vi "HandleObservationAsync.vi"(8 "error in (no error)":errorcluster, 10 "Acquisition.lvclass In":refnum<class "Acquisition.lvclass">, 11 "S4ACS_GUI in":refnum<class "S4GUI.lvclass">) -> (0 "error out":errorcluster, 2 "Acquisition.lvclass Out":refnum<class "Acquisition.lvclass">, 3 "S4ACS_GUI out":refnum<class "S4GUI.lvclass">)   [LabVIEW 2018, in "S4GUI.lvclass"]
uses:
  S4GUI.lvclass
  Acquisition/Acquisition.lvclass
  C:/Users/devstaff/sparc4/s4gui/Versao ZeroMQ REQ-REP/SPARC4_GUI -v1.0.0 - 20241216/Server/Server.lvclass
  S4GUI.lvclass/S4GUI.ctl
  Instrument/Instrument.lvclass/Instrument.ctl
  Device/Optics/Optics.lvclass/Optics.ctl
  Interface/Interface.lvclass/Interface.ctl
  Server/Server.lvclass/Server.ctl
  Device/Optics/Opt_Selector/Opt_Selector.lvclass
  C:/Users/devstaff/sparc4/s4gui/Versao ZeroMQ REQ-REP/SPARC4_GUI -v1.0.0 - 20241216/Device/Optics/Optics.lvclass
  Instrument/Instrument.lvclass
  StateMachine/State Machine.lvclass
  SyncBox/Sync Box.lvclass
  Trigger/Trigger.lvclass
  Channel/Channel.lvclass
  Interface/Interface.lvclass
  TelFocus/TelFocus.lvclass
  SecMirror/SecMirror.lvclass
  Device/Optics/Optics.lvclass
  Server/Server.lvclass
panel:
  out "time308":u32
  out "time307":u32
  out "time9":u32
  out "delay 89":u32
  out "time 10":u32
  out "time elapsed 2":u32
  out "time 8":u32
  out "delay 78":u32
  out "time7":u32
  out "time6":u32
  out "time5":u32
  out "delay 3-4":u32
  out "time4":u32
  out "time3":u32
  out "time 2":u32
  out "time1":u32
  # "ACS DELAY"
  # "WAVEPLATE DURATION"
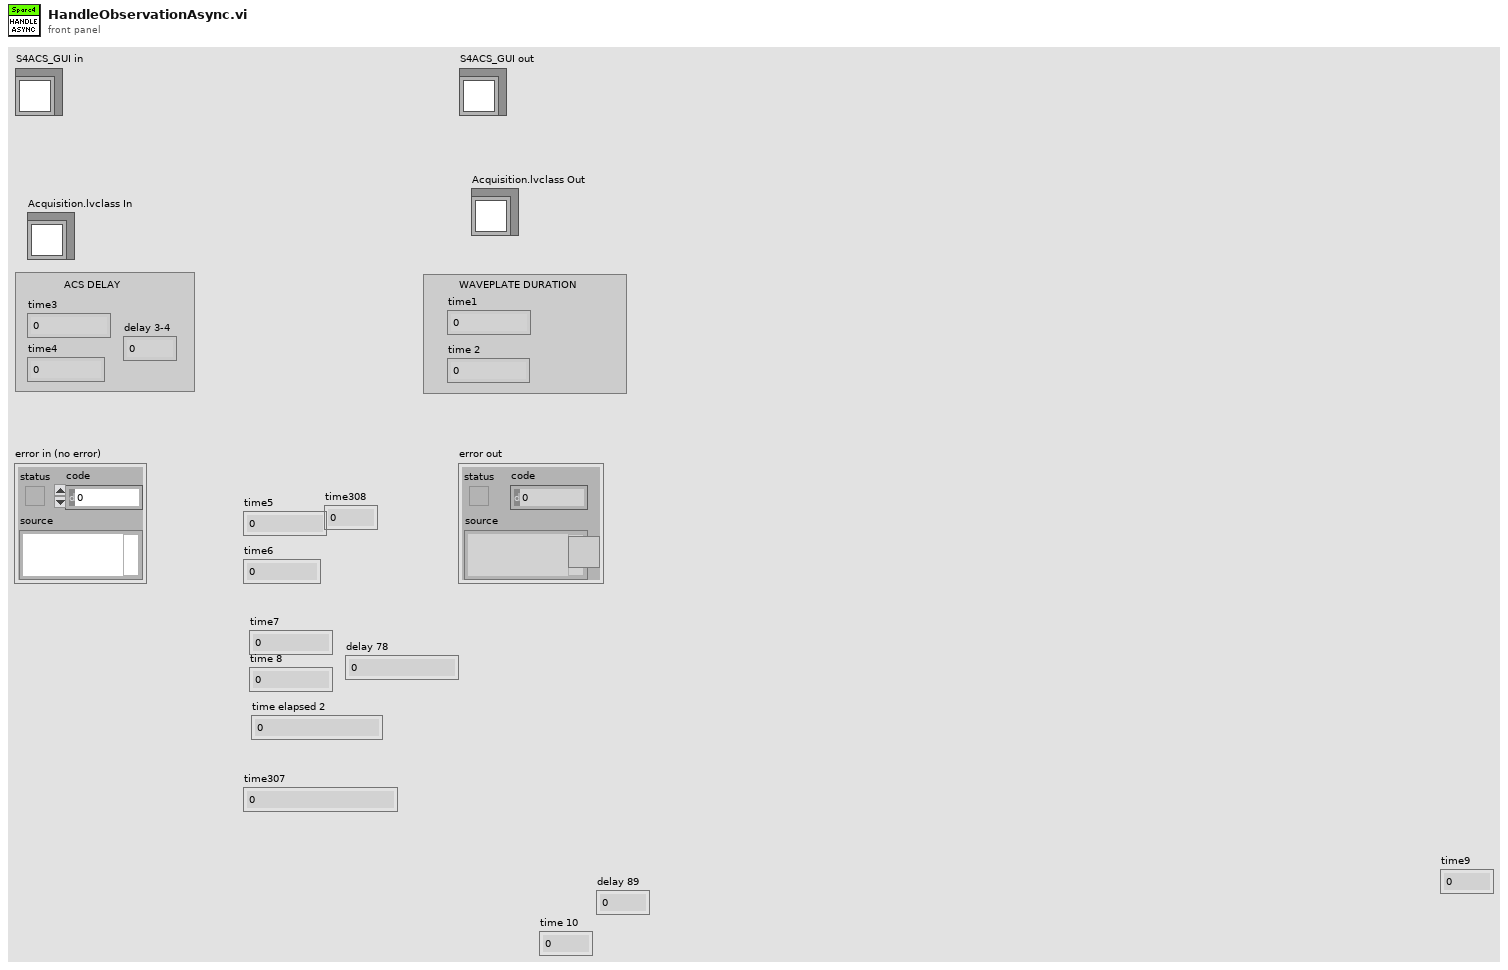
[diagram p1: front panel]
types:
  T1 = cluster{"ACQUISITION_MODE":u8, "TRIGGER_MODE":u8, "READ_MODE":u8, "PREAMP":u8, "READOUT_RATE":u8, "VERTICAL_SHIFT_SPEED":u8, "EM_MODE":u8, "EM_GAIN":u16, "SHUTTER_MODE":u8, "SHUTTER_TTL":u8, "SHUTTER_OPENING_TIME":u16, "SHUTTER_CLOSING_TIME":u16, "VBIN":u16, "HBIN":u16, "INITIAL_LINE":u16, "INITIAL_COLUMN":u16, "FINAL_LINE":u16, "FINAL_COLUMN":u16, "FRAME_TRANSFER":bool, "VERTICAL_CLOCK_VOLTAGE":u8, "AD_CHANNEL":u32}
  T2 = cluster{"Texp":dbl, "Nimages":u32, "InitialLine":u32, "FinalLine":u32, "InitialColumn":u32, "FinalColumn":u32, "EmGain":u32, "Cooler Off":bool, "CyclesDone":u32, "SequesDone":u32, "UsedDiskSpace":u16, "Error":bool}
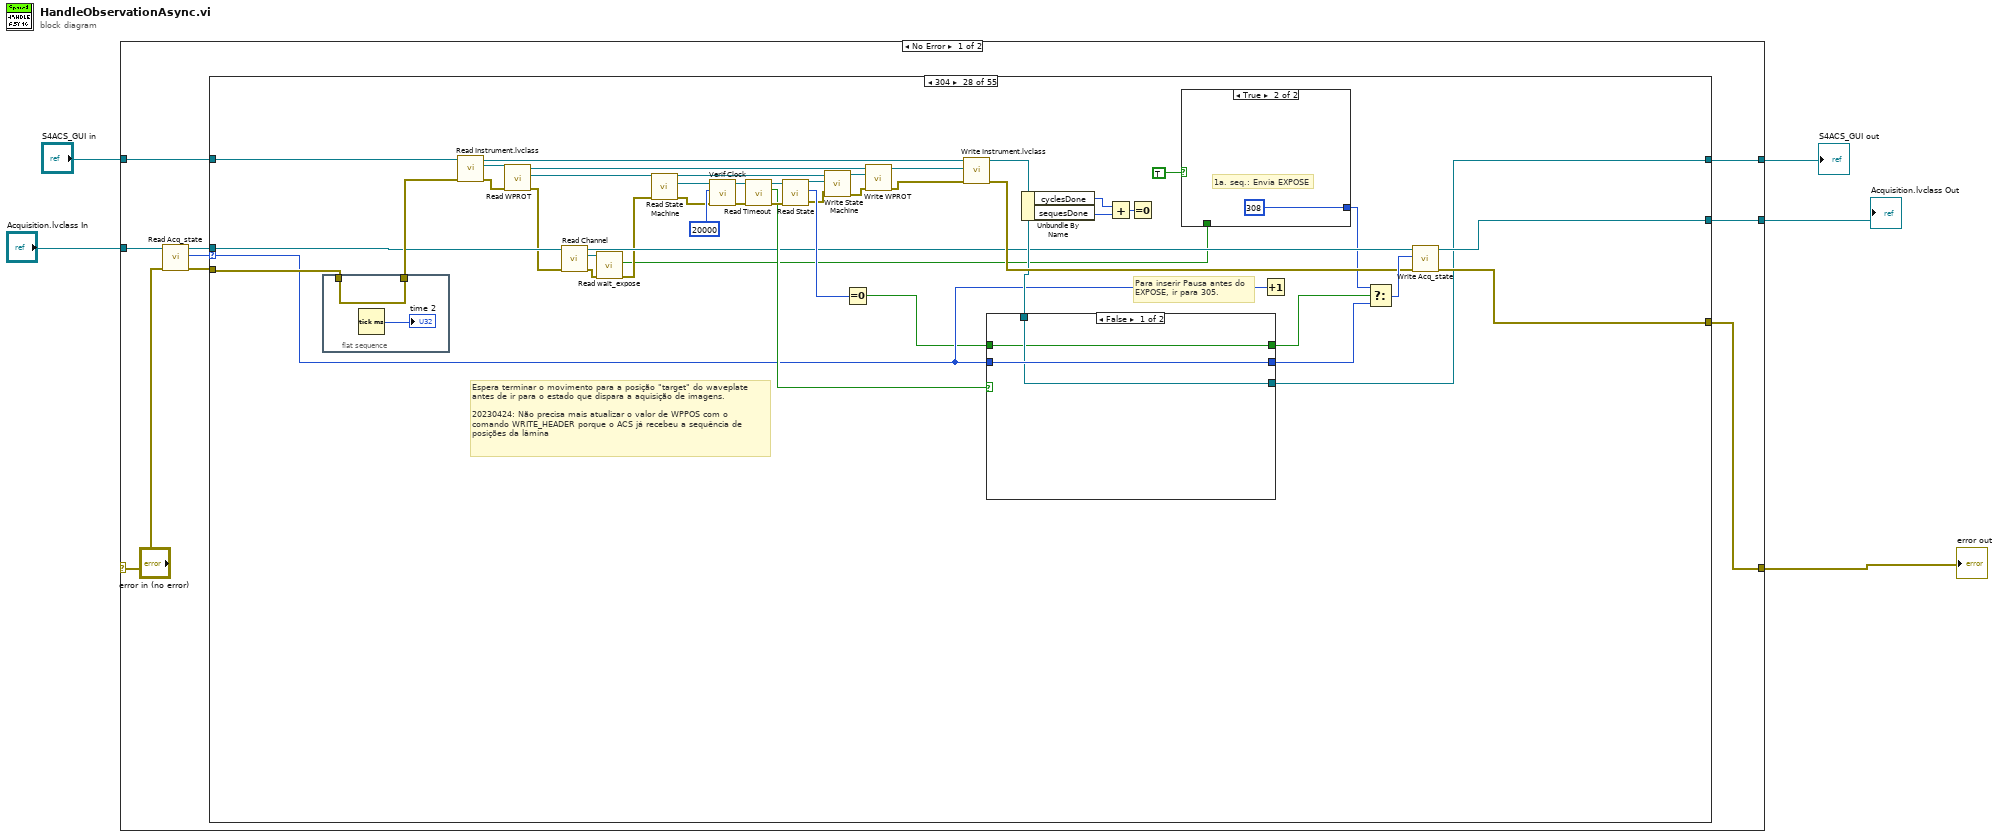
[diagram p0: block diagram]
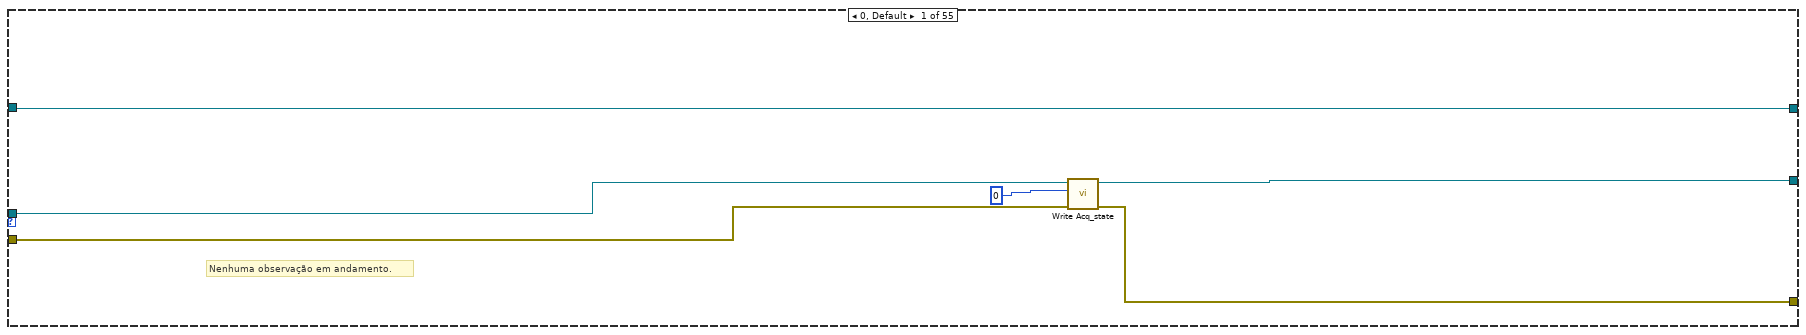
[diagram p2: hidden frame]
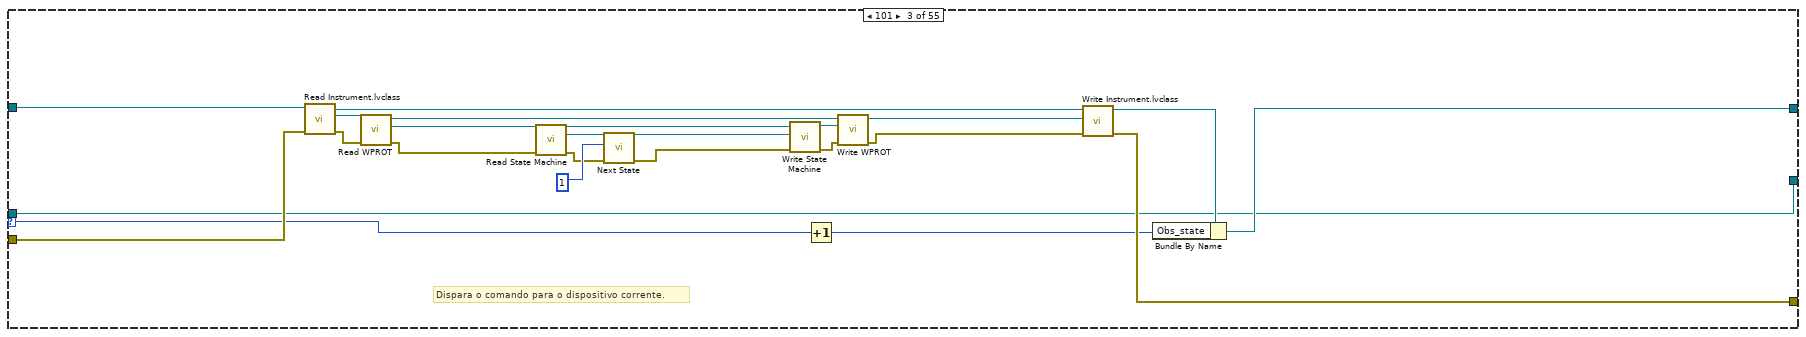
[diagram p4: hidden frame]
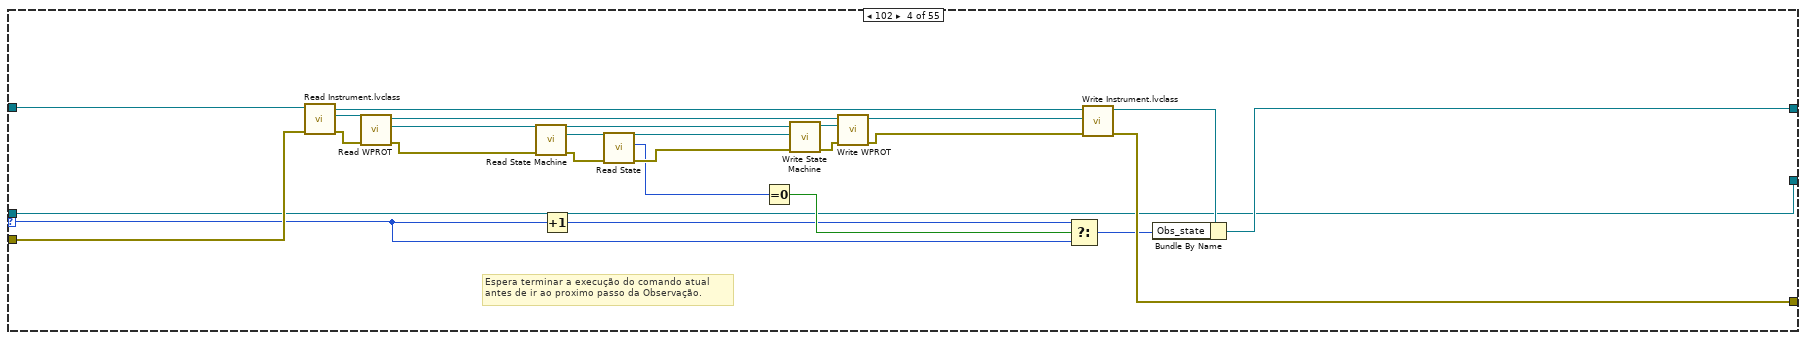
[diagram p5: hidden frame]
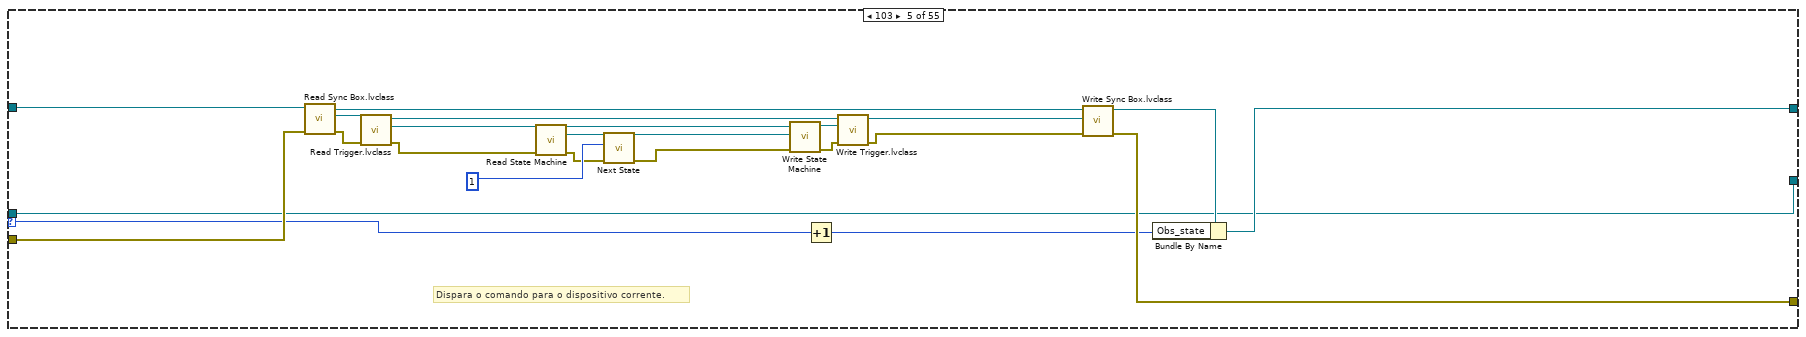
[diagram p6: hidden frame]
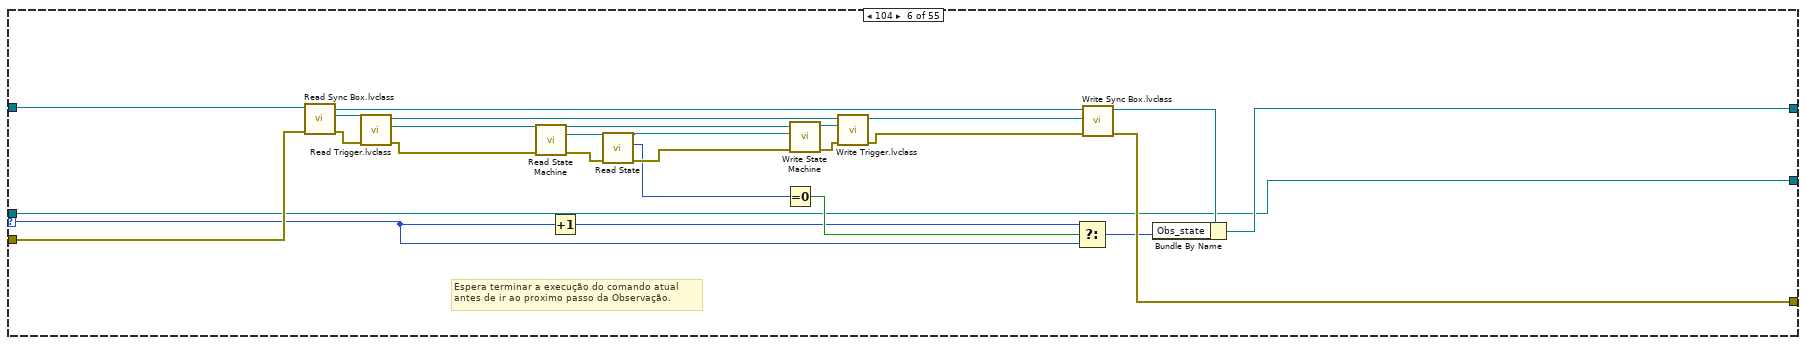
[diagram p7: hidden frame]
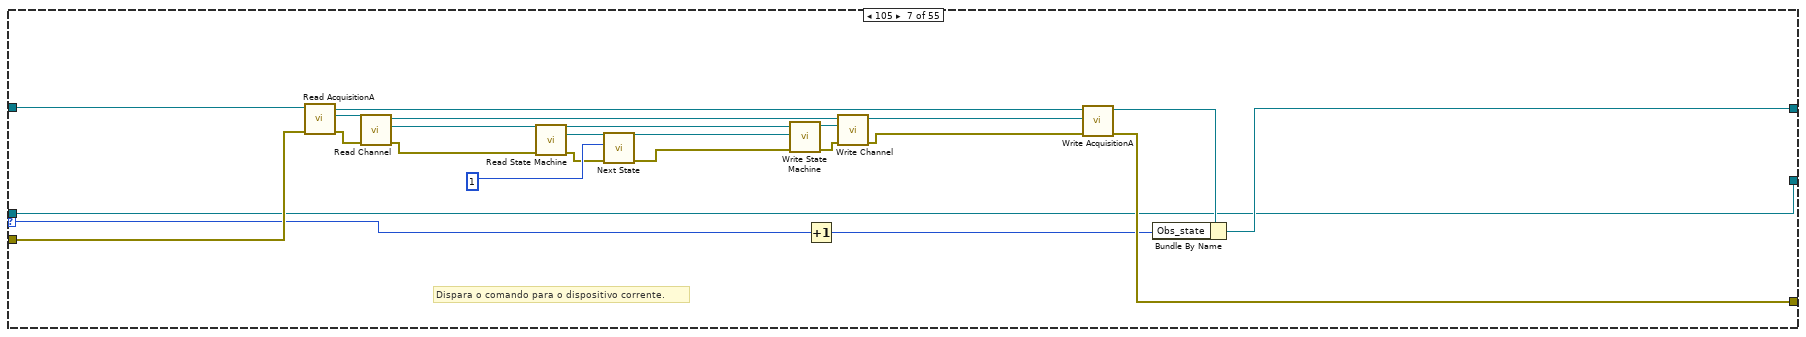
[diagram p8: hidden frame]
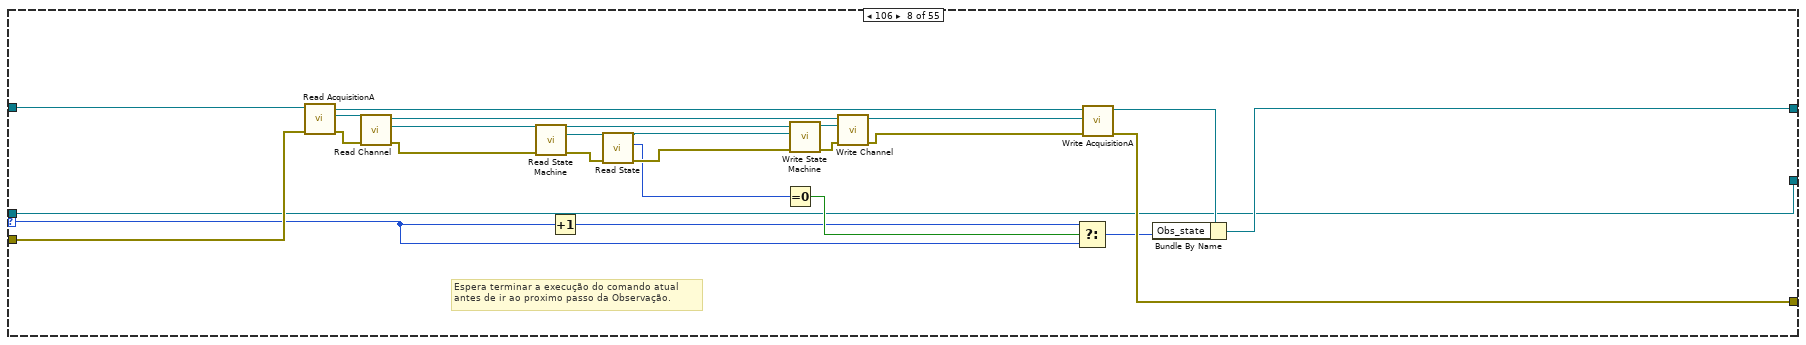
[diagram p9: hidden frame]
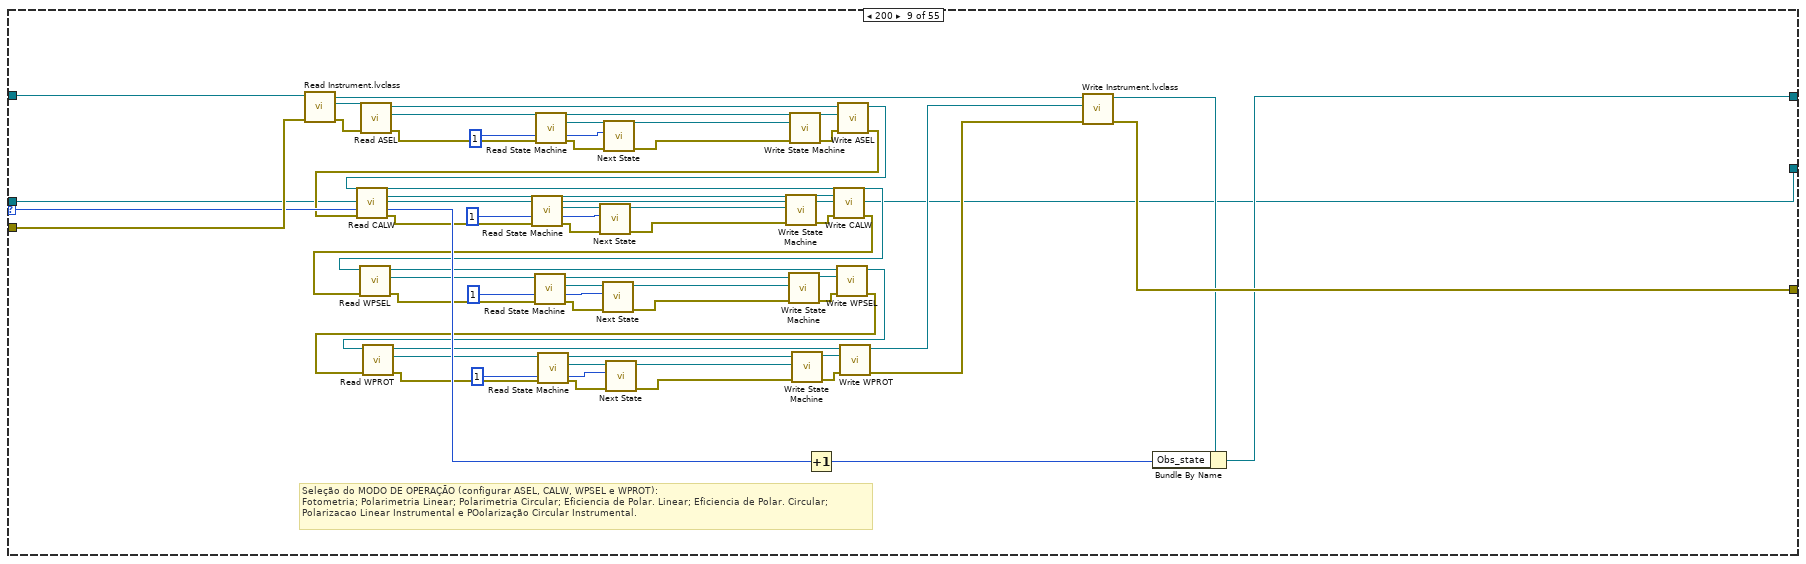
[diagram p10: hidden frame]
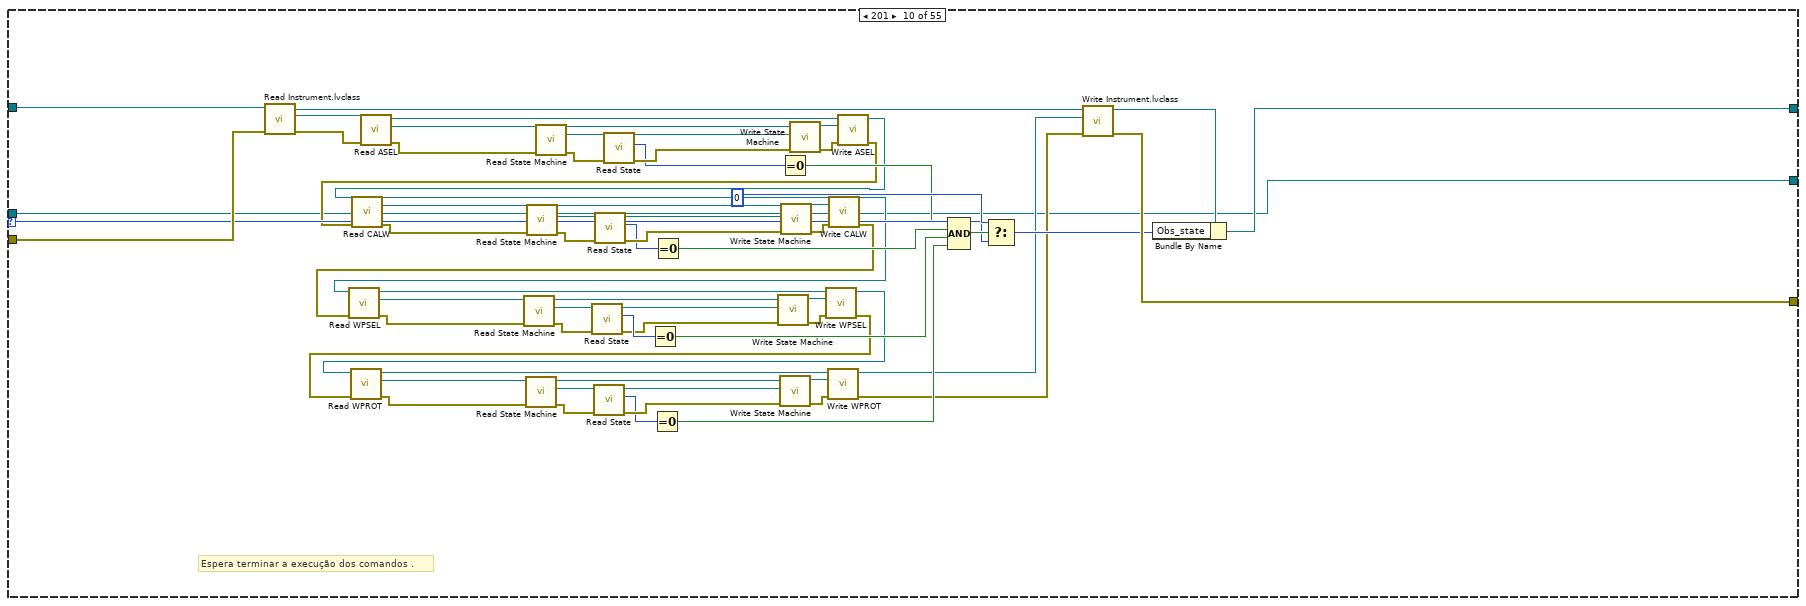
[diagram p11: hidden frame]
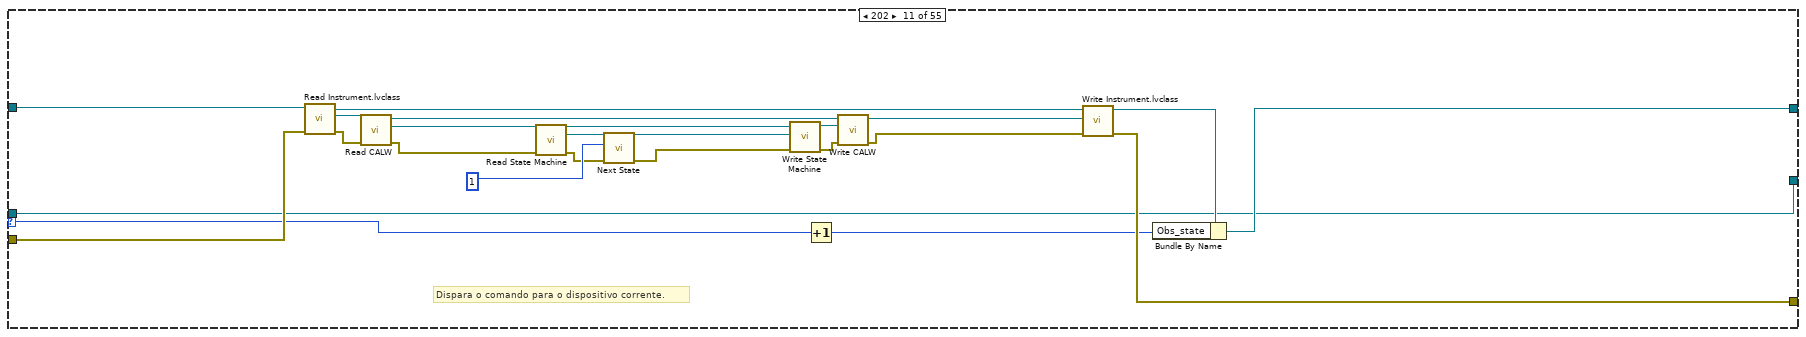
[diagram p12: hidden frame]
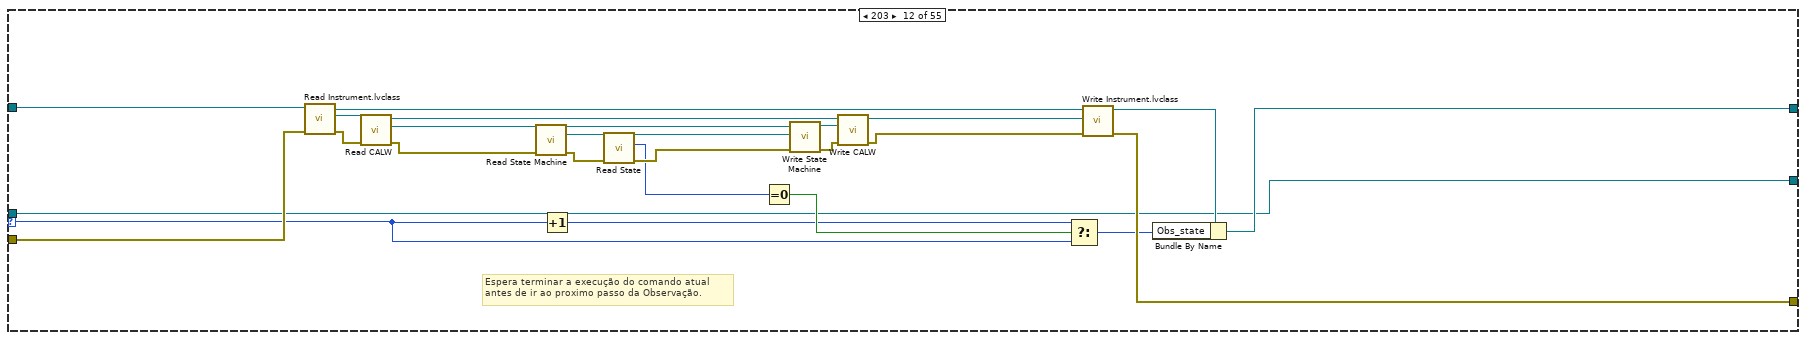
[diagram p13: hidden frame]
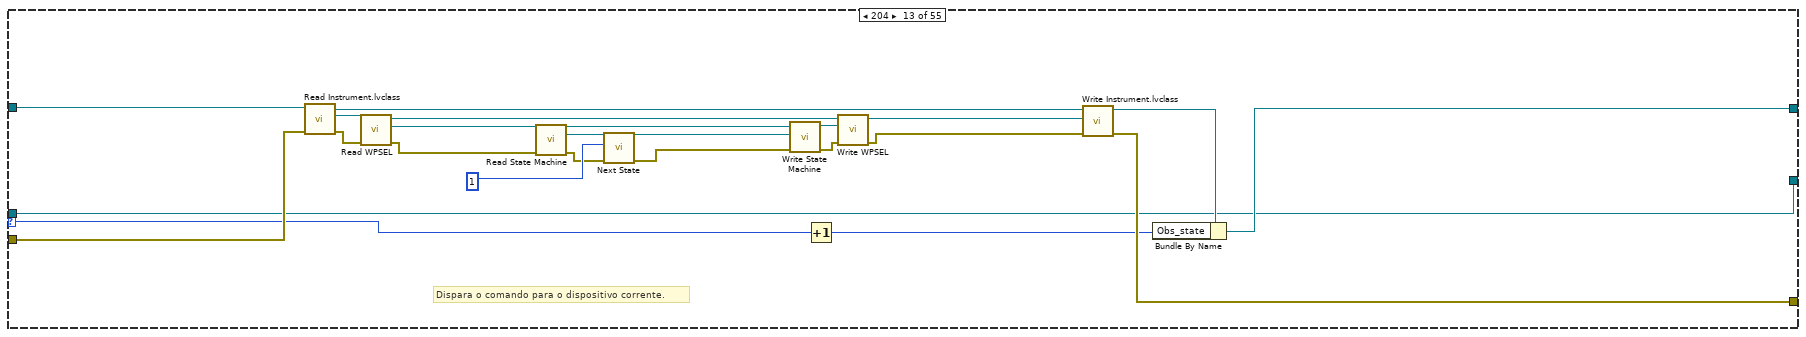
[diagram p14: hidden frame]
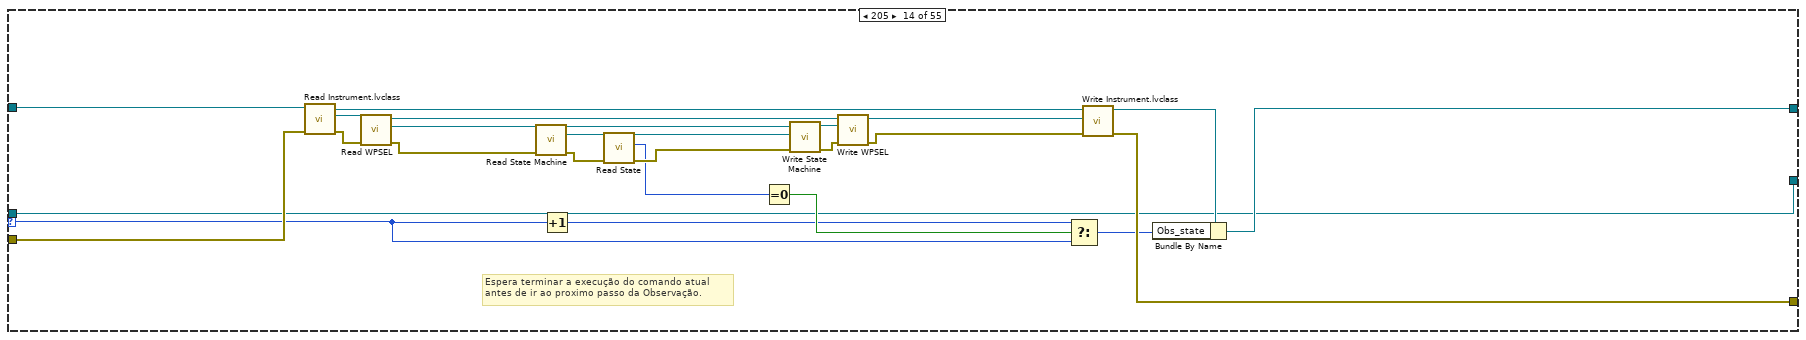
[diagram p15: hidden frame]
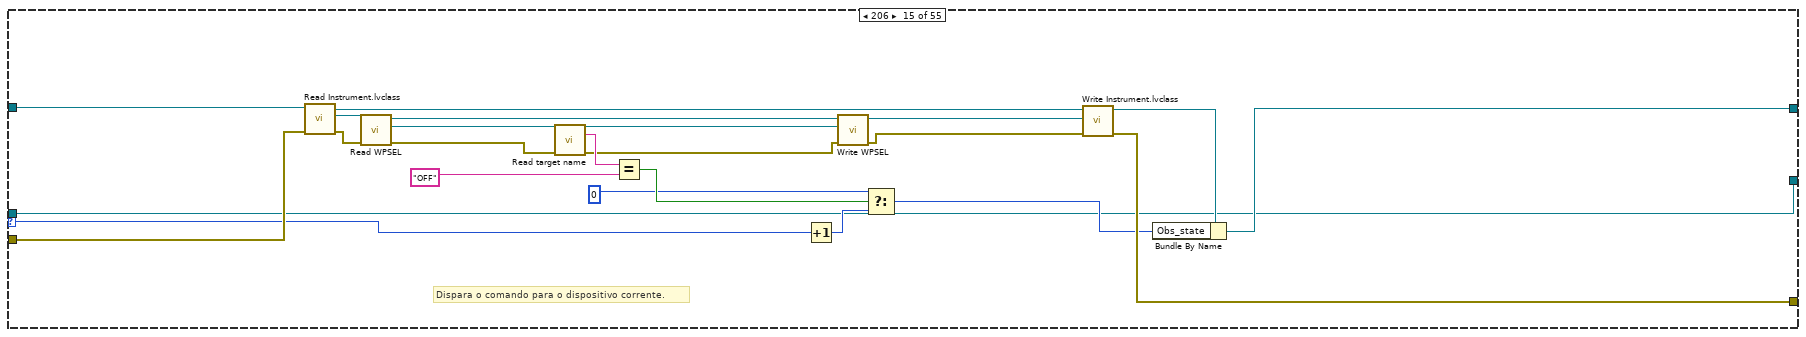
[diagram p16: hidden frame]
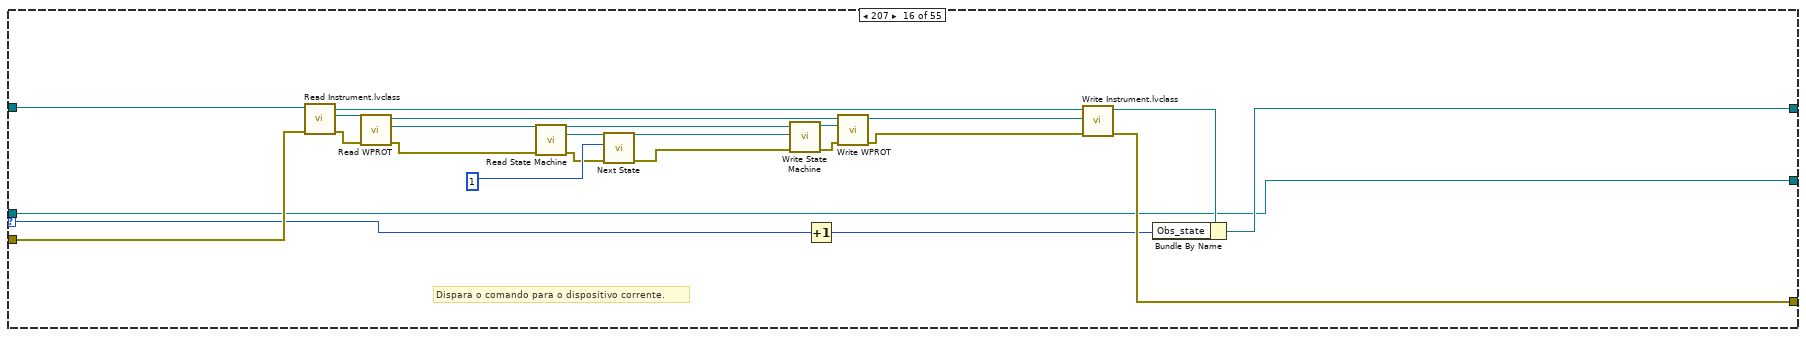
[diagram p17: hidden frame]
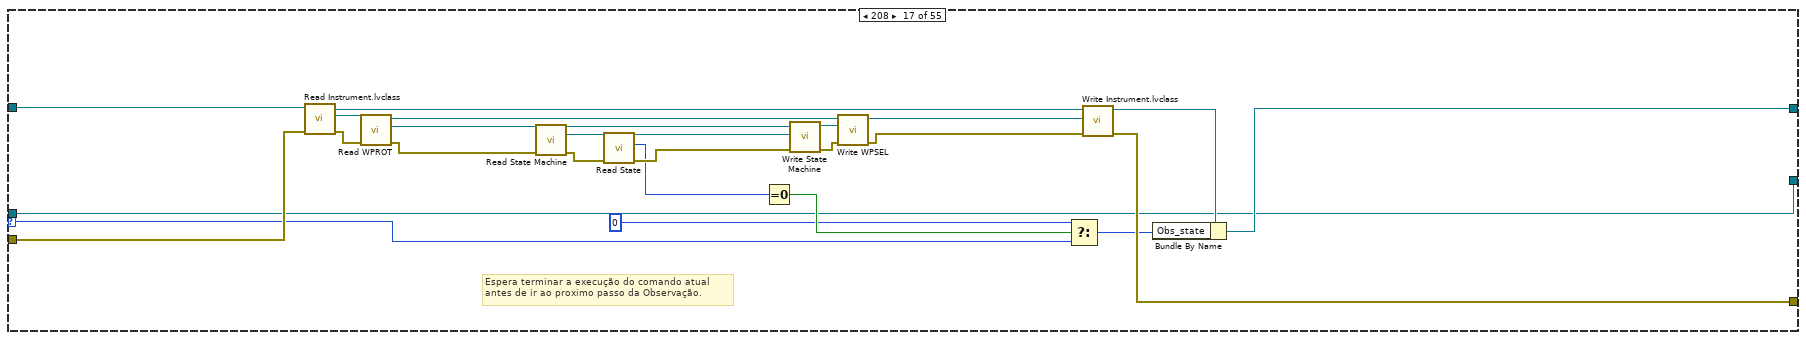
[diagram p18: hidden frame]
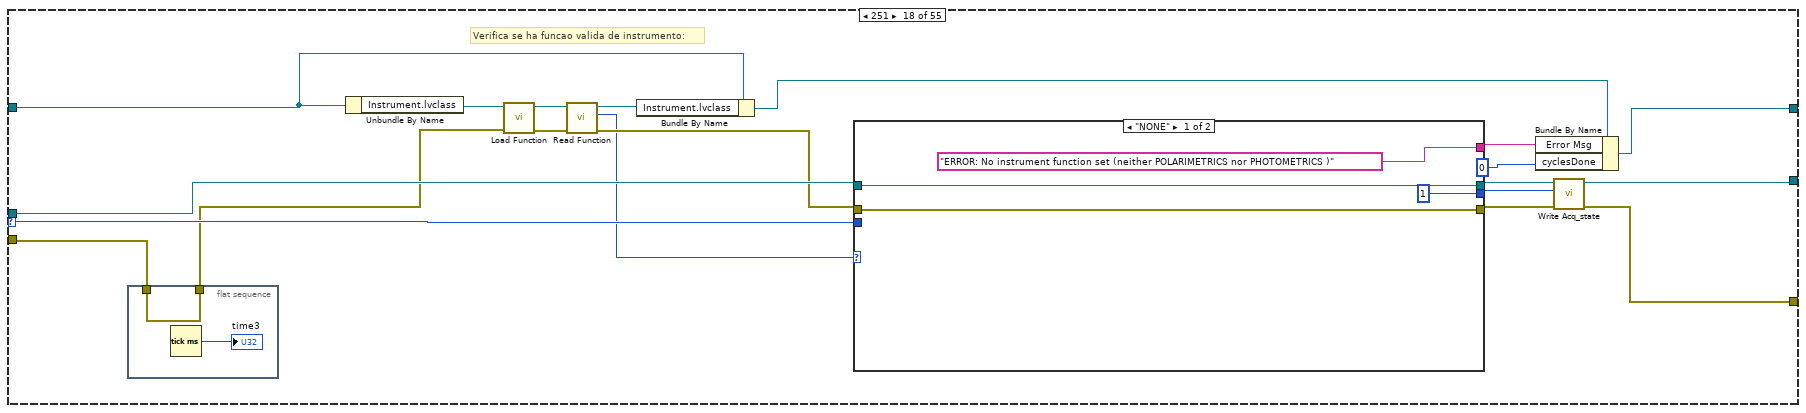
[diagram p19: hidden frame]
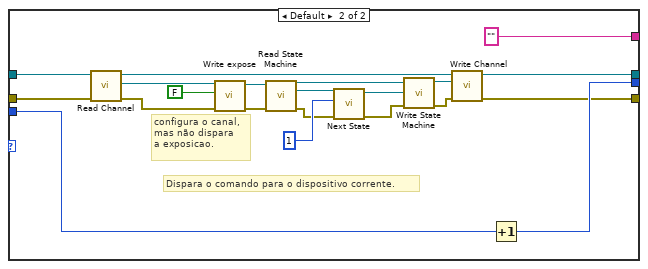
[diagram p20: hidden frame]
diagram:
  n1 = case shown="No Error" "error in (no error)" {
    selector: "error in (no error)" -> [w9 w1887]
    tunnel: [w15 w1887] -> w5
    tunnel: [w14 w1886] -> w3
    tunnel: "S4ACS_GUI in" -> [w13 w1886]
    tunnel: "Acquisition.lvclass In" -> [w12 w1885]
    tunnel: [w7 w1885] -> w1
    frame No Error {
      n2 = call-dynamic "Read Acq_state.vi"("error in (no error)"=w9, "Acquisition in"=w12) -> ("error out"=w8:errorcluster, "Acq_state"=w10:u32, "Acquisition out"=w11:refnum<class "Acquisition.lvclass">)  [unwired: 7 in]
      n3 = case shown="304" w10 {
        selector: w10 -> [_ _ w28 w51 w78 w101 w128 w151 w220 w284 w310 w333 w360 w383 w419 w433 w456 w499 w530 w603 w610 w653 w666 _ w758 w768 w824 w873 w935 w959 w1001 w1047 _ w1146 w1156 w1184 w1224 w1260 w1295 w1351 w1435 _ w1537 _ w1624 w1673 w1722 w1745 w1761 w1786 w1805 w1830 _ _ _]
        tunnel: w13 -> [w20 w24 w42 w68 w92 w118 w142 w168 w234 w302 w324 w350 w374 w400 w423 w447 w473 w484 w528 w573 w617 w634 w664 w733 w743 w767 w825 w909 w931 w949 w990 w1050 w1083 w1136 w1155 w1175 w1202 w1252 w1290 w1346 w1430 w1497 w1536 w1610 w1626 w1675 w1718 w1736 w1767 w1782 w1796 w1823 w1856 w1864 w1867]
        tunnel: [w20 w24 w26 w55 w76 w109 w126 w159 w218 w289 w308 w337 w358 w387 w418 w431 w460 w490 w527 w573 w617 w637 w663 w719 w748 w767 w791 w882 w931 w947 w980 w1049 w1082 w1134 w1155 w1174 w1201 w1254 w1289 w1347 w1431 w1493 w1536 w1610 w1623 w1659 w1718 w1740 w1767 w1782 w1800 w1823 w1851 w1864 w1869] -> w14
        tunnel: w8 -> [w19 w23 w41 w67 w91 w117 w141 w167 w233 w301 w323 w349 w373 w399 w422 w446 w472 w492 w540 w574 w611 w640 w676 w724 w742 w781 w788 w897 w936 w957 w985 w1056 w1087 w1144 w1169 w1172 w1198 w1245 w1280 w1331 w1415 w1508 w1540 w1604 w1625 w1674 w1720 w1750 w1764 w1784 w1813 w1843 w1855 w1863 w1866]
        tunnel: [w16 w23 w40 w66 w90 w116 w140 w166 w232 w300 w322 w348 w372 w398 w421 w445 w471 w493 w541 w607 w612 w641 w677 w726 w752 w779 w790 w901 w933 w952 w1004 w1054 w1084 w1139 w1167 w1178 w1222 w1255 w1300 w1334 w1418 w1513 w1538 w1611 w1617 w1655 w1711 w1746 w1765 w1778 w1809 w1839 w1849 w1863 w1868] -> w15
        tunnel: w11 -> [w18 w22 w25 w49 w75 w99 w125 w149 w175 w238 w307 w331 w357 w381 w407 w430 w454 w498 w545 w606 w618 w645 w681 w718 w757 w782 w793 w881 w937 w958 w971 w1057 w1086 w1145 w1170 w1183 w1200 w1250 w1283 w1332 w1416 w1509 w1541 w1605 w1621 w1658 w1721 w1751 w1762 w1785 w1814 w1844 w1854 w1862 w1865]
        tunnel: [w17 w22 w25 w49 w75 w99 w125 w149 w175 w238 w307 w331 w357 w381 w407 w430 w454 w495 w542 w608 w613 w642 w678 w725 w753 w780 w789 w900 w932 w953 w1005 w1055 w1085 w1140 w1168 w1182 w1223 w1259 w1301 w1350 w1434 w1514 w1539 w1612 w1620 w1656 w1715 w1747 w1766 w1779 w1810 w1840 w1850 w1862 w1865] -> w7
        frame 0, Default {
          # "Nenhuma observação em andamento."
          n4 = call-dynamic "Write Acq_state.vi"("error in (no error)"=w19, "Acq_state"=u32 0 ("Obs_state"), "Acquisition in"=w18) -> ("error out"=w16:errorcluster, "Acquisition out"=w17:refnum<class "Acquisition.lvclass">)  [unwired: 7 in]
        }
        frame 1 {
          # "Estado de erro!\nFica aqui até acionar STOP ou ABORT."
          # "Nenhuma observação em andamento."
        }
        frame 101 {
          # "Dispara o comando para o dispositivo corrente."
          n5 = call "Read Instrument.lvclass.vi"("error in (no error)"=w41, "S4ACS_GUI in"=w42) -> ("error out"=w47:errorcluster, "Instrument.lvclass"=w48:refnum<class "Instrument.lvclass">, "S4ACS_GUI out"=w44:refnum<class "S4GUI.lvclass">)  [unwired: 7 in]
          n6 = call "Read WPROT.vi"("error in (no error)"=w47, "Instrument in"=w48) -> ("error out"=w34:errorcluster, "Opt_Selector.lvclass"=w33:refnum<class "Opt_Selector.lvclass">, "Instrument out"=w46:refnum<class "Instrument.lvclass">)  [unwired: 7 in]
          n7 = call-dynamic "Read State Machine.vi"("error in (no error)"=w34, "Device in"=w33) -> ("error out"=w37:errorcluster, "State Machine.lvclass"=w39:refnum<class "State Machine.lvclass">, "Device out"=w31:refnum<class "Opt_Selector.lvclass">)  [unwired: 7 in]
          n8 = call "Next State.vi"("error in (no error)"=w37, "New_State"=1, "State Machine in"=w39) -> ("error out"=w36:errorcluster, "State Machine out"=w35:refnum<class "State Machine.lvclass">)  [unwired: 7 in]
          n9 = call-dynamic "Write State Machine.vi"("error in (no error)"=w36, "State Machine.lvclass"=w35, "Device in"=w31) -> ("error out"=w30:errorcluster, "Device out"=w32:refnum<class "Opt_Selector.lvclass">)  [unwired: 7 in]
          n10 = Increment(x=w28) -> (x+1=w27:u32)
          n11 = call "Write WPROT.vi"("error in (no error)"=w30, "Opt_Selector.lvclass"=w32, "Instrument in"=w46) -> ("error out"=w43:errorcluster, "Instrument out"=w45:refnum<class "Instrument.lvclass">)  [unwired: 7 in]
          n12 = call "Write Instrument.lvclass.vi"("error in (no error)"=w43, "Instrument.lvclass"=w45, "S4ACS_GUI in"=w44) -> ("error out"=w40:errorcluster, "S4ACS_GUI out"=w29:refnum<class "S4GUI.lvclass">)  [unwired: 7 in]
          n13 = Bundle By Name(cluster=w29, "Obs_state"=w27) -> (w26:refnum<class "S4GUI.lvclass">)
        }
        frame 102 {
          # "Espera terminar a execução do comando atual \nantes de ir ao proximo passo da Observação."
          n14 = call "Read Instrument.lvclass.vi"("error in (no error)"=w67, "S4ACS_GUI in"=w68) -> ("error out"=w73:errorcluster, "Instrument.lvclass"=w74:refnum<class "Instrument.lvclass">, "S4ACS_GUI out"=w70:refnum<class "S4GUI.lvclass">)  [unwired: 7 in]
          n15 = call "Read WPROT.vi"("error in (no error)"=w73, "Instrument in"=w74) -> ("error out"=w61:errorcluster, "Opt_Selector.lvclass"=w60:refnum<class "Opt_Selector.lvclass">, "Instrument out"=w72:refnum<class "Instrument.lvclass">)  [unwired: 7 in]
          n16 = call-dynamic "Read State Machine.vi"("error in (no error)"=w61, "Device in"=w60) -> ("error out"=w64:errorcluster, "State Machine.lvclass"=w65:refnum<class "State Machine.lvclass">, "Device out"=w58:refnum<class "Opt_Selector.lvclass">)  [unwired: 7 in]
          n17 = Increment(x=w51) -> (x+1=w50:u32)
          n18 = call-dynamic "Read State.vi"("error in (no error)"=w64, "State Machine in"=w65) -> ("error out"=w63:errorcluster, "State"=w53:i32, "State Machine out"=w62:refnum<class "State Machine.lvclass">)  [unwired: 7 in]
          n19 = Equal To 0?(x=w53) -> (x = 0?=w54:bool)
          n20 = call-dynamic "Write State Machine.vi"("error in (no error)"=w63, "State Machine.lvclass"=w62, "Device in"=w58) -> ("error out"=w57:errorcluster, "Device out"=w59:refnum<class "Opt_Selector.lvclass">)  [unwired: 7 in]
          n21 = call "Write WPROT.vi"("error in (no error)"=w57, "Opt_Selector.lvclass"=w59, "Instrument in"=w72) -> ("error out"=w69:errorcluster, "Instrument out"=w71:refnum<class "Instrument.lvclass">)  [unwired: 7 in]
          n22 = Select(t=w50, s=w54, f=w51) -> (s? t:f=w52:u32)
          n23 = call "Write Instrument.lvclass.vi"("error in (no error)"=w69, "Instrument.lvclass"=w71, "S4ACS_GUI in"=w70) -> ("error out"=w66:errorcluster, "S4ACS_GUI out"=w56:refnum<class "S4GUI.lvclass">)  [unwired: 7 in]
          n24 = Bundle By Name(cluster=w56, "Obs_state"=w52) -> (w55:refnum<class "S4GUI.lvclass">)
        }
        frame 103 {
          # "Dispara o comando para o dispositivo corrente."
          n25 = call-dynamic "Read Sync Box.lvclass.vi"("error in (no error)"=w91, "SPARC4_AC in"=w92) -> ("error out"=w97:errorcluster, "Sync Box.lvclass"=w98:refnum<class "Sync Box.lvclass">, "SPARC4_AC out"=w94:refnum<class "S4GUI.lvclass">)  [unwired: 7 in]
          n26 = call-dynamic "Read Trigger.lvclass.vi"("error in (no error)"=w97, "Sync Box in"=w98) -> ("error out"=w84:errorcluster, "Trigger.lvclass"=w83:refnum<class "Trigger.lvclass">, "Sync Box out"=w96:refnum<class "Sync Box.lvclass">)  [unwired: 7 in]
          n27 = call-dynamic "Read State Machine.vi"("error in (no error)"=w84, "Device in"=w83) -> ("error out"=w87:errorcluster, "State Machine.lvclass"=w89:refnum<class "State Machine.lvclass">, "Device out"=w81:refnum<class "Trigger.lvclass">)  [unwired: 7 in]
          n28 = call "Next State.vi"("error in (no error)"=w87, "New_State"=1, "State Machine in"=w89) -> ("error out"=w86:errorcluster, "State Machine out"=w85:refnum<class "State Machine.lvclass">)  [unwired: 7 in]
          n29 = call-dynamic "Write State Machine.vi"("error in (no error)"=w86, "State Machine.lvclass"=w85, "Device in"=w81) -> ("error out"=w80:errorcluster, "Device out"=w82:refnum<class "Trigger.lvclass">)  [unwired: 7 in]
          n30 = Increment(x=w78) -> (x+1=w77:u32)
          n31 = call-dynamic "Write Trigger.lvclass.vi"("error in (no error)"=w80, "Trigger.lvclass"=w82, "Sync Box in"=w96) -> ("error out"=w93:errorcluster, "Sync Box out"=w95:refnum<class "Sync Box.lvclass">)  [unwired: 7 in]
          n32 = call-dynamic "Write Sync Box.lvclass.vi"("error in (no error)"=w93, "Sync Box.lvclass"=w95, "SPARC4_AC in"=w94) -> ("error out"=w90:errorcluster, "SPARC4_AC out"=w79:refnum<class "S4GUI.lvclass">)  [unwired: 7 in]
          n33 = Bundle By Name(cluster=w79, "Obs_state"=w77) -> (w76:refnum<class "S4GUI.lvclass">)
        }
        frame 104 {
          # "Espera terminar a execução do comando atual \nantes de ir ao proximo passo da Observação."
          n34 = call-dynamic "Read Sync Box.lvclass.vi"("error in (no error)"=w117, "SPARC4_AC in"=w118) -> ("error out"=w123:errorcluster, "Sync Box.lvclass"=w124:refnum<class "Sync Box.lvclass">, "SPARC4_AC out"=w120:refnum<class "S4GUI.lvclass">)  [unwired: 7 in]
          n35 = call-dynamic "Read Trigger.lvclass.vi"("error in (no error)"=w123, "Sync Box in"=w124) -> ("error out"=w115:errorcluster, "Trigger.lvclass"=w114:refnum<class "Trigger.lvclass">, "Sync Box out"=w122:refnum<class "Sync Box.lvclass">)  [unwired: 7 in]
          n36 = call-dynamic "Read State Machine.vi"("error in (no error)"=w115, "Device in"=w114) -> ("error out"=w106:errorcluster, "State Machine.lvclass"=w108:refnum<class "State Machine.lvclass">, "Device out"=w112:refnum<class "Trigger.lvclass">)  [unwired: 7 in]
          n37 = Increment(x=w101) -> (x+1=w103:u32)
          n38 = call-dynamic "Read State.vi"("error in (no error)"=w106, "State Machine in"=w108) -> ("error out"=w105:errorcluster, "State"=w100:i32, "State Machine out"=w107:refnum<class "State Machine.lvclass">)  [unwired: 7 in]
          n39 = Equal To 0?(x=w100) -> (x = 0?=w104:bool)
          n40 = call-dynamic "Write State Machine.vi"("error in (no error)"=w105, "State Machine.lvclass"=w107, "Device in"=w112) -> ("error out"=w111:errorcluster, "Device out"=w113:refnum<class "Trigger.lvclass">)  [unwired: 7 in]
          n41 = call-dynamic "Write Trigger.lvclass.vi"("error in (no error)"=w111, "Trigger.lvclass"=w113, "Sync Box in"=w122) -> ("error out"=w119:errorcluster, "Sync Box out"=w121:refnum<class "Sync Box.lvclass">)  [unwired: 7 in]
          n42 = Select(t=w103, s=w104, f=w101) -> (s? t:f=w102:u32)
          n43 = call-dynamic "Write Sync Box.lvclass.vi"("error in (no error)"=w119, "Sync Box.lvclass"=w121, "SPARC4_AC in"=w120) -> ("error out"=w116:errorcluster, "SPARC4_AC out"=w110:refnum<class "S4GUI.lvclass">)  [unwired: 7 in]
          n44 = Bundle By Name(cluster=w110, "Obs_state"=w102) -> (w109:refnum<class "S4GUI.lvclass">)
        }
        frame 105 {
          # "Dispara o comando para o dispositivo corrente."
          n45 = call-dynamic "Read AcquisitionA.vi"("error in (no error)"=w141, "S4ACS_GUI in"=w142) -> ("error out"=w147:errorcluster, "Acquisition.lvclass"=w148:refnum<class "Acquisition.lvclass">, "S4ACS_GUI out"=w144:refnum<class "S4GUI.lvclass">)  [unwired: 7 in]
          n46 = call-dynamic "Read Channel.vi"("error in (no error)"=w147, "Acquisition in"=w148) -> ("error out"=w134:errorcluster, "Channel.lvclass"=w133:refnum<class "Channel.lvclass">, "Acquisition out"=w146:refnum<class "Acquisition.lvclass">)  [unwired: 7 in]
          n47 = call-dynamic "Read State Machine.vi"("error in (no error)"=w134, "Device in"=w133) -> ("error out"=w137:errorcluster, "State Machine.lvclass"=w139:refnum<class "State Machine.lvclass">, "Device out"=w131:refnum<class "Channel.lvclass">)  [unwired: 7 in]
          n48 = call "Next State.vi"("error in (no error)"=w137, "New_State"=1, "State Machine in"=w139) -> ("error out"=w136:errorcluster, "State Machine out"=w135:refnum<class "State Machine.lvclass">)  [unwired: 7 in]
          n49 = call-dynamic "Write State Machine.vi"("error in (no error)"=w136, "State Machine.lvclass"=w135, "Device in"=w131) -> ("error out"=w130:errorcluster, "Device out"=w132:refnum<class "Channel.lvclass">)  [unwired: 7 in]
          n50 = Increment(x=w128) -> (x+1=w127:u32)
          n51 = call-dynamic "Write Channel.vi"("error in (no error)"=w130, "Channel.lvclass"=w132, "Acquisition in"=w146) -> ("error out"=w143:errorcluster, "Acquisition out"=w145:refnum<class "Acquisition.lvclass">)  [unwired: 7 in]
          n52 = call-dynamic "Write AcquisitionA.vi"("error in (no error)"=w143, "Acquisition.lvclass"=w145, "S4ACS_GUI in"=w144) -> ("error out"=w140:errorcluster, "S4ACS_GUI out"=w129:refnum<class "S4GUI.lvclass">)  [unwired: 7 in]
          n53 = Bundle By Name(cluster=w129, "Obs_state"=w127) -> (w126:refnum<class "S4GUI.lvclass">)
        }
        frame 106 {
          # "Espera terminar a execução do comando atual \nantes de ir ao proximo passo da Observação."
          n54 = call-dynamic "Read AcquisitionA.vi"("error in (no error)"=w167, "S4ACS_GUI in"=w168) -> ("error out"=w173:errorcluster, "Acquisition.lvclass"=w174:refnum<class "Acquisition.lvclass">, "S4ACS_GUI out"=w170:refnum<class "S4GUI.lvclass">)  [unwired: 7 in]
          n55 = call-dynamic "Read Channel.vi"("error in (no error)"=w173, "Acquisition in"=w174) -> ("error out"=w165:errorcluster, "Channel.lvclass"=w164:refnum<class "Channel.lvclass">, "Acquisition out"=w172:refnum<class "Acquisition.lvclass">)  [unwired: 7 in]
          n56 = call-dynamic "Read State Machine.vi"("error in (no error)"=w165, "Device in"=w164) -> ("error out"=w156:errorcluster, "State Machine.lvclass"=w158:refnum<class "State Machine.lvclass">, "Device out"=w162:refnum<class "Channel.lvclass">)  [unwired: 7 in]
          n57 = Increment(x=w151) -> (x+1=w153:u32)
          n58 = call-dynamic "Read State.vi"("error in (no error)"=w156, "State Machine in"=w158) -> ("error out"=w155:errorcluster, "State"=w150:i32, "State Machine out"=w157:refnum<class "State Machine.lvclass">)  [unwired: 7 in]
          n59 = Equal To 0?(x=w150) -> (x = 0?=w154:bool)
          n60 = call-dynamic "Write State Machine.vi"("error in (no error)"=w155, "State Machine.lvclass"=w157, "Device in"=w162) -> ("error out"=w161:errorcluster, "Device out"=w163:refnum<class "Channel.lvclass">)  [unwired: 7 in]
          n61 = call-dynamic "Write Channel.vi"("error in (no error)"=w161, "Channel.lvclass"=w163, "Acquisition in"=w172) -> ("error out"=w169:errorcluster, "Acquisition out"=w171:refnum<class "Acquisition.lvclass">)  [unwired: 7 in]
          n62 = Select(t=w153, s=w154, f=w151) -> (s? t:f=w152:u32)
          n63 = call-dynamic "Write AcquisitionA.vi"("error in (no error)"=w169, "Acquisition.lvclass"=w171, "S4ACS_GUI in"=w170) -> ("error out"=w166:errorcluster, "S4ACS_GUI out"=w160:refnum<class "S4GUI.lvclass">)  [unwired: 7 in]
          n64 = Bundle By Name(cluster=w160, "Obs_state"=w152) -> (w159:refnum<class "S4GUI.lvclass">)
        }
        frame 200 {
          # "Seleção do MODO DE OPERAÇÃO (configurar ASEL, CALW, WPSEL e WPROT): \nFotometria; Polarimetria Linear; Polarimetria Circular; Eficiencia de Polar. Linear; Eficiencia de Polar. Circular;\nPolarizacao Linear Instrumental e POolarização Circular Instrumental."
          n65 = call "Read Instrument.lvclass.vi"("error in (no error)"=w233, "S4ACS_GUI in"=w234) -> ("error out"=w237:errorcluster, "Instrument.lvclass"=w197:refnum<class "Instrument.lvclass">, "S4ACS_GUI out"=w235:refnum<class "S4GUI.lvclass">)  [unwired: 7 in]
          n66 = call "Read ASEL.vi"("error in (no error)"=w237, "Instrument in"=w197) -> ("error out"=w226:errorcluster, "Opt_Selector.lvclass"=w225:refnum<class "Opt_Selector.lvclass">, "Instrument out"=w236:refnum<class "Instrument.lvclass">)  [unwired: 7 in]
          n67 = call-dynamic "Read State Machine.vi"("error in (no error)"=w226, "Device in"=w225) -> ("error out"=w229:errorcluster, "State Machine.lvclass"=w231:refnum<class "State Machine.lvclass">, "Device out"=w223:refnum<class "Opt_Selector.lvclass">)  [unwired: 7 in]
          n68 = call "Next State.vi"("error in (no error)"=w229, "New_State"=1, "State Machine in"=w231) -> ("error out"=w228:errorcluster, "State Machine out"=w227:refnum<class "State Machine.lvclass">)  [unwired: 7 in]
          n69 = call-dynamic "Write State Machine.vi"("error in (no error)"=w228, "State Machine.lvclass"=w227, "Device in"=w223) -> ("error out"=w222:errorcluster, "Device out"=w224:refnum<class "Opt_Selector.lvclass">)  [unwired: 7 in]
          n70 = Increment(x=w220) -> (x+1=w219:u32)
          n71 = call "Write ASEL.vi"("error in (no error)"=w222, "Opt_Selector.lvclass"=w224, "Instrument in"=w236) -> ("error out"=w178:errorcluster, "Instrument out"=w196:refnum<class "Instrument.lvclass">)  [unwired: 7 in]
          n72 = call "Read CALW.vi"("error in (no error)"=w178, "Instrument in"=w196) -> ("error out"=w213:errorcluster, "Opt_Selector.lvclass"=w214:refnum<class "Opt_Selector.lvclass">, "Instrument out"=w195:refnum<class "Instrument.lvclass">)  [unwired: 7 in]
          n73 = call-dynamic "Read State Machine.vi"("error in (no error)"=w213, "Device in"=w214) -> ("error out"=w210:errorcluster, "State Machine.lvclass"=w208:refnum<class "State Machine.lvclass">, "Device out"=w216:refnum<class "Opt_Selector.lvclass">)  [unwired: 7 in]
          n74 = call "Next State.vi"("error in (no error)"=w210, "New_State"=1, "State Machine in"=w208) -> ("error out"=w211:errorcluster, "State Machine out"=w212:refnum<class "State Machine.lvclass">)  [unwired: 7 in]
          n75 = call-dynamic "Write State Machine.vi"("error in (no error)"=w211, "State Machine.lvclass"=w212, "Device in"=w216) -> ("error out"=w217:errorcluster, "Device out"=w215:refnum<class "Opt_Selector.lvclass">)  [unwired: 7 in]
          n76 = call "Write CALW.vi"("error in (no error)"=w217, "Opt_Selector.lvclass"=w215, "Instrument in"=w195) -> ("error out"=w177:errorcluster, "Instrument out"=w194:refnum<class "Instrument.lvclass">)  [unwired: 7 in]
          n77 = call "Read WPSEL.vi"("error in (no error)"=w177, "Instrument in"=w194) -> ("error out"=w202:errorcluster, "Opt_Selector.lvclass"=w201:refnum<class "Opt_Selector.lvclass">, "Instrument out"=w193:refnum<class "Instrument.lvclass">)  [unwired: 7 in]
          n78 = call-dynamic "Read State Machine.vi"("error in (no error)"=w202, "Device in"=w201) -> ("error out"=w205:errorcluster, "State Machine.lvclass"=w207:refnum<class "State Machine.lvclass">, "Device out"=w199:refnum<class "Opt_Selector.lvclass">)  [unwired: 7 in]
          n79 = call "Next State.vi"("error in (no error)"=w205, "New_State"=1, "State Machine in"=w207) -> ("error out"=w204:errorcluster, "State Machine out"=w203:refnum<class "State Machine.lvclass">)  [unwired: 7 in]
          n80 = call-dynamic "Write State Machine.vi"("error in (no error)"=w204, "State Machine.lvclass"=w203, "Device in"=w199) -> ("error out"=w198:errorcluster, "Device out"=w200:refnum<class "Opt_Selector.lvclass">)  [unwired: 7 in]
          n81 = call "Write WPSEL.vi"("error in (no error)"=w198, "Opt_Selector.lvclass"=w200, "Instrument in"=w193) -> ("error out"=w176:errorcluster, "Instrument out"=w182:refnum<class "Instrument.lvclass">)  [unwired: 7 in]
          n82 = call "Read WPROT.vi"("error in (no error)"=w176, "Instrument in"=w182) -> ("error out"=w188:errorcluster, "Opt_Selector.lvclass"=w189:refnum<class "Opt_Selector.lvclass">, "Instrument out"=w181:refnum<class "Instrument.lvclass">)  [unwired: 7 in]
          n83 = call-dynamic "Read State Machine.vi"("error in (no error)"=w188, "Device in"=w189) -> ("error out"=w185:errorcluster, "State Machine.lvclass"=w183:refnum<class "State Machine.lvclass">, "Device out"=w191:refnum<class "Opt_Selector.lvclass">)  [unwired: 7 in]
          n84 = call "Next State.vi"("error in (no error)"=w185, "New_State"=1, "State Machine in"=w183) -> ("error out"=w186:errorcluster, "State Machine out"=w187:refnum<class "State Machine.lvclass">)  [unwired: 7 in]
          n85 = call-dynamic "Write State Machine.vi"("error in (no error)"=w186, "State Machine.lvclass"=w187, "Device in"=w191) -> ("error out"=w192:errorcluster, "Device out"=w190:refnum<class "Opt_Selector.lvclass">)  [unwired: 7 in]
          n86 = call "Write WPROT.vi"("error in (no error)"=w192, "Opt_Selector.lvclass"=w190, "Instrument in"=w181) -> ("error out"=w179:errorcluster, "Instrument out"=w180:refnum<class "Instrument.lvclass">)  [unwired: 7 in]
          n87 = call "Write Instrument.lvclass.vi"("error in (no error)"=w179, "Instrument.lvclass"=w180, "S4ACS_GUI in"=w235) -> ("error out"=w232:errorcluster, "S4ACS_GUI out"=w221:refnum<class "S4GUI.lvclass">)  [unwired: 7 in]
          n88 = Bundle By Name(cluster=w221, "Obs_state"=w219) -> (w218:refnum<class "S4GUI.lvclass">)
        }
        frame 201 {
          # "Espera terminar a execução dos comandos ."
          n89 = call "Read Instrument.lvclass.vi"("error in (no error)"=w301, "S4ACS_GUI in"=w302) -> ("error out"=w305:errorcluster, "Instrument.lvclass"=w306:refnum<class "Instrument.lvclass">, "S4ACS_GUI out"=w303:refnum<class "S4GUI.lvclass">)  [unwired: 7 in]
          n90 = call "Read ASEL.vi"("error in (no error)"=w305, "Instrument in"=w306) -> ("error out"=w295:errorcluster, "Opt_Selector.lvclass"=w294:refnum<class "Opt_Selector.lvclass">, "Instrument out"=w304:refnum<class "Instrument.lvclass">)  [unwired: 7 in]
          n91 = call-dynamic "Read State Machine.vi"("error in (no error)"=w295, "Device in"=w294) -> ("error out"=w298:errorcluster, "State Machine.lvclass"=w299:refnum<class "State Machine.lvclass">, "Device out"=w292:refnum<class "Opt_Selector.lvclass">)  [unwired: 7 in]
          n92 = call-dynamic "Read State.vi"("error in (no error)"=w298, "State Machine in"=w299) -> ("error out"=w297:errorcluster, "State"=w288:i32, "State Machine out"=w296:refnum<class "State Machine.lvclass">)  [unwired: 7 in]
          n93 = Equal To 0?(x=w288) -> (x = 0?=w283:bool)
          n94 = call-dynamic "Write State Machine.vi"("error in (no error)"=w297, "State Machine.lvclass"=w296, "Device in"=w292) -> ("error out"=w291:errorcluster, "Device out"=w293:refnum<class "Opt_Selector.lvclass">)  [unwired: 7 in]
          n95 = call "Write ASEL.vi"("error in (no error)"=w291, "Opt_Selector.lvclass"=w293, "Instrument in"=w304) -> ("error out"=w245:errorcluster, "Instrument out"=w246:refnum<class "Instrument.lvclass">)  [unwired: 7 in]
          n96 = call "Read CALW.vi"("error in (no error)"=w245, "Instrument in"=w246) -> ("error out"=w278:errorcluster, "Opt_Selector.lvclass"=w279:refnum<class "Opt_Selector.lvclass">, "Instrument out"=w249:refnum<class "Instrument.lvclass">)  [unwired: 7 in]
          n97 = call-dynamic "Read State Machine.vi"("error in (no error)"=w278, "Device in"=w279) -> ("error out"=w275:errorcluster, "State Machine.lvclass"=w274:refnum<class "State Machine.lvclass">, "Device out"=w281:refnum<class "Opt_Selector.lvclass">)  [unwired: 7 in]
          n98 = call-dynamic "Read State.vi"("error in (no error)"=w275, "State Machine in"=w274) -> ("error out"=w276:errorcluster, "State"=w273:i32, "State Machine out"=w277:refnum<class "State Machine.lvclass">)  [unwired: 7 in]
          n99 = Equal To 0?(x=w273) -> (x = 0?=w272:bool)
          n100 = call-dynamic "Write State Machine.vi"("error in (no error)"=w276, "State Machine.lvclass"=w277, "Device in"=w281) -> ("error out"=w282:errorcluster, "Device out"=w280:refnum<class "Opt_Selector.lvclass">)  [unwired: 7 in]
          n101 = call "Write CALW.vi"("error in (no error)"=w282, "Opt_Selector.lvclass"=w280, "Instrument in"=w249) -> ("error out"=w243:errorcluster, "Instrument out"=w244:refnum<class "Instrument.lvclass">)  [unwired: 7 in]
          n102 = call "Read WPSEL.vi"("error in (no error)"=w243, "Instrument in"=w244) -> ("error out"=w266:errorcluster, "Opt_Selector.lvclass"=w265:refnum<class "Opt_Selector.lvclass">, "Instrument out"=w248:refnum<class "Instrument.lvclass">)  [unwired: 7 in]
          n103 = call-dynamic "Read State Machine.vi"("error in (no error)"=w266, "Device in"=w265) -> ("error out"=w269:errorcluster, "State Machine.lvclass"=w270:refnum<class "State Machine.lvclass">, "Device out"=w263:refnum<class "Opt_Selector.lvclass">)  [unwired: 7 in]
          n104 = call-dynamic "Read State.vi"("error in (no error)"=w269, "State Machine in"=w270) -> ("error out"=w268:errorcluster, "State"=w271:i32, "State Machine out"=w267:refnum<class "State Machine.lvclass">)  [unwired: 7 in]
          n105 = Equal To 0?(x=w271) -> (x = 0?=w251:bool)
          n106 = call-dynamic "Write State Machine.vi"("error in (no error)"=w268, "State Machine.lvclass"=w267, "Device in"=w263) -> ("error out"=w262:errorcluster, "Device out"=w264:refnum<class "Opt_Selector.lvclass">)  [unwired: 7 in]
          n107 = call "Write WPSEL.vi"("error in (no error)"=w262, "Opt_Selector.lvclass"=w264, "Instrument in"=w248) -> ("error out"=w241:errorcluster, "Instrument out"=w242:refnum<class "Instrument.lvclass">)  [unwired: 7 in]
          n108 = call "Read WPROT.vi"("error in (no error)"=w241, "Instrument in"=w242) -> ("error out"=w257:errorcluster, "Opt_Selector.lvclass"=w258:refnum<class "Opt_Selector.lvclass">, "Instrument out"=w247:refnum<class "Instrument.lvclass">)  [unwired: 7 in]
          n109 = call-dynamic "Read State Machine.vi"("error in (no error)"=w257, "Device in"=w258) -> ("error out"=w254:errorcluster, "State Machine.lvclass"=w253:refnum<class "State Machine.lvclass">, "Device out"=w260:refnum<class "Opt_Selector.lvclass">)  [unwired: 7 in]
          n110 = call-dynamic "Read State.vi"("error in (no error)"=w254, "State Machine in"=w253) -> ("error out"=w255:errorcluster, "State"=w252:i32, "State Machine out"=w256:refnum<class "State Machine.lvclass">)  [unwired: 7 in]
          n111 = Equal To 0?(x=w252) -> (x = 0?=w250:bool)
          n112 = call-dynamic "Write State Machine.vi"("error in (no error)"=w255, "State Machine.lvclass"=w256, "Device in"=w260) -> ("error out"=w261:errorcluster, "Device out"=w259:refnum<class "Opt_Selector.lvclass">)  [unwired: 7 in]
          n113 = call "Write WPROT.vi"("error in (no error)"=w261, "Opt_Selector.lvclass"=w259, "Instrument in"=w247) -> ("error out"=w239:errorcluster, "Instrument out"=w240:refnum<class "Instrument.lvclass">)  [unwired: 7 in]
          n114 = Compound Arithmetic op=AND(w283, w272, w251, w250) -> (w285:bool)
          n115 = Select(t=u32 0, s=w285, f=w284) -> (s? t:f=w287:u32)
          n116 = call "Write Instrument.lvclass.vi"("error in (no error)"=w239, "Instrument.lvclass"=w240, "S4ACS_GUI in"=w303) -> ("error out"=w300:errorcluster, "S4ACS_GUI out"=w290:refnum<class "S4GUI.lvclass">)  [unwired: 7 in]
          n117 = Bundle By Name(cluster=w290, "Obs_state"=w287) -> (w289:refnum<class "S4GUI.lvclass">)
        }
        frame 202 {
          # "Dispara o comando para o dispositivo corrente."
          n118 = call "Read Instrument.lvclass.vi"("error in (no error)"=w323, "S4ACS_GUI in"=w324) -> ("error out"=w329:errorcluster, "Instrument.lvclass"=w330:refnum<class "Instrument.lvclass">, "S4ACS_GUI out"=w326:refnum<class "S4GUI.lvclass">)  [unwired: 7 in]
          n119 = call "Read CALW.vi"("error in (no error)"=w329, "Instrument in"=w330) -> ("error out"=w316:errorcluster, "Opt_Selector.lvclass"=w315:refnum<class "Opt_Selector.lvclass">, "Instrument out"=w328:refnum<class "Instrument.lvclass">)  [unwired: 7 in]
          n120 = call-dynamic "Read State Machine.vi"("error in (no error)"=w316, "Device in"=w315) -> ("error out"=w319:errorcluster, "State Machine.lvclass"=w321:refnum<class "State Machine.lvclass">, "Device out"=w313:refnum<class "Opt_Selector.lvclass">)  [unwired: 7 in]
          n121 = call "Next State.vi"("error in (no error)"=w319, "New_State"=1, "State Machine in"=w321) -> ("error out"=w318:errorcluster, "State Machine out"=w317:refnum<class "State Machine.lvclass">)  [unwired: 7 in]
          n122 = call-dynamic "Write State Machine.vi"("error in (no error)"=w318, "State Machine.lvclass"=w317, "Device in"=w313) -> ("error out"=w312:errorcluster, "Device out"=w314:refnum<class "Opt_Selector.lvclass">)  [unwired: 7 in]
          n123 = Increment(x=w310) -> (x+1=w309:u32)
          n124 = call "Write CALW.vi"("error in (no error)"=w312, "Opt_Selector.lvclass"=w314, "Instrument in"=w328) -> ("error out"=w325:errorcluster, "Instrument out"=w327:refnum<class "Instrument.lvclass">)  [unwired: 7 in]
          n125 = call "Write Instrument.lvclass.vi"("error in (no error)"=w325, "Instrument.lvclass"=w327, "S4ACS_GUI in"=w326) -> ("error out"=w322:errorcluster, "S4ACS_GUI out"=w311:refnum<class "S4GUI.lvclass">)  [unwired: 7 in]
          n126 = Bundle By Name(cluster=w311, "Obs_state"=w309) -> (w308:refnum<class "S4GUI.lvclass">)
        }
        frame 203 {
          # "Espera terminar a execução do comando atual \nantes de ir ao proximo passo da Observação."
          n127 = call "Read Instrument.lvclass.vi"("error in (no error)"=w349, "S4ACS_GUI in"=w350) -> ("error out"=w355:errorcluster, "Instrument.lvclass"=w356:refnum<class "Instrument.lvclass">, "S4ACS_GUI out"=w352:refnum<class "S4GUI.lvclass">)  [unwired: 7 in]
          n128 = call "Read CALW.vi"("error in (no error)"=w355, "Instrument in"=w356) -> ("error out"=w343:errorcluster, "Opt_Selector.lvclass"=w342:refnum<class "Opt_Selector.lvclass">, "Instrument out"=w354:refnum<class "Instrument.lvclass">)  [unwired: 7 in]
          n129 = call-dynamic "Read State Machine.vi"("error in (no error)"=w343, "Device in"=w342) -> ("error out"=w346:errorcluster, "State Machine.lvclass"=w347:refnum<class "State Machine.lvclass">, "Device out"=w340:refnum<class "Opt_Selector.lvclass">)  [unwired: 7 in]
          n130 = Increment(x=w333) -> (x+1=w332:u32)
          n131 = call-dynamic "Read State.vi"("error in (no error)"=w346, "State Machine in"=w347) -> ("error out"=w345:errorcluster, "State"=w335:i32, "State Machine out"=w344:refnum<class "State Machine.lvclass">)  [unwired: 7 in]
          n132 = Equal To 0?(x=w335) -> (x = 0?=w336:bool)
          n133 = call-dynamic "Write State Machine.vi"("error in (no error)"=w345, "State Machine.lvclass"=w344, "Device in"=w340) -> ("error out"=w339:errorcluster, "Device out"=w341:refnum<class "Opt_Selector.lvclass">)  [unwired: 7 in]
          n134 = call "Write CALW.vi"("error in (no error)"=w339, "Opt_Selector.lvclass"=w341, "Instrument in"=w354) -> ("error out"=w351:errorcluster, "Instrument out"=w353:refnum<class "Instrument.lvclass">)  [unwired: 7 in]
          n135 = Select(t=w332, s=w336, f=w333) -> (s? t:f=w334:u32)
          n136 = call "Write Instrument.lvclass.vi"("error in (no error)"=w351, "Instrument.lvclass"=w353, "S4ACS_GUI in"=w352) -> ("error out"=w348:errorcluster, "S4ACS_GUI out"=w338:refnum<class "S4GUI.lvclass">)  [unwired: 7 in]
          n137 = Bundle By Name(cluster=w338, "Obs_state"=w334) -> (w337:refnum<class "S4GUI.lvclass">)
        }
        frame 204 {
          # "Dispara o comando para o dispositivo corrente."
          n138 = call "Read Instrument.lvclass.vi"("error in (no error)"=w373, "S4ACS_GUI in"=w374) -> ("error out"=w379:errorcluster, "Instrument.lvclass"=w380:refnum<class "Instrument.lvclass">, "S4ACS_GUI out"=w376:refnum<class "S4GUI.lvclass">)  [unwired: 7 in]
          n139 = call "Read WPSEL.vi"("error in (no error)"=w379, "Instrument in"=w380) -> ("error out"=w366:errorcluster, "Opt_Selector.lvclass"=w365:refnum<class "Opt_Selector.lvclass">, "Instrument out"=w378:refnum<class "Instrument.lvclass">)  [unwired: 7 in]
          n140 = call-dynamic "Read State Machine.vi"("error in (no error)"=w366, "Device in"=w365) -> ("error out"=w369:errorcluster, "State Machine.lvclass"=w371:refnum<class "State Machine.lvclass">, "Device out"=w363:refnum<class "Opt_Selector.lvclass">)  [unwired: 7 in]
          n141 = call "Next State.vi"("error in (no error)"=w369, "New_State"=1, "State Machine in"=w371) -> ("error out"=w368:errorcluster, "State Machine out"=w367:refnum<class "State Machine.lvclass">)  [unwired: 7 in]
          n142 = call-dynamic "Write State Machine.vi"("error in (no error)"=w368, "State Machine.lvclass"=w367, "Device in"=w363) -> ("error out"=w362:errorcluster, "Device out"=w364:refnum<class "Opt_Selector.lvclass">)  [unwired: 7 in]
          n143 = Increment(x=w360) -> (x+1=w359:u32)
          n144 = call "Write WPSEL.vi"("error in (no error)"=w362, "Opt_Selector.lvclass"=w364, "Instrument in"=w378) -> ("error out"=w375:errorcluster, "Instrument out"=w377:refnum<class "Instrument.lvclass">)  [unwired: 7 in]
          n145 = call "Write Instrument.lvclass.vi"("error in (no error)"=w375, "Instrument.lvclass"=w377, "S4ACS_GUI in"=w376) -> ("error out"=w372:errorcluster, "S4ACS_GUI out"=w361:refnum<class "S4GUI.lvclass">)  [unwired: 7 in]
          n146 = Bundle By Name(cluster=w361, "Obs_state"=w359) -> (w358:refnum<class "S4GUI.lvclass">)
        }
        frame 205 {
          # "Espera terminar a execução do comando atual \nantes de ir ao proximo passo da Observação."
          n147 = call "Read Instrument.lvclass.vi"("error in (no error)"=w399, "S4ACS_GUI in"=w400) -> ("error out"=w405:errorcluster, "Instrument.lvclass"=w406:refnum<class "Instrument.lvclass">, "S4ACS_GUI out"=w402:refnum<class "S4GUI.lvclass">)  [unwired: 7 in]
          n148 = call "Read WPSEL.vi"("error in (no error)"=w405, "Instrument in"=w406) -> ("error out"=w393:errorcluster, "Opt_Selector.lvclass"=w392:refnum<class "Opt_Selector.lvclass">, "Instrument out"=w404:refnum<class "Instrument.lvclass">)  [unwired: 7 in]
          n149 = call-dynamic "Read State Machine.vi"("error in (no error)"=w393, "Device in"=w392) -> ("error out"=w396:errorcluster, "State Machine.lvclass"=w397:refnum<class "State Machine.lvclass">, "Device out"=w390:refnum<class "Opt_Selector.lvclass">)  [unwired: 7 in]
          n150 = Increment(x=w383) -> (x+1=w382:u32)
          n151 = call-dynamic "Read State.vi"("error in (no error)"=w396, "State Machine in"=w397) -> ("error out"=w395:errorcluster, "State"=w385:i32, "State Machine out"=w394:refnum<class "State Machine.lvclass">)  [unwired: 7 in]
          n152 = Equal To 0?(x=w385) -> (x = 0?=w386:bool)
          n153 = call-dynamic "Write State Machine.vi"("error in (no error)"=w395, "State Machine.lvclass"=w394, "Device in"=w390) -> ("error out"=w389:errorcluster, "Device out"=w391:refnum<class "Opt_Selector.lvclass">)  [unwired: 7 in]
          n154 = call "Write WPSEL.vi"("error in (no error)"=w389, "Opt_Selector.lvclass"=w391, "Instrument in"=w404) -> ("error out"=w401:errorcluster, "Instrument out"=w403:refnum<class "Instrument.lvclass">)  [unwired: 7 in]
          n155 = Select(t=w382, s=w386, f=w383) -> (s? t:f=w384:u32)
          n156 = call "Write Instrument.lvclass.vi"("error in (no error)"=w401, "Instrument.lvclass"=w403, "S4ACS_GUI in"=w402) -> ("error out"=w398:errorcluster, "S4ACS_GUI out"=w388:refnum<class "S4GUI.lvclass">)  [unwired: 7 in]
          n157 = Bundle By Name(cluster=w388, "Obs_state"=w384) -> (w387:refnum<class "S4GUI.lvclass">)
        }
        frame 206 {
          # "Dispara o comando para o dispositivo corrente."
          n158 = call "Read Instrument.lvclass.vi"("error in (no error)"=w422, "S4ACS_GUI in"=w423) -> ("error out"=w428:errorcluster, "Instrument.lvclass"=w429:refnum<class "Instrument.lvclass">, "S4ACS_GUI out"=w425:refnum<class "S4GUI.lvclass">)  [unwired: 7 in]
          n159 = call "Read WPSEL.vi"("error in (no error)"=w428, "Instrument in"=w429) -> ("error out"=w416:errorcluster, "Opt_Selector.lvclass"=w417:refnum<class "Opt_Selector.lvclass">, "Instrument out"=w427:refnum<class "Instrument.lvclass">)  [unwired: 7 in]
          n160 = call "Read target name.vi"("error in (no error)"=w416, "Optics in"=w417) -> ("error out"=w410:errorcluster, "target name"=w415:string, "Optics out"=w409:refnum<class "Opt_Selector.lvclass">)  [unwired: 7 in]
          n161 = Equal?(x=w415, y="OFF") -> (x = y?=w413:bool)
          n162 = Increment(x=w419) -> (x+1=w411:u32)
          n163 = call "Write WPSEL.vi"("error in (no error)"=w410, "Opt_Selector.lvclass"=w409, "Instrument in"=w427) -> ("error out"=w424:errorcluster, "Instrument out"=w426:refnum<class "Instrument.lvclass">)  [unwired: 7 in]
          n164 = Select(t=u32 0, s=w413, f=w411) -> (s? t:f=w408:u32)
          n165 = call "Write Instrument.lvclass.vi"("error in (no error)"=w424, "Instrument.lvclass"=w426, "S4ACS_GUI in"=w425) -> ("error out"=w421:errorcluster, "S4ACS_GUI out"=w420:refnum<class "S4GUI.lvclass">)  [unwired: 7 in]
          n166 = Bundle By Name(cluster=w420, "Obs_state"=w408) -> (w418:refnum<class "S4GUI.lvclass">)
        }
        frame 207 {
          # "Dispara o comando para o dispositivo corrente."
          n167 = call "Read Instrument.lvclass.vi"("error in (no error)"=w446, "S4ACS_GUI in"=w447) -> ("error out"=w452:errorcluster, "Instrument.lvclass"=w453:refnum<class "Instrument.lvclass">, "S4ACS_GUI out"=w449:refnum<class "S4GUI.lvclass">)  [unwired: 7 in]
          n168 = call "Read WPROT.vi"("error in (no error)"=w452, "Instrument in"=w453) -> ("error out"=w439:errorcluster, "Opt_Selector.lvclass"=w438:refnum<class "Opt_Selector.lvclass">, "Instrument out"=w451:refnum<class "Instrument.lvclass">)  [unwired: 7 in]
          n169 = call-dynamic "Read State Machine.vi"("error in (no error)"=w439, "Device in"=w438) -> ("error out"=w442:errorcluster, "State Machine.lvclass"=w444:refnum<class "State Machine.lvclass">, "Device out"=w436:refnum<class "Opt_Selector.lvclass">)  [unwired: 7 in]
          n170 = call "Next State.vi"("error in (no error)"=w442, "New_State"=1, "State Machine in"=w444) -> ("error out"=w441:errorcluster, "State Machine out"=w440:refnum<class "State Machine.lvclass">)  [unwired: 7 in]
          n171 = call-dynamic "Write State Machine.vi"("error in (no error)"=w441, "State Machine.lvclass"=w440, "Device in"=w436) -> ("error out"=w435:errorcluster, "Device out"=w437:refnum<class "Opt_Selector.lvclass">)  [unwired: 7 in]
          n172 = Increment(x=w433) -> (x+1=w432:u32)
          n173 = call "Write WPROT.vi"("error in (no error)"=w435, "Opt_Selector.lvclass"=w437, "Instrument in"=w451) -> ("error out"=w448:errorcluster, "Instrument out"=w450:refnum<class "Instrument.lvclass">)  [unwired: 7 in]
          n174 = call "Write Instrument.lvclass.vi"("error in (no error)"=w448, "Instrument.lvclass"=w450, "S4ACS_GUI in"=w449) -> ("error out"=w445:errorcluster, "S4ACS_GUI out"=w434:refnum<class "S4GUI.lvclass">)  [unwired: 7 in]
          n175 = Bundle By Name(cluster=w434, "Obs_state"=w432) -> (w431:refnum<class "S4GUI.lvclass">)
        }
        frame 208 {
          # "Espera terminar a execução do comando atual \nantes de ir ao proximo passo da Observação."
          n176 = call "Read Instrument.lvclass.vi"("error in (no error)"=w472, "S4ACS_GUI in"=w473) -> ("error out"=w478:errorcluster, "Instrument.lvclass"=w479:refnum<class "Instrument.lvclass">, "S4ACS_GUI out"=w475:refnum<class "S4GUI.lvclass">)  [unwired: 7 in]
          n177 = call "Read WPROT.vi"("error in (no error)"=w478, "Instrument in"=w479) -> ("error out"=w466:errorcluster, "Opt_Selector.lvclass"=w465:refnum<class "Opt_Selector.lvclass">, "Instrument out"=w477:refnum<class "Instrument.lvclass">)  [unwired: 7 in]
          n178 = call-dynamic "Read State Machine.vi"("error in (no error)"=w466, "Device in"=w465) -> ("error out"=w469:errorcluster, "State Machine.lvclass"=w470:refnum<class "State Machine.lvclass">, "Device out"=w463:refnum<class "Opt_Selector.lvclass">)  [unwired: 7 in]
          n179 = call-dynamic "Read State.vi"("error in (no error)"=w469, "State Machine in"=w470) -> ("error out"=w468:errorcluster, "State"=w458:i32, "State Machine out"=w467:refnum<class "State Machine.lvclass">)  [unwired: 7 in]
          n180 = Equal To 0?(x=w458) -> (x = 0?=w459:bool)
          n181 = call-dynamic "Write State Machine.vi"("error in (no error)"=w468, "State Machine.lvclass"=w467, "Device in"=w463) -> ("error out"=w462:errorcluster, "Device out"=w464:refnum<class "Opt_Selector.lvclass">)  [unwired: 7 in]
          n182 = call "Write WPSEL.vi"("error in (no error)"=w462, "Opt_Selector.lvclass"=w464, "Instrument in"=w477) -> ("error out"=w474:errorcluster, "Instrument out"=w476:refnum<class "Instrument.lvclass">)  [unwired: 7 in]
          n183 = Select(t=u32 0, s=w459, f=w456) -> (s? t:f=w457:u32)
          n184 = call "Write Instrument.lvclass.vi"("error in (no error)"=w474, "Instrument.lvclass"=w476, "S4ACS_GUI in"=w475) -> ("error out"=w471:errorcluster, "S4ACS_GUI out"=w461:refnum<class "S4GUI.lvclass">)  [unwired: 7 in]
          n185 = Bundle By Name(cluster=w461, "Obs_state"=w457) -> (w460:refnum<class "S4GUI.lvclass">)
        }
        frame 251 {
          # "Verifica se ha funcao valida de instrumento:"
          n186 = flat-sequence {
            tunnel: [w526] -> w482
            tunnel: w492 -> [w526]
            frame #0 {
              n187 = Tick Count (ms)() -> (millisecond timer value=→"time3":u32)
            }
          }
          n188 = Unbundle By Name(w484) -> ("Instrument.lvclass"=w488:refnum<class "Instrument.lvclass">)
          n189 = call-dynamic "Load Function.vi"("error in (no error)"=w482, "Instrument in"=w488) -> ("error out"=w485:errorcluster, "Instrument out"=w487:refnum<class "Instrument.lvclass">)  [unwired: 8 in]
          n190 = call-dynamic "Read Function.vi"("error in (no error)"=w485, "Instrument in"=w487) -> ("error out"=w481:errorcluster, "Function"=w480:enum16{"PHOTO", "POLAR", "NONE"}, "Instrument out"=w486:refnum<class "Instrument.lvclass">)  [unwired: 7 in]
          n191 = Bundle By Name(cluster=w484, "Instrument.lvclass"=w486) -> (w483:refnum<class "S4GUI.lvclass">)
          n192 = case shown="\"NONE\"" w480 {
            tunnel: w499 -> [_ w517]
            tunnel: w498 -> [w503 w509]
            tunnel: [u32 1 w508] -> w497
            tunnel: [w503 w507] -> w496
            tunnel: [w501 w506] -> w494
            tunnel: w481 -> [w501 w505]
            tunnel: ["ERROR: No instrument function set (neither POLARIMETRICS nor PHOTOMETRICS )" ("Error Msg") "" ("Error Msg")] -> w491
            frame "NONE" {
            }
            frame Default {
              # "configura o canal,\nmas não dispara\na exposicao."
              # "Dispara o comando para o dispositivo corrente."
              n193 = call-dynamic "Read Channel.vi"("error in (no error)"=w505, "Acquisition in"=w509) -> ("error out"=w514:errorcluster, "Channel.lvclass"=w516:refnum<class "Channel.lvclass">, "Acquisition out"=w524:refnum<class "Acquisition.lvclass">)  [unwired: 7 in]
              n194 = call-dynamic "Write expose.vi"("error in (no error)"=w514, "expose"=FALSE, "Channel in"=w516) -> ("error out"=w513:errorcluster, "Channel out"=w515:refnum<class "Channel.lvclass">)  [unwired: 7 in]
              n195 = call-dynamic "Read State Machine.vi"("error in (no error)"=w513, "Device in"=w515) -> ("error out"=w521:errorcluster, "State Machine.lvclass"=w523:refnum<class "State Machine.lvclass">, "Device out"=w519:refnum<class "Channel.lvclass">)  [unwired: 7 in]
              n196 = call "Next State.vi"("error in (no error)"=w521, "New_State"=1, "State Machine in"=w523) -> ("error out"=w510:errorcluster, "State Machine out"=w511:refnum<class "State Machine.lvclass">)  [unwired: 7 in]
              n197 = call-dynamic "Write State Machine.vi"("error in (no error)"=w510, "State Machine.lvclass"=w511, "Device in"=w519) -> ("error out"=w518:errorcluster, "Device out"=w520:refnum<class "Channel.lvclass">)  [unwired: 7 in]
              n198 = call-dynamic "Write Channel.vi"("error in (no error)"=w518, "Channel.lvclass"=w520, "Acquisition in"=w524) -> ("error out"=w506:errorcluster, "Acquisition out"=w507:refnum<class "Acquisition.lvclass">)  [unwired: 7 in]
              n199 = Increment(x=w517) -> (x+1=w508:u32)
            }
          }
          n200 = Bundle By Name(cluster=w483, "Error Msg"=w491, "cyclesDone"=u32 0) -> (w490:refnum<class "S4GUI.lvclass">)
          n201 = call-dynamic "Write Acq_state.vi"("error in (no error)"=w494, "Acq_state"=w497, "Acquisition in"=w496) -> ("error out"=w493:errorcluster, "Acquisition out"=w495:refnum<class "Acquisition.lvclass">)  [unwired: 7 in]
        }
        frame 252 {
          # "Erro no Texp."
          # "Erro no setup\ninicial do ACS."
          # "Espera terminar a execução do comando atual \nantes de ir ao proximo passo da Observação."
          n202 = flat-sequence {
            tunnel: [w571] -> w539
            tunnel: w540 -> [w571]
            frame #0 {
              n203 = Tick Count (ms)() -> (millisecond timer value=→"time4":u32)
            }
          }
          n204 = call-dynamic "Read Channel.vi"("error in (no error)"=w539, "Acquisition in"=w545) -> ("error out"=w554:errorcluster, "Channel.lvclass"=w553:refnum<class "Channel.lvclass">, "Acquisition out"=w555:refnum<class "Acquisition.lvclass">)  [unwired: 7 in]
          n205 = call-dynamic "Read State Machine.vi"("error in (no error)"=w554, "Device in"=w553) -> ("error out"=w547:errorcluster, "State Machine.lvclass"=w549:refnum<class "State Machine.lvclass">, "Device out"=w551:refnum<class "Channel.lvclass">)  [unwired: 7 in]
          n206 = call-dynamic "Read State.vi"("error in (no error)"=w547, "State Machine in"=w549) -> ("error out"=w546:errorcluster, "State"=w537:i32, "State Machine out"=w548:refnum<class "State Machine.lvclass">)  [unwired: 7 in]
          n207 = Equal To 0?(x=w537) -> (x = 0?=w535:bool)
          n208 = call-dynamic "Write State Machine.vi"("error in (no error)"=w546, "State Machine.lvclass"=w548, "Device in"=w551) -> ("error out"=w550:errorcluster, "Device out"=w552:refnum<class "Channel.lvclass">)  [unwired: 7 in]
          n209 = Equal?(x=28, y=w537) -> (x = y?=w534:bool)
          n210 = Equal?(x=38, y=w537) -> (x = y?=w533:bool)
          n211 = call-dynamic "Write Channel.vi"("error in (no error)"=w550, "Channel.lvclass"=w552, "Acquisition in"=w555) -> ("error out"=w544:errorcluster, "Acquisition out"=w543:refnum<class "Acquisition.lvclass">)  [unwired: 7 in]
          n212 = Build Array(w535, w534, w533) -> (w532:bool[])
          n213 = Boolean Array To Number(Boolean array=w532) -> (number=w531:u32)
          n214 = case shown="0, Default" w531 {
            tunnel: w530 -> [w557 _ _ _]
            tunnel: [w557 u32 300 ("t") u32 1 ("t") u32 1 ("t")] -> w529
            tunnel: w528 -> [w556 w560 w565 w569]
            tunnel: [w556 w559 w564 w568] -> w527
            frame 0, Default {
            }
            frame 1 {
              n215 = Tick Count (ms)() -> (millisecond timer value=→"time307":u32)
              n216 = Bundle By Name(cluster=w560, "Error Msg"="") -> (w559:refnum<class "S4GUI.lvclass">)
            }
            frame 2 {
              n217 = Bundle By Name(cluster=w565, "Error Msg"="ERROR: Some channel initialization failed. S4GUI:HandleObservationAsync.vi state 252.") -> (w564:refnum<class "S4GUI.lvclass">)
            }
            frame 4 {
              n218 = Bundle By Name(cluster=w569, "Error Msg"="ERROR: Some channel with invalid Exposition Time. S4GUI:HandleObservationAsync.vi state 252.") -> (w568:refnum<class "S4GUI.lvclass">)
            }
          }
          n219 = call-dynamic "Write Acq_state.vi"("error in (no error)"=w544, "Acq_state"=w529, "Acquisition in"=w543) -> ("error out"=w541:errorcluster, "Acquisition out"=w542:refnum<class "Acquisition.lvclass">)  [unwired: 7 in]
        }
        frame 253 {
          # "Sem syncbox, \ntrigger mode = 0 (internal)"
          n220 = call-dynamic "Read Channel.vi"("error in (no error)"=w574, "Acquisition in"=w606) -> ("error out"=w579:errorcluster, "Channel.lvclass"=w578:refnum<class "Channel.lvclass">, "Acquisition out"=w601:refnum<class "Acquisition.lvclass">)  [unwired: 7 in]
          n221 = call-dynamic "Read Interface.vi"("error in (no error)"=w579, "Channel in"=w578) -> ("error out"=w577:errorcluster, "Interface.lvclass"=w583:refnum<class "Interface.lvclass">, "Channel out"=w582:refnum<class "Channel.lvclass">)  [unwired: 7 in]
          n222 = call-dynamic "Get CCD_Config.vi"("error in (no error)"=w577, "Interface in"=w583) -> ("error out"=w590:errorcluster, "output cluster"=w592:T1, "Interface out"=w589:refnum<class "Interface.lvclass">)  [unwired: 7 in]
          n223 = Bundle By Name(cluster=w592, "TRIGGER_MODE"=u8 0) -> (w588:T1)
          n224 = call-dynamic "Set CCD_Config.vi"("error in (no error)"=w590, "input cluster"=w588, "Interface in"=w589) -> ("error out"=w586:errorcluster, "Interface out"=w584:refnum<class "Interface.lvclass">)  [unwired: 7 in]
          n225 = Flatten To String(anything=w588, error in (no error)=w586) -> (data string=w587:string, error out=w585:errorcluster)  [unwired: 2 in, 1 out]
          n226 = call "Write flatted cluster.vi"("error in (no error)"=w585, "flatted cluster"=w587, "Interface in"=w584) -> ("error out"=w580:errorcluster, "Interface out"=w581:refnum<class "Interface.lvclass">)  [unwired: 7 in]
          n227 = call-dynamic "Write Interface.vi"("error in (no error)"=w580, "Interface.lvclass"=w581, "Channel in"=w582) -> ("error out"=w576:errorcluster, "Channel out"=w575:refnum<class "Channel.lvclass">)  [unwired: 7 in]
          n228 = call-dynamic "Read State Machine.vi"("error in (no error)"=w576, "Device in"=w575) -> ("error out"=w598:errorcluster, "State Machine.lvclass"=w600:refnum<class "State Machine.lvclass">, "Device out"=w596:refnum<class "Channel.lvclass">)  [unwired: 7 in]
          n229 = Increment(x=w603) -> (x+1=w604:u32)
          n230 = call "Next State.vi"("error in (no error)"=w598, "New_State"=60, "State Machine in"=w600) -> ("error out"=w593:errorcluster, "State Machine out"=w594:refnum<class "State Machine.lvclass">)  [unwired: 7 in]
          n231 = call-dynamic "Write State Machine.vi"("error in (no error)"=w593, "State Machine.lvclass"=w594, "Device in"=w596) -> ("error out"=w595:errorcluster, "Device out"=w597:refnum<class "Channel.lvclass">)  [unwired: 7 in]
          n232 = call-dynamic "Write Channel.vi"("error in (no error)"=w595, "Channel.lvclass"=w597, "Acquisition in"=w601) -> ("error out"=w602:errorcluster, "Acquisition out"=w605:refnum<class "Acquisition.lvclass">)  [unwired: 7 in]
          n233 = call-dynamic "Write Acq_state.vi"("error in (no error)"=w602, "Acq_state"=w604, "Acquisition in"=w605) -> ("error out"=w607:errorcluster, "Acquisition out"=w608:refnum<class "Acquisition.lvclass">)  [unwired: 7 in]
        }
        frame 254 {
          # "Espera terminar a execução do comando atual \nantes de ir ao proximo passo da Observação."
          n234 = call-dynamic "Read Channel.vi"("error in (no error)"=w611, "Acquisition in"=w618) -> ("error out"=w629:errorcluster, "Channel.lvclass"=w628:refnum<class "Channel.lvclass">, "Acquisition out"=w630:refnum<class "Acquisition.lvclass">)  [unwired: 7 in]
          n235 = call-dynamic "Read State Machine.vi"("error in (no error)"=w629, "Device in"=w628) -> ("error out"=w622:errorcluster, "State Machine.lvclass"=w624:refnum<class "State Machine.lvclass">, "Device out"=w626:refnum<class "Channel.lvclass">)  [unwired: 7 in]
          n236 = call-dynamic "Read State.vi"("error in (no error)"=w622, "State Machine in"=w624) -> ("error out"=w621:errorcluster, "State"=w619:i32, "State Machine out"=w623:refnum<class "State Machine.lvclass">)  [unwired: 7 in]
          n237 = Equal To 0?(x=w619) -> (x = 0?=w620:bool)
          n238 = call-dynamic "Write State Machine.vi"("error in (no error)"=w621, "State Machine.lvclass"=w623, "Device in"=w626) -> ("error out"=w625:errorcluster, "Device out"=w627:refnum<class "Channel.lvclass">)  [unwired: 7 in]
          n239 = call-dynamic "Write Channel.vi"("error in (no error)"=w625, "Channel.lvclass"=w627, "Acquisition in"=w630) -> ("error out"=w615:errorcluster, "Acquisition out"=w614:refnum<class "Acquisition.lvclass">)  [unwired: 7 in]
          n240 = Select(t=u32 299, s=w620, f=w610) -> (s? t:f=w616:u32)
          n241 = call-dynamic "Write Acq_state.vi"("error in (no error)"=w615, "Acq_state"=w616, "Acquisition in"=w614) -> ("error out"=w612:errorcluster, "Acquisition out"=w613:refnum<class "Acquisition.lvclass">)  [unwired: 7 in]
        }
        frame 271 {
          # "configura o canal,\nmas não dispara\na exposicao."
          # "Dispara o comando para o dispositivo corrente."
          n242 = flat-sequence {
            tunnel: [w662] -> w639
            tunnel: w640 -> [w662]
            frame #0 {
              n243 = Tick Count (ms)() -> (millisecond timer value=→"time5":u32)
            }
          }
          n244 = call-dynamic "Read Channel.vi"("error in (no error)"=w639, "Acquisition in"=w645) -> ("error out"=w650:errorcluster, "Channel.lvclass"=w652:refnum<class "Channel.lvclass">, "Acquisition out"=w660:refnum<class "Acquisition.lvclass">)  [unwired: 7 in]
          n245 = call-dynamic "Write expose.vi"("error in (no error)"=w650, "expose"=FALSE, "Channel in"=w652) -> ("error out"=w649:errorcluster, "Channel out"=w651:refnum<class "Channel.lvclass">)  [unwired: 7 in]
          n246 = call-dynamic "Read State Machine.vi"("error in (no error)"=w649, "Device in"=w651) -> ("error out"=w657:errorcluster, "State Machine.lvclass"=w659:refnum<class "State Machine.lvclass">, "Device out"=w655:refnum<class "Channel.lvclass">)  [unwired: 7 in]
          n247 = call "Next State.vi"("error in (no error)"=w657, "New_State"=1, "State Machine in"=w659) -> ("error out"=w646:errorcluster, "State Machine out"=w647:refnum<class "State Machine.lvclass">)  [unwired: 7 in]
          n248 = call-dynamic "Write State Machine.vi"("error in (no error)"=w646, "State Machine.lvclass"=w647, "Device in"=w655) -> ("error out"=w654:errorcluster, "Device out"=w656:refnum<class "Channel.lvclass">)  [unwired: 7 in]
          n249 = call-dynamic "Write Channel.vi"("error in (no error)"=w654, "Channel.lvclass"=w656, "Acquisition in"=w660) -> ("error out"=w632:errorcluster, "Acquisition out"=w643:refnum<class "Acquisition.lvclass">)  [unwired: 7 in]
          n250 = Increment(x=w653) -> (x+1=w644:u32)
          n251 = Unbundle By Name(w634) -> ("TelFocus.lvclass"=w636:refnum<class "TelFocus.lvclass">)
          n252 = call-dynamic "Write focus #stepsdone.vi"("error in (no error)"=w632, "focus #stepsdone"=u32 0, "TelFocus in"=w636) -> ("error out"=w631:errorcluster, "TelFocus out"=w633:refnum<class "TelFocus.lvclass">)  [unwired: 7 in]
          n253 = Bundle By Name(cluster=w634, "TelFocus.lvclass"=w633, "Error Msg"="") -> (w637:refnum<class "S4GUI.lvclass">)
          n254 = call-dynamic "Write Acq_state.vi"("error in (no error)"=w631, "Acq_state"=w644, "Acquisition in"=w643) -> ("error out"=w641:errorcluster, "Acquisition out"=w642:refnum<class "Acquisition.lvclass">)  [unwired: 7 in]
        }
        frame 272 {
          # "Erro no Texp."
          # "Erro no setup\ninicial do ACS."
          # "Espera terminar a execução do comando atual \nantes de ir ao proximo passo da Observação."
          n255 = flat-sequence {
            tunnel: [w706] -> w675
            tunnel: w676 -> [w706]
            frame #0 {
              n256 = Tick Count (ms)() -> (millisecond timer value=→"time6":u32)
            }
          }
          n257 = call-dynamic "Read Channel.vi"("error in (no error)"=w675, "Acquisition in"=w681) -> ("error out"=w690:errorcluster, "Channel.lvclass"=w689:refnum<class "Channel.lvclass">, "Acquisition out"=w691:refnum<class "Acquisition.lvclass">)  [unwired: 7 in]
          n258 = call-dynamic "Read State Machine.vi"("error in (no error)"=w690, "Device in"=w689) -> ("error out"=w683:errorcluster, "State Machine.lvclass"=w685:refnum<class "State Machine.lvclass">, "Device out"=w687:refnum<class "Channel.lvclass">)  [unwired: 7 in]
          n259 = call-dynamic "Read State.vi"("error in (no error)"=w683, "State Machine in"=w685) -> ("error out"=w682:errorcluster, "State"=w673:i32, "State Machine out"=w684:refnum<class "State Machine.lvclass">)  [unwired: 7 in]
          n260 = Equal To 0?(x=w673) -> (x = 0?=w671:bool)
          n261 = call-dynamic "Write State Machine.vi"("error in (no error)"=w682, "State Machine.lvclass"=w684, "Device in"=w687) -> ("error out"=w686:errorcluster, "Device out"=w688:refnum<class "Channel.lvclass">)  [unwired: 7 in]
          n262 = Equal?(x=28, y=w673) -> (x = y?=w670:bool)
          n263 = Equal?(x=38, y=w673) -> (x = y?=w669:bool)
          n264 = call-dynamic "Write Channel.vi"("error in (no error)"=w686, "Channel.lvclass"=w688, "Acquisition in"=w691) -> ("error out"=w680:errorcluster, "Acquisition out"=w679:refnum<class "Acquisition.lvclass">)  [unwired: 7 in]
          n265 = Build Array(w671, w670, w669) -> (w668:bool[])
          n266 = Boolean Array To Number(Boolean array=w668) -> (number=w667:u32)
          n267 = case shown="0, Default" w667 {
            tunnel: w666 -> [w692 _ _ _]
            tunnel: [w692 u32 360 ("t") u32 0 ("t") u32 0 ("t")] -> w665
            tunnel: w664 -> [w693 w695 w700 w704]
            tunnel: [w693 w694 w699 w703] -> w663
            frame 0, Default {
            }
            frame 1 {
              n268 = Bundle By Name(cluster=w695, "Error Msg"="") -> (w694:refnum<class "S4GUI.lvclass">)
            }
            frame 2 {
              n269 = Bundle By Name(cluster=w700, "Error Msg"="ERROR: Some channel initialization failed. S4GUI:HandleObservationAsync.vi state 272.") -> (w699:refnum<class "S4GUI.lvclass">)
            }
            frame 4 {
              n270 = Bundle By Name(cluster=w704, "Error Msg"="ERROR: Some channel with invalid Exposition Time. S4GUI:HandleObservationAsync.vi state 272.") -> (w703:refnum<class "S4GUI.lvclass">)
            }
          }
          n271 = call-dynamic "Write Acq_state.vi"("error in (no error)"=w680, "Acq_state"=w665, "Acquisition in"=w679) -> ("error out"=w677:errorcluster, "Acquisition out"=w678:refnum<class "Acquisition.lvclass">)  [unwired: 7 in]
        }
        frame 300 {
          # "Verifica se é modo fotometria ou polarimetria:\nTrue = polarimetria (estado 301)\nFalse = fotometria (estado 321)"
          n272 = flat-sequence {
            tunnel: [w734] -> w723
            tunnel: w724 -> [w734]
            frame #0 {
              n273 = local read "time4"() -> (w736:u32)
              n274 = local read "time3"() -> (w735:u32)
              n275 = Subtract(x=w736, y=w735) -> (x-y=→"delay 3-4":u32)
            }
          }
          n276 = call "Read Instrument.lvclass.vi"("error in (no error)"=w723, "S4ACS_GUI in"=w733) -> ("error out"=w730:errorcluster, "Instrument.lvclass"=w731:refnum<class "Instrument.lvclass">, "S4ACS_GUI out"=w720:refnum<class "S4GUI.lvclass">)  [unwired: 7 in]
          n277 = call-dynamic "Read mode.vi"("error in (no error)"=w730, "Instrument in"=w731) -> ("error out"=w710:errorcluster, "mode"=w729:bool)  [unwired: 7 in, 1 out]
          n278 = call-dynamic "Read Channel.vi"("error in (no error)"=w710, "Acquisition in"=w718) -> ("error out"=w712:errorcluster, "Channel.lvclass"=w714:refnum<class "Channel.lvclass">, "Acquisition out"=w717:refnum<class "Acquisition.lvclass">)  [unwired: 7 in]
          n279 = call-dynamic "Write PrevCyclesDone.vi"("error in (no error)"=w712, "PrevCyclesDone"=u32 0, "Channel in"=w714) -> ("error out"=w711:errorcluster, "Channel out"=w713:refnum<class "Channel.lvclass">)  [unwired: 7 in]
          n280 = call-dynamic "Write Channel.vi"("error in (no error)"=w711, "Channel.lvclass"=w713, "Acquisition in"=w717) -> ("error out"=w709:errorcluster, "Acquisition out"=w716:refnum<class "Acquisition.lvclass">)  [unwired: 7 in]
          n281 = Select(t=u32 301, s=w729, f=u32 321 ("t")) -> (s? t:f=w727:u32)
          n282 = call-dynamic "Write Acq_state.vi"("error in (no error)"=w709, "Acq_state"=w727, "Acquisition in"=w716) -> ("error out"=w726:errorcluster, "Acquisition out"=w725:refnum<class "Acquisition.lvclass">)  [unwired: 7 in]
          n283 = Bundle By Name(cluster=w720, "cyclesDone"=u32 0, "sequesDone"=u32 0, "seqAtual"=u32 0) -> (w719:refnum<class "S4GUI.lvclass">)
        }
        frame 301 {
          # "Se for polarimetria com 1 pos,\ndesabilita WAIT EXPOSE no ACS."
          # "Envia WAIT_EXPOSE_COMMAND ...\nON (se forem varias posicoes) ou\nOFF (se for uma única posição da lâmina.)"
          n284 = call-dynamic "VerifWavePlate.vi"("error in (no error)"=w742, "S4GUI in"=w743) -> ("error out"=w741:errorcluster, "One Position"=w739:bool, "S4GUI out"=w740:refnum<class "S4GUI.lvclass">)  [unwired: 7 in]
          n285 = Not(x=w739) -> (.not. x?=w738:bool)
          n286 = call-dynamic "Read Channel.vi"("error in (no error)"=w741, "Acquisition in"=w757) -> ("error out"=w745:errorcluster, "Channel.lvclass"=w747:refnum<class "Channel.lvclass">, "Acquisition out"=w765:refnum<class "Acquisition.lvclass">)  [unwired: 7 in]
          n287 = call-dynamic "Write wait_expose.vi"("error in (no error)"=w745, "wait_expose"=w738, "Channel in"=w747) -> ("error out"=w744:errorcluster, "Channel out"=w746:refnum<class "Channel.lvclass">)  [unwired: 7 in]
          n288 = call-dynamic "Read State Machine.vi"("error in (no error)"=w744, "Device in"=w746) -> ("error out"=w762:errorcluster, "State Machine.lvclass"=w764:refnum<class "State Machine.lvclass">, "Device out"=w760:refnum<class "Channel.lvclass">)  [unwired: 7 in]
          n289 = call "Next State.vi"("error in (no error)"=w762, "New_State"=40, "State Machine in"=w764) -> ("error out"=w750:errorcluster, "State Machine out"=w751:refnum<class "State Machine.lvclass">)  [unwired: 7 in]
          n290 = call-dynamic "Write State Machine.vi"("error in (no error)"=w750, "State Machine.lvclass"=w751, "Device in"=w760) -> ("error out"=w759:errorcluster, "Device out"=w761:refnum<class "Channel.lvclass">)  [unwired: 7 in]
          n291 = Increment(x=w758) -> (x+1=w756:u32)
          n292 = call-dynamic "Write Channel.vi"("error in (no error)"=w759, "Channel.lvclass"=w761, "Acquisition in"=w765) -> ("error out"=w755:errorcluster, "Acquisition out"=w754:refnum<class "Acquisition.lvclass">)  [unwired: 7 in]
          n293 = call-dynamic "Write Acq_state.vi"("error in (no error)"=w755, "Acq_state"=w756, "Acquisition in"=w754) -> ("error out"=w752:errorcluster, "Acquisition out"=w753:refnum<class "Acquisition.lvclass">)  [unwired: 7 in]
          n294 = Bundle By Name(cluster=w740, "Error Msg"="") -> (w748:refnum<class "S4GUI.lvclass">)
        }
        frame 302 {
          # "Espera canal voltar para IDLE"
          n295 = call-dynamic "Read Channel.vi"("error in (no error)"=w781, "Acquisition in"=w782) -> ("error out"=w772:errorcluster, "Channel.lvclass"=w773:refnum<class "Channel.lvclass">, "Acquisition out"=w774:refnum<class "Acquisition.lvclass">)  [unwired: 7 in]
          n296 = call-dynamic "Read State Machine.vi"("error in (no error)"=w772, "Device in"=w773) -> ("error out"=w775:errorcluster, "State Machine.lvclass"=w777:refnum<class "State Machine.lvclass">)  [unwired: 7 in, 1 out]
          n297 = call-dynamic "Read State.vi"("error in (no error)"=w775, "State Machine in"=w777) -> ("error out"=w770:errorcluster, "State"=w776:i32)  [unwired: 7 in, 1 out]
          n298 = Equal?(x=0, y=w776) -> (x = y?=w766:bool)
          n299 = Increment(x=w768) -> (x+1=w769:u32)
          n300 = Select(t=w769, s=w766, f=w768) -> (s? t:f=w771:u32)
          n301 = call-dynamic "Write Acq_state.vi"("error in (no error)"=w770, "Acq_state"=w771, "Acquisition in"=w774) -> ("error out"=w779:errorcluster, "Acquisition out"=w780:refnum<class "Acquisition.lvclass">)  [unwired: 7 in]
        }
        frame 303 {
          # "2024 04 26: ATEN敲O: NO MODO POLARIMETRIA ASYNC, APENAS 1 CANAL POR VEZ PODE FAZER AQUISI敲O!\nO atributo S4GUI:SeqAtual pode se perder se mais de um canal rodar aqui..."
          n302 = flat-sequence {
            tunnel: w788 -> [w829]
            tunnel: [w829] -> w787
            frame #0 {
              n303 = Tick Count (ms)() -> (millisecond timer value=→"time1":u32)
            }
          }
          n304 = call "Read Instrument.lvclass.vi"("error in (no error)"=w787, "S4ACS_GUI in"=w825) -> ("error out"=w827:errorcluster, "Instrument.lvclass"=w828:refnum<class "Instrument.lvclass">, "S4ACS_GUI out"=w785:refnum<class "S4GUI.lvclass">)  [unwired: 7 in]
          n305 = call "Read WPROT.vi"("error in (no error)"=w827, "Instrument in"=w828) -> ("error out"=w822:errorcluster, "Opt_Selector.lvclass"=w823:refnum<class "Opt_Selector.lvclass">, "Instrument out"=w826:refnum<class "Instrument.lvclass">)  [unwired: 7 in]
          n306 = call-dynamic "getTargetPos.vi"("error in (no error)"=w822, "Opt_Selector in"=w823) -> ("error out"=w821:errorcluster, "Target Pos"=w801:u16, "Opt_Selector out"=w820:refnum<class "Opt_Selector.lvclass">)  [unwired: 7 in]
          n307 = Build Array(-1.0 ("element"), 0.0 ("element"), 22.5 ("element"), 45.0 ("element"), 67.5 ("element"), 90.0 ("element"), 112.5 ("element"), 135.0 ("element"), 157.5 ("element"), 180.0 ("element"), 202.5 ("element"), 225.0 ("element"), 247.5 ("element"), 270.0 ("element"), 292.5 ("element"), 315.0 ("element"), 337.5 ("element")) -> (w813:dbl[])
          n308 = Unbundle By Name(w785) -> ("seqAtual"=w786:u32)
          n309 = Index Array(array=w813, index=w801) -> (element=w800:dbl)
          n310 = case shown="0, Default" w801 {
            selector: w801 -> [_ w863]
            tunnel: w826 -> [w839 w851]
            tunnel: [w839 w851] -> w796
            tunnel: [w836 w850] -> w795
            tunnel: w824 -> [_ w865]
            tunnel: [u32 314 w864] -> w794
            tunnel: w821 -> [w837 w859]
            tunnel: w820 -> [w838 w858]
            tunnel: w800 -> [_ w853]
            tunnel: [w834 w852] -> w797
            tunnel: [u32 0 ("seqAtual") w841] -> w784
            tunnel: w786 -> [_ w842]
            frame 0, Default {
              # "Verifica os ciclos"
              # "Recupera a sequencia anterior para o caso \nde repetição da sequencia (sem precisar clicar \nnas posicoes desejadas novamente)."
              n311 = call-dynamic "Read sequencia_ant.vi"("error in (no error)"=w837, "Opt_Selector in"=w838) -> ("error out"=w833:errorcluster, "sequencia_ant"=w832:u16, "Opt_Selector out"=w835:refnum<class "Opt_Selector.lvclass">)  [unwired: 7 in]
              n312 = call-dynamic "Write sequencia.vi"("error in (no error)"=w833, "sequencia"=w832, "Opt_Selector in"=w835) -> ("error out"=w836:errorcluster, "Opt_Selector out"=w834:refnum<class "Opt_Selector.lvclass">)  [unwired: 7 in]
            }
            frame 1..16 {
              # "Inicia o Ticks com\nvalor do relogio atual"
              # "Espera até 40 x 0.25s (= 10s) para\nmecanismo entrar em READY"
              n313 = Number To Decimal String(number=w863) -> (decimal integer string=w862:string)  [unwired: 1 in]
              n314 = Concatenate Strings("WP" ("string"), w862) -> (w860:string)
              n315 = call "Write target name.vi"("error in (no error)"=w859, "target name"=w860, "Optics in"=w858) -> ("error out"=w856:errorcluster, "Optics out"=w857:refnum<class "Opt_Selector.lvclass">)  [unwired: 7 in]
              n316 = call "Write target.vi"("error in (no error)"=w856, "target"=w853, "Optics in"=w857) -> ("error out"=w855:errorcluster, "Optics out"=w854:refnum<class "Opt_Selector.lvclass">)  [unwired: 7 in]
              n317 = call-dynamic "Read State Machine.vi"("error in (no error)"=w855, "Device in"=w854) -> ("error out"=w867:errorcluster, "State Machine.lvclass"=w869:refnum<class "State Machine.lvclass">, "Device out"=w866:refnum<class "Opt_Selector.lvclass">)  [unwired: 7 in]
              n318 = Increment(x=w865) -> (x+1=w864:u32)
              n319 = Increment(x=w842) -> (x+1=w841:u32)
              n320 = call "Next State.vi"("error in (no error)"=w867, "New_State"=1, "State Machine in"=w869) -> ("error out"=w848:errorcluster, "State Machine out"=w849:refnum<class "State Machine.lvclass">)  [unwired: 7 in]
              n321 = call-dynamic "Write Timer.vi"("error in (no error)"=w848, "Timer"=u32 40, "State Machine in"=w849) -> ("error out"=w845:errorcluster, "State Machine out"=w846:refnum<class "State Machine.lvclass">)  [unwired: 7 in]
              n322 = call-dynamic "Init Ticks.vi"("error in (no error)"=w845, "State Machine in"=w846) -> ("error out"=w843:errorcluster, "State Machine out"=w844:refnum<class "State Machine.lvclass">)  [unwired: 8 in]
              n323 = call-dynamic "Write State Machine.vi"("error in (no error)"=w843, "State Machine.lvclass"=w844, "Device in"=w866) -> ("error out"=w850:errorcluster, "Device out"=w852:refnum<class "Opt_Selector.lvclass">)  [unwired: 7 in]
            }
          }
          n324 = call "Write WPROT.vi"("error in (no error)"=w795, "Opt_Selector.lvclass"=w797, "Instrument in"=w796) -> ("error out"=w799:errorcluster, "Instrument out"=w798:refnum<class "Instrument.lvclass">)  [unwired: 7 in]
          n325 = Bundle By Name(cluster=w785, "seqAtual"=w784) -> (w783:refnum<class "S4GUI.lvclass">)
          n326 = call "Write Instrument.lvclass.vi"("error in (no error)"=w799, "Instrument.lvclass"=w798, "S4ACS_GUI in"=w783) -> ("error out"=w792:errorcluster, "S4ACS_GUI out"=w791:refnum<class "S4GUI.lvclass">)  [unwired: 7 in]
          n327 = call-dynamic "Write Acq_state.vi"("error in (no error)"=w792, "Acq_state"=w794, "Acquisition in"=w793) -> ("error out"=w790:errorcluster, "Acquisition out"=w789:refnum<class "Acquisition.lvclass">)  [unwired: 7 in]
        }
        frame 304 {
          # "Para inserir Pausa antes do\nEXPOSE, ir para 305."
          # "Espera terminar o movimento para a posição \"target\" do waveplate\nantes de ir para o estado que dispara a aquisição de imagens.\n\n20230424: Não precisa mais atualizar o valor de WPPOS com o\ncomando WRITE_HEADER porque o ACS já recebeu a sequência de\nposições da lâmina"
          n328 = flat-sequence {
            tunnel: [w929] -> w896
            tunnel: w897 -> [w929]
            frame #0 {
              n329 = Tick Count (ms)() -> (millisecond timer value=→"time 2":u32)
            }
          }
          n330 = call "Read Instrument.lvclass.vi"("error in (no error)"=w896, "S4ACS_GUI in"=w909) -> ("error out"=w914:errorcluster, "Instrument.lvclass"=w915:refnum<class "Instrument.lvclass">, "S4ACS_GUI out"=w911:refnum<class "S4GUI.lvclass">)  [unwired: 7 in]
          n331 = call "Read WPROT.vi"("error in (no error)"=w914, "Instrument in"=w915) -> ("error out"=w879:errorcluster, "Opt_Selector.lvclass"=w908:refnum<class "Opt_Selector.lvclass">, "Instrument out"=w913:refnum<class "Instrument.lvclass">)  [unwired: 7 in]
          n332 = call-dynamic "Read Channel.vi"("error in (no error)"=w879, "Acquisition in"=w881) -> ("error out"=w875:errorcluster, "Channel.lvclass"=w876:refnum<class "Channel.lvclass">, "Acquisition out"=w880:refnum<class "Acquisition.lvclass">)  [unwired: 7 in]
          n333 = call-dynamic "Read wait_expose.vi"("error in (no error)"=w875, "Channel in"=w876) -> ("error out"=w878:errorcluster, "wait_expose"=w877:bool)  [unwired: 7 in, 1 out]
          n334 = call-dynamic "Read State Machine.vi"("error in (no error)"=w878, "Device in"=w908) -> ("error out"=w885:errorcluster, "State Machine.lvclass"=w888:refnum<class "State Machine.lvclass">, "Device out"=w906:refnum<class "Opt_Selector.lvclass">)  [unwired: 7 in]
          n335 = call-dynamic "Verif Clock.vi"("error in (no error)"=w885, "period (ms)"=u32 20000 ("period"), "State Machine in"=w888) -> ("error out"=w889:errorcluster, "State Machine out"=w887:refnum<class "State Machine.lvclass">)  [unwired: 6 in, 1 out]
          n336 = call-dynamic "Read Timeout.vi"("error in (no error)"=w889, "State Machine in"=w887) -> ("error out"=w884:errorcluster, "Timeout"=w883:bool, "State Machine out"=w886:refnum<class "State Machine.lvclass">)  [unwired: 7 in]
          n337 = call-dynamic "Read State.vi"("error in (no error)"=w884, "State Machine in"=w886) -> ("error out"=w898:errorcluster, "State"=w904:i32, "State Machine out"=w899:refnum<class "State Machine.lvclass">)  [unwired: 7 in]
          n338 = call-dynamic "Write State Machine.vi"("error in (no error)"=w898, "State Machine.lvclass"=w899, "Device in"=w906) -> ("error out"=w905:errorcluster, "Device out"=w907:refnum<class "Opt_Selector.lvclass">)  [unwired: 7 in]
          n339 = Equal To 0?(x=w904) -> (x = 0?=w872:bool)
          n340 = call "Write WPROT.vi"("error in (no error)"=w905, "Opt_Selector.lvclass"=w907, "Instrument in"=w913) -> ("error out"=w910:errorcluster, "Instrument out"=w912:refnum<class "Instrument.lvclass">)  [unwired: 7 in]
          n341 = call "Write Instrument.lvclass.vi"("error in (no error)"=w910, "Instrument.lvclass"=w912, "S4ACS_GUI in"=w911) -> ("error out"=w902:errorcluster, "S4ACS_GUI out"=w891:refnum<class "S4GUI.lvclass">)  [unwired: 7 in]
          n342 = case shown="False" w883 {
            tunnel: w873 -> [w918 _]
            tunnel: [w918 u32 1 ("Obs_state")] -> w892
            tunnel: w891 -> [w917 w923]
            tunnel: [w917 w922] -> w882
            tunnel: [w916 FALSE] -> w871
            tunnel: w872 -> [w916 _]
            frame False {
            }
            frame True {
              n343 = Bundle By Name(cluster=w923, "Error Msg"="ERROR: moving waveplate (S4GUI:HandleObservationAsync.vi - state 304)") -> (w922:refnum<class "S4GUI.lvclass">)
            }
          }
          n344 = Unbundle By Name(w891) -> ("cyclesDone"=w894:u32, "sequesDone"=w893:u32)
          n345 = Add(x=w894, y=w893) -> (x+y=w895:u32)
          n346 = Equal To 0?(x=w895) -> ()  [unwired: 1 out]
          n347 = case shown="True" TRUE {
            tunnel: [w924 u32 308 ("t")] -> w870
            tunnel: w877 -> [w926 _]
            frame False {
              # "2a seq. em diante: depende\nde Channel.wait_expose"
              n348 = Select(t=u32 308, s=w926, f=u32 326 ("t")) -> (s? t:f=w924:u32)
            }
            frame True {
              # "1a. seq.: Envia EXPOSE"
            }
          }
          n349 = Increment(x=w873) -> ()  [unwired: 1 out]
          n350 = Select(t=w870, s=w871, f=w892) -> (s? t:f=w903:u32)
          n351 = call-dynamic "Write Acq_state.vi"("error in (no error)"=w902, "Acq_state"=w903, "Acquisition in"=w880) -> ("error out"=w901:errorcluster, "Acquisition out"=w900:refnum<class "Acquisition.lvclass">)  [unwired: 7 in]
        }
        frame 305 {
          # "Pausa de 200ms entre posicio-\nnamento da lamina e o envio de\nEXPOSE."
          n352 = Tick Count (ms)() -> (millisecond timer value=w938:u32)
          n353 = local read "time 2"() -> (w940:u32)
          n354 = Subtract(x=w938, y=w940) -> (x-y=w942:u32)
          n355 = To Double Precision Float(number=w942) -> (double precision float=w943:dbl)
          n356 = Less?(x=200.0 ("y"), y=w943) -> (x < y?=w939:bool)
          n357 = case shown="True" w939 {
            tunnel: [w944 u32 308 ("t")] -> w934
            tunnel: w938 -> [_ w945]
            tunnel: w935 -> [w944 _]
            frame False {
            }
            frame True {
              # "1a sequencia:\nenvia EXPOSE"
              n358 = local write "time 2"(w945) -> ()
            }
          }
          n359 = call-dynamic "Write Acq_state.vi"("error in (no error)"=w936, "Acq_state"=w934, "Acquisition in"=w937) -> ("error out"=w933:errorcluster, "Acquisition out"=w932:refnum<class "Acquisition.lvclass">)  [unwired: 7 in]
        }
        frame 308 {
          # "Dispara o comando para o dispositivo corrente."
          n360 = call-dynamic "Read Channel.vi"("error in (no error)"=w957, "Acquisition in"=w958) -> ("error out"=w964:errorcluster, "Channel.lvclass"=w963:refnum<class "Channel.lvclass">, "Acquisition out"=w968:refnum<class "Acquisition.lvclass">)  [unwired: 7 in]
          n361 = call-dynamic "Read State Machine.vi"("error in (no error)"=w964, "Device in"=w963) -> ("error out"=w965:errorcluster, "State Machine.lvclass"=w967:refnum<class "State Machine.lvclass">, "Device out"=w961:refnum<class "Channel.lvclass">)  [unwired: 7 in]
          n362 = call "Next State.vi"("error in (no error)"=w965, "New_State"=50, "State Machine in"=w967) -> ("error out"=w950:errorcluster, "State Machine out"=w951:refnum<class "State Machine.lvclass">)  [unwired: 7 in]
          n363 = call-dynamic "Write State Machine.vi"("error in (no error)"=w950, "State Machine.lvclass"=w951, "Device in"=w961) -> ("error out"=w960:errorcluster, "Device out"=w962:refnum<class "Channel.lvclass">)  [unwired: 7 in]
          n364 = Increment(x=w959) -> (x+1=w956:u32)
          n365 = call-dynamic "Write Channel.vi"("error in (no error)"=w960, "Channel.lvclass"=w962, "Acquisition in"=w968) -> ("error out"=w955:errorcluster, "Acquisition out"=w954:refnum<class "Acquisition.lvclass">)  [unwired: 7 in]
          n366 = call-dynamic "Write Acq_state.vi"("error in (no error)"=w955, "Acq_state"=w956, "Acquisition in"=w954) -> ("error out"=w952:errorcluster, "Acquisition out"=w953:refnum<class "Acquisition.lvclass">)  [unwired: 7 in]
          n367 = Bundle By Name(cluster=w949, "Error Msg"="") -> (w947:refnum<class "S4GUI.lvclass">)
        }
        frame 309 {
          # "OV 20241016 -Cancelada a verificacao do \nSeqsDone incrementar, pois agora o ACS garante as\ntransicoes Detector Status:  IDLE->ACTIVE->WAITING..."
          # "Se wait_expose=T, não envia\no EXPOSE do estado 308\n(1o EXPOSE já foi enviado).\n\nNeste caso, vai para:\n* 312 se houver mais \n   de 1 posição da lamina ou para \n* 326 se houver apenas 1 posição\n   da lâmina"
          # "OV 20240821 -Espera ACTIVE ou SeqsDone incrementar."
          n368 = Unbundle By Name(w990) -> ("seqAtual"=w989:u32)
          n369 = flat-sequence {
            tunnel: [w1031] -> w973
            tunnel: w985 -> [w1031]
            frame #0 {
              n370 = Tick Count (ms)() -> (millisecond timer value=→"time308":u32)
            }
          }
          n371 = call "Read id.vi"("error in (no error)"=w973, "Server in"=w971) -> ("error out"=w972:errorcluster, "id"=w969:u32, "Server out"=w970:refnum<class "Acquisition.lvclass">)  [unwired: 7 in]
          n372 = call-dynamic "Read Channel.vi"("error in (no error)"=w972, "Acquisition in"=w970) -> ("error out"=w977:errorcluster, "Channel.lvclass"=w979:refnum<class "Channel.lvclass">, "Acquisition out"=w1014:refnum<class "Acquisition.lvclass">)  [unwired: 7 in]
          n373 = call-dynamic "Read Status.vi"("error in (no error)"=w977, "Channel in"=w979) -> ("error out"=w976:errorcluster, "Status"=w975:T2, "Channel out"=w978:refnum<class "Channel.lvclass">)  [unwired: 7 in]
          n374 = Unbundle By Name(w975) -> ("Error"=w974:bool)
          n375 = call-dynamic "Read SequesDone.vi"("error in (no error)"=w976, "Channel in"=w978) -> ("error out"=w991:errorcluster, "SequesDoneRaw"=w992:u32, "Channel out"=w993:refnum<class "Channel.lvclass">)  [unwired: 6 in, 1 out]
          n376 = call-dynamic "Read wait_expose.vi"("error in (no error)"=w991, "Channel in"=w993) -> ("error out"=w999:errorcluster, "Channel out"=w1000:refnum<class "Channel.lvclass">)  [unwired: 7 in, 1 out]
          n377 = Equal?(x=w992, y=w989) -> (x = y?=w986:bool)
          n378 = call-dynamic "Read State Machine.vi"("error in (no error)"=w999, "Device in"=w1000) -> ("error out"=w1008:errorcluster, "State Machine.lvclass"=w1010:refnum<class "State Machine.lvclass">, "Device out"=w1012:refnum<class "Channel.lvclass">)  [unwired: 7 in]
          n379 = call-dynamic "Read State.vi"("error in (no error)"=w1008, "State Machine in"=w1010) -> ("error out"=w1007:errorcluster, "State"=w1002:i32, "State Machine out"=w1009:refnum<class "State Machine.lvclass">)  [unwired: 7 in]
          n380 = call-dynamic "Write State Machine.vi"("error in (no error)"=w1007, "State Machine.lvclass"=w1009, "Device in"=w1012) -> ("error out"=w1011:errorcluster, "Device out"=w1013:refnum<class "Channel.lvclass">)  [unwired: 7 in]
          n381 = Greater?(x=w1002, y=53) -> (0:w988:bool)
          n382 = disable-structure shown="Enabled" {
            disable-tunnel: w988 -> [w1029 w1030]
            disable-tunnel: [w1028 w1030] -> w987
            disable-tunnel: w986 -> [w1027 _]
            frame Disabled {
              n383 = Or(x=w1029, y=w1027) -> (x .or. y?=w1028:bool)
            }
            frame Enabled {
            }
          }
          n384 = call-dynamic "Write Channel.vi"("error in (no error)"=w1011, "Channel.lvclass"=w1013, "Acquisition in"=w1014) -> ("error out"=w998:errorcluster, "Acquisition out"=w1006:refnum<class "Acquisition.lvclass">)  [unwired: 7 in]
          n385 = call-dynamic "VerifWavePlate.vi"("error in (no error)"=w998, "S4GUI in"=w990) -> ("error out"=w997:errorcluster, "One Position"=w996:bool, "S4GUI out"=w981:refnum<class "S4GUI.lvclass">)  [unwired: 7 in]
          n386 = Select(t=u32 328, s=w996, f=u32 312 ("t")) -> (s? t:f=w984:u32)
          n387 = Select(t=w984, s=w987, f=w1001) -> (s? t:f=w983:u32)
          n388 = case shown="False" w974 {
            tunnel: [w1017 u32 1 ("Acq_state")] -> w982
            tunnel: w983 -> [w1017 _]
            tunnel: w981 -> [w1016 w1021]
            tunnel: [w1016 w1020] -> w980
            tunnel: w969 -> [_ w1019]
            frame False {
              n389 = Tick Count (ms)() -> (millisecond timer value=w1015:u32)
              n390 = local write "time307"(w1015) -> ()
            }
            frame True {
              n391 = Increment(x=w1019) -> (x+1=w1018:u32)
              n392 = Number To Decimal String(number=w1018) -> (decimal integer string=w1024:string)  [unwired: 1 in]
              n393 = Concatenate Strings("CHANNEL ", w1024, ": Error flag TRUE - see ACS panel.  HandleObservationAsync.vi - state 309.") -> (w1026:string)
              n394 = Bundle By Name(cluster=w1021, "Error Msg"=w1026) -> (w1020:refnum<class "S4GUI.lvclass">)
            }
          }
          n395 = call-dynamic "Write Acq_state.vi"("error in (no error)"=w997, "Acq_state"=w982, "Acquisition in"=w1006) -> ("error out"=w1004:errorcluster, "Acquisition out"=w1005:refnum<class "Acquisition.lvclass">)  [unwired: 7 in]
        }
        frame 312 {
          # "Exemplo:\nSET #CYCLES 3\nSET #SEQ 4\ntotal de sequencias: 3 x 4 = 12\n\nseq.        CYCLES_DONE           SEQS_DONE\n1a.                     0                                 0\n2a.                     0                                 1 \n3a.                     0                                 2 \n4a.                     0                                 3 \n\n5a.                     1                                 4->0 \n6a.                     1                                 1 \n7a.                     1                                 2 \n8a.                     1                                 3 \n\n9a.                     2                                 4->0 \n10a.                   2                                 1 \n11a.                   2                                 2 \n12a.                   2                                 3 \n\nfim                    3                                 4"
          # "SEQS_DONE = 0,1,2,...,n,0,1,..."
          n396 = Unbundle By Name(w1050) -> ("seqAtual"=w1051:u32)
          n397 = call-dynamic "Read Channel.vi"("error in (no error)"=w1056, "Acquisition in"=w1057) -> ("error out"=w1043:errorcluster, "Channel.lvclass"=w1045:refnum<class "Channel.lvclass">, "Acquisition out"=w1058:refnum<class "Acquisition.lvclass">)  [unwired: 7 in]
          n398 = call-dynamic "Read stopping.vi"("error in (no error)"=w1043, "Channel in"=w1045) -> ("error out"=w1042:errorcluster, "stopping"=w1041:bool, "Channel out"=w1044:refnum<class "Channel.lvclass">)  [unwired: 7 in]
          n399 = call-dynamic "Read SequesDone.vi"("error in (no error)"=w1042, "Channel in"=w1044) -> ("error out"=w1052:errorcluster, "SequesDoneRaw"=w1033:u32, "Channel out"=w1053:refnum<class "Channel.lvclass">)  [unwired: 6 in, 1 out]
          n400 = Equal?(x=w1033, y=w1051) -> (x = y?=w1046:bool)
          n401 = call-dynamic "Write Channel.vi"("error in (no error)"=w1052, "Channel.lvclass"=w1053, "Acquisition in"=w1058) -> ("error out"=w1039:errorcluster, "Acquisition out"=w1040:refnum<class "Acquisition.lvclass">)  [unwired: 7 in]
          n402 = call-dynamic "GetCubeDuration.vi"("error in (no error)"=w1039, "Acquisition in"=w1040) -> ("error out"=w1038:errorcluster, "Acquisition out"=w1037:refnum<class "Acquisition.lvclass">, "CubeDuration"=w1036:dbl)  [unwired: 7 in]
          n403 = Multiply(x=w1036, y=1000.0) -> (x*y=w1035:dbl)
          n404 = case shown="False" w1046 {
            tunnel: w1050 -> [w1060 w1077]
            tunnel: [w1059 w1077] -> w1049
            tunnel: [w1061 w1079] -> w1048
            tunnel: w1047 -> [w1062 _]
            tunnel: w1041 -> [_ w1078]
            tunnel: w1035 -> [w1068 _]
            frame False {
              n405 = Add(x=1000.0, y=w1068) -> (x+y=w1066:dbl)
              n406 = local read "time307"() -> (w1069:u32)
              n407 = Tick Count (ms)() -> (millisecond timer value=w1070:u32)
              n408 = Subtract(x=w1070, y=w1069) -> (x-y=w1065:u32)
              n409 = To Double Precision Float(number=w1065) -> (double precision float=w1064:dbl)
              n410 = Less?(x=w1066, y=w1064) -> (x < y?=w1063:bool)
              n411 = case shown="True" w1063 {
                tunnel: w1062 -> [w1072 _]
                tunnel: [w1072 u32 1 ("Acq_state")] -> w1061
                tunnel: [w1071 w1074] -> w1059
                tunnel: w1060 -> [w1071 w1075]
                frame False {
                }
                frame True {
                  n412 = Bundle By Name(cluster=w1075, "Error Msg"="ERROR: Acquisition Timeout - HandleObservationAsync.vi - state 312.") -> (w1074:refnum<class "S4GUI.lvclass">)
                }
              }
            }
            frame True {
              n413 = case shown="False" w1078 {
                tunnel: [u32 303 ("Obs_state") u32 0 ("Obs_state")] -> w1079
                frame False {
                }
                frame True {
                }
              }
            }
          }
          n414 = call-dynamic "Write Acq_state.vi"("error in (no error)"=w1038, "Acq_state"=w1048, "Acquisition in"=w1037) -> ("error out"=w1054:errorcluster, "Acquisition out"=w1055:refnum<class "Acquisition.lvclass">)  [unwired: 7 in]
        }
        frame 314 {
          n415 = disable-structure shown="Enabled" {
            disable-tunnel: w1087 -> [w1104 w1120]
            disable-tunnel: w1086 -> [w1103 w1121]
            disable-tunnel: [w1092 w1119] -> w1085
            disable-tunnel: [w1091 w1118] -> w1084
            disable-tunnel: w1083 -> [w1088 w1115]
            disable-tunnel: [w1088 w1114] -> w1082
            frame Disabled {
              n416 = call-dynamic "Read Channel.vi"("error in (no error)"=w1104, "Acquisition in"=w1103) -> ("error out"=w1102:errorcluster, "Channel.lvclass"=w1101:refnum<class "Channel.lvclass">, "Acquisition out"=w1089:refnum<class "Acquisition.lvclass">)  [unwired: 7 in]
              n417 = call-dynamic "Read ciclos.vi"("error in (no error)"=w1102, "Channel in"=w1101) -> ("error out"=w1098:errorcluster, "ciclos"=w1100:u32, "Channel out"=w1090:refnum<class "Channel.lvclass">)  [unwired: 7 in]
              n418 = Decrement(x=w1100) -> (x-1=w1105:u32)
              n419 = Greater Than 0?(x=w1105) -> (x > 0?=w1109:bool)
              n420 = case shown="True" w1109 {
                selector: w1109 -> [w1111 w1113]
                tunnel: w1105 -> [_ w1112]
                tunnel: [w1111 w1113] -> w1108
                tunnel: [u32 0 w1112] -> w1095
                frame False {
                }
                frame True {
                }
              }
              n421 = call-dynamic "Write ciclos.vi"("error in (no error)"=w1098, "ciclos"=w1095, "Channel in"=w1090) -> ("error out"=w1097:errorcluster, "Channel out"=w1096:refnum<class "Channel.lvclass">)  [unwired: 7 in]
              n422 = Select(t=u32 301, s=w1108, f=u32 0) -> (s? t:f=w1099:u32)
              n423 = call-dynamic "Write Channel.vi"("error in (no error)"=w1097, "Channel.lvclass"=w1096, "Acquisition in"=w1089) -> ("error out"=w1093:errorcluster, "Acquisition out"=w1094:refnum<class "Acquisition.lvclass">)  [unwired: 7 in]
              n424 = call-dynamic "Write Acq_state.vi"("error in (no error)"=w1093, "Acq_state"=w1099, "Acquisition in"=w1094) -> ("error out"=w1091:errorcluster, "Acquisition out"=w1092:refnum<class "Acquisition.lvclass">)  [unwired: 7 in]
            }
            frame Enabled {
              n425 = Unbundle By Name(w1115) -> ("cyclesDone"=w1117:u32)
              n426 = Increment(x=w1117) -> (x+1=w1116:u32)
              n427 = Bundle By Name(cluster=w1115, "cyclesDone"=w1116) -> (w1114:refnum<class "S4GUI.lvclass">)
              n428 = Unbundle By Name(w1114) -> ("TotalCiclos"=w1128:u32, "cyclesDone"=w1127:u32)
              n429 = Subtract(x=w1128, y=w1127) -> (x-y=w1126:u32)
              n430 = Greater Than 0?(x=w1126) -> (x > 0?=w1125:bool)
              n431 = Select(t=u32 303, s=w1125, f=u32 0) -> (s? t:f=w1122:u32)
              n432 = call-dynamic "Write Acq_state.vi"("error in (no error)"=w1120, "Acq_state"=w1122, "Acquisition in"=w1121) -> ("error out"=w1118:errorcluster, "Acquisition out"=w1119:refnum<class "Acquisition.lvclass">)  [unwired: 7 in]
            }
          }
        }
        frame 321 {
          # "Envia: WAIT_EXPOSE_COMMAND  OFF"
          # "Para Fotometria Async -> DESABILITA comando EXPOSE para os ACS."
          n433 = call-dynamic "Read Channel.vi"("error in (no error)"=w1144, "Acquisition in"=w1145) -> ("error out"=w1131:errorcluster, "Channel.lvclass"=w1133:refnum<class "Channel.lvclass">, "Acquisition out"=w1153:refnum<class "Acquisition.lvclass">)  [unwired: 7 in]
          n434 = call-dynamic "Write wait_expose.vi"("error in (no error)"=w1131, "wait_expose"=FALSE, "Channel in"=w1133) -> ("error out"=w1130:errorcluster, "Channel out"=w1132:refnum<class "Channel.lvclass">)  [unwired: 7 in]
          n435 = call-dynamic "Read State Machine.vi"("error in (no error)"=w1130, "Device in"=w1132) -> ("error out"=w1150:errorcluster, "State Machine.lvclass"=w1152:refnum<class "State Machine.lvclass">, "Device out"=w1148:refnum<class "Channel.lvclass">)  [unwired: 7 in]
          n436 = call "Next State.vi"("error in (no error)"=w1150, "New_State"=40, "State Machine in"=w1152) -> ("error out"=w1137:errorcluster, "State Machine out"=w1138:refnum<class "State Machine.lvclass">)  [unwired: 7 in]
          n437 = call-dynamic "Write State Machine.vi"("error in (no error)"=w1137, "State Machine.lvclass"=w1138, "Device in"=w1148) -> ("error out"=w1147:errorcluster, "Device out"=w1149:refnum<class "Channel.lvclass">)  [unwired: 7 in]
          n438 = Increment(x=w1146) -> (x+1=w1143:u32)
          n439 = call-dynamic "Write Channel.vi"("error in (no error)"=w1147, "Channel.lvclass"=w1149, "Acquisition in"=w1153) -> ("error out"=w1142:errorcluster, "Acquisition out"=w1141:refnum<class "Acquisition.lvclass">)  [unwired: 7 in]
          n440 = call-dynamic "Write Acq_state.vi"("error in (no error)"=w1142, "Acq_state"=w1143, "Acquisition in"=w1141) -> ("error out"=w1139:errorcluster, "Acquisition out"=w1140:refnum<class "Acquisition.lvclass">)  [unwired: 7 in]
          n441 = Bundle By Name(cluster=w1136, "Error Msg"="") -> (w1134:refnum<class "S4GUI.lvclass">)
        }
        frame 322 {
          # "Espera canal voltar para IDLE"
          n442 = call-dynamic "Read Channel.vi"("error in (no error)"=w1169, "Acquisition in"=w1170) -> ("error out"=w1160:errorcluster, "Channel.lvclass"=w1161:refnum<class "Channel.lvclass">, "Acquisition out"=w1162:refnum<class "Acquisition.lvclass">)  [unwired: 7 in]
          n443 = call-dynamic "Read State Machine.vi"("error in (no error)"=w1160, "Device in"=w1161) -> ("error out"=w1163:errorcluster, "State Machine.lvclass"=w1165:refnum<class "State Machine.lvclass">)  [unwired: 7 in, 1 out]
          n444 = call-dynamic "Read State.vi"("error in (no error)"=w1163, "State Machine in"=w1165) -> ("error out"=w1158:errorcluster, "State"=w1164:i32)  [unwired: 7 in, 1 out]
          n445 = Equal?(x=0, y=w1164) -> (x = y?=w1154:bool)
          n446 = Increment(x=w1156) -> (x+1=w1157:u32)
          n447 = Select(t=w1157, s=w1154, f=w1156) -> (s? t:f=w1159:u32)
          n448 = call-dynamic "Write Acq_state.vi"("error in (no error)"=w1158, "Acq_state"=w1159, "Acquisition in"=w1162) -> ("error out"=w1167:errorcluster, "Acquisition out"=w1168:refnum<class "Acquisition.lvclass">)  [unwired: 7 in]
        }
        frame 323 {
          # "Envia: EXPOSE para o ACS"
          # "Dispara o comando para o dispositivo corrente."
          n449 = flat-sequence {
            tunnel: w1172 -> [w1194]
            tunnel: [w1194] -> w1171
            frame #0 {
              n450 = Tick Count (ms)() -> (millisecond timer value=w1195:u32)
              n451 = local write "time 2"(w1195) -> ()
            }
          }
          n452 = call-dynamic "Read Channel.vi"("error in (no error)"=w1171, "Acquisition in"=w1183) -> ("error out"=w1189:errorcluster, "Channel.lvclass"=w1188:refnum<class "Channel.lvclass">, "Acquisition out"=w1193:refnum<class "Acquisition.lvclass">)  [unwired: 7 in]
          n453 = call-dynamic "Read State Machine.vi"("error in (no error)"=w1189, "Device in"=w1188) -> ("error out"=w1190:errorcluster, "State Machine.lvclass"=w1192:refnum<class "State Machine.lvclass">, "Device out"=w1186:refnum<class "Channel.lvclass">)  [unwired: 7 in]
          n454 = call "Next State.vi"("error in (no error)"=w1190, "New_State"=50, "State Machine in"=w1192) -> ("error out"=w1176:errorcluster, "State Machine out"=w1177:refnum<class "State Machine.lvclass">)  [unwired: 7 in]
          n455 = call-dynamic "Write State Machine.vi"("error in (no error)"=w1176, "State Machine.lvclass"=w1177, "Device in"=w1186) -> ("error out"=w1185:errorcluster, "Device out"=w1187:refnum<class "Channel.lvclass">)  [unwired: 7 in]
          n456 = Increment(x=w1184) -> (x+1=w1180:u32)
          n457 = call-dynamic "Write Channel.vi"("error in (no error)"=w1185, "Channel.lvclass"=w1187, "Acquisition in"=w1193) -> ("error out"=w1179:errorcluster, "Acquisition out"=w1181:refnum<class "Acquisition.lvclass">)  [unwired: 7 in]
          n458 = call-dynamic "Write Acq_state.vi"("error in (no error)"=w1179, "Acq_state"=w1180, "Acquisition in"=w1181) -> ("error out"=w1178:errorcluster, "Acquisition out"=w1182:refnum<class "Acquisition.lvclass">)  [unwired: 7 in]
          n459 = Bundle By Name(cluster=w1175, "Error Msg"="") -> (w1174:refnum<class "S4GUI.lvclass">)
        }
        frame 324 {
          # "Espera Status Detector entrar em ACTIVE"
          n460 = call "Read id.vi"("error in (no error)"=w1198, "Server in"=w1200) -> ("error out"=w1197:errorcluster, "id"=w1196:u32, "Server out"=w1199:refnum<class "Acquisition.lvclass">)  [unwired: 7 in]
          n461 = call-dynamic "Read Channel.vi"("error in (no error)"=w1197, "Acquisition in"=w1199) -> ("error out"=w1209:errorcluster, "Channel.lvclass"=w1210:refnum<class "Channel.lvclass">, "Acquisition out"=w1232:refnum<class "Acquisition.lvclass">)  [unwired: 7 in]
          n462 = call-dynamic "Read Status.vi"("error in (no error)"=w1209, "Channel in"=w1210) -> ("error out"=w1207:errorcluster, "Status"=w1208:T2, "Channel out"=w1206:refnum<class "Channel.lvclass">)  [unwired: 7 in]
          n463 = Unbundle By Name(w1208) -> ("Error"=w1203:bool)
          n464 = call-dynamic "Read wait_expose.vi"("error in (no error)"=w1207, "Channel in"=w1206) -> ("error out"=w1216:errorcluster, "wait_expose"=w1214:bool, "Channel out"=w1217:refnum<class "Channel.lvclass">)  [unwired: 7 in]
          n465 = call-dynamic "Read State Machine.vi"("error in (no error)"=w1216, "Device in"=w1217) -> ("error out"=w1226:errorcluster, "State Machine.lvclass"=w1228:refnum<class "State Machine.lvclass">, "Device out"=w1230:refnum<class "Channel.lvclass">)  [unwired: 7 in]
          n466 = call-dynamic "Read State.vi"("error in (no error)"=w1226, "State Machine in"=w1228) -> ("error out"=w1225:errorcluster, "State"=w1219:i32, "State Machine out"=w1227:refnum<class "State Machine.lvclass">)  [unwired: 7 in]
          n467 = Greater?(x=w1219, y=53) -> (0:w1211:bool)
          n468 = call-dynamic "Write State Machine.vi"("error in (no error)"=w1225, "State Machine.lvclass"=w1227, "Device in"=w1230) -> ("error out"=w1229:errorcluster, "Device out"=w1231:refnum<class "Channel.lvclass">)  [unwired: 7 in]
          n469 = call-dynamic "Write Channel.vi"("error in (no error)"=w1229, "Channel.lvclass"=w1231, "Acquisition in"=w1232) -> ("error out"=w1220:errorcluster, "Acquisition out"=w1221:refnum<class "Acquisition.lvclass">)  [unwired: 7 in]
          n470 = Increment(x=w1224) -> (x+1=w1213:u32)
          n471 = Select(t=327 ("y"), s=w1214, f=w1213) -> (s? t:f=w1212:u32)
          n472 = Select(t=w1212, s=w1211, f=w1224) -> (s? t:f=w1204:u32)
          n473 = case shown="True" w1203 {
            tunnel: [w1235 u32 1 ("Acq_state")] -> w1205
            tunnel: w1204 -> [w1235 _]
            tunnel: w1202 -> [w1234 w1239]
            tunnel: [w1234 w1238] -> w1201
            tunnel: w1196 -> [_ w1237]
            frame False {
              n474 = Tick Count (ms)() -> (millisecond timer value=w1233:u32)
              n475 = local write "time307"(w1233) -> ()
            }
            frame True {
              n476 = Increment(x=w1237) -> (x+1=w1236:u32)
              n477 = Number To Decimal String(number=w1236) -> (decimal integer string=w1242:string)  [unwired: 1 in]
              n478 = Concatenate Strings("CHANNEL ", w1242, ": Error flag TRUE - see ACS panel.  HandleObservationAsync.vi - state 324.") -> (w1244:string)
              n479 = Bundle By Name(cluster=w1239, "Error Msg"=w1244) -> (w1238:refnum<class "S4GUI.lvclass">)
            }
          }
          n480 = call-dynamic "Write Acq_state.vi"("error in (no error)"=w1220, "Acq_state"=w1205, "Acquisition in"=w1221) -> ("error out"=w1222:errorcluster, "Acquisition out"=w1223:refnum<class "Acquisition.lvclass">)  [unwired: 7 in]
        }
        frame 325 {
          # "Dispara o comando para o dispositivo corrente."
          n481 = call-dynamic "Read Channel.vi"("error in (no error)"=w1245, "Acquisition in"=w1250) -> ("error out"=w1251:errorcluster, "Channel.lvclass"=w1246:refnum<class "Channel.lvclass">, "Acquisition out"=w1248:refnum<class "Acquisition.lvclass">)  [unwired: 7 in]
          n482 = call-dynamic "Read wait_expose.vi"("error in (no error)"=w1251, "Channel in"=w1246) -> ("error out"=w1247:errorcluster, "wait_expose"=w1249:bool)  [unwired: 7 in, 1 out]
          n483 = case shown="False" w1249 {
            tunnel: w1248 -> [w1262 w1268]
            tunnel: w1247 -> [w1261 w1267]
            tunnel: [w1262 w1266] -> w1258
            tunnel: [w1261 w1265] -> w1256
            frame False {
            }
            frame True {
              n484 = call-dynamic "Read Channel.vi"("error in (no error)"=w1267, "Acquisition in"=w1268) -> ("error out"=w1273:errorcluster, "Channel.lvclass"=w1272:refnum<class "Channel.lvclass">, "Acquisition out"=w1277:refnum<class "Acquisition.lvclass">)  [unwired: 7 in]
              n485 = call-dynamic "Read State Machine.vi"("error in (no error)"=w1273, "Device in"=w1272) -> ("error out"=w1274:errorcluster, "State Machine.lvclass"=w1276:refnum<class "State Machine.lvclass">, "Device out"=w1270:refnum<class "Channel.lvclass">)  [unwired: 7 in]
              n486 = call "Next State.vi"("error in (no error)"=w1274, "New_State"=50, "State Machine in"=w1276) -> ("error out"=w1263:errorcluster, "State Machine out"=w1264:refnum<class "State Machine.lvclass">)  [unwired: 7 in]
              n487 = call-dynamic "Write State Machine.vi"("error in (no error)"=w1263, "State Machine.lvclass"=w1264, "Device in"=w1270) -> ("error out"=w1269:errorcluster, "Device out"=w1271:refnum<class "Channel.lvclass">)  [unwired: 7 in]
              n488 = call-dynamic "Write Channel.vi"("error in (no error)"=w1269, "Channel.lvclass"=w1271, "Acquisition in"=w1277) -> ("error out"=w1265:errorcluster, "Acquisition out"=w1266:refnum<class "Acquisition.lvclass">)  [unwired: 7 in]
            }
          }
          n489 = Increment(x=w1260) -> (x+1=w1257:u32)
          n490 = call-dynamic "Write Acq_state.vi"("error in (no error)"=w1256, "Acq_state"=w1257, "Acquisition in"=w1258) -> ("error out"=w1255:errorcluster, "Acquisition out"=w1259:refnum<class "Acquisition.lvclass">)  [unwired: 7 in]
          n491 = Bundle By Name(cluster=w1252, "Error Msg"="") -> (w1254:refnum<class "S4GUI.lvclass">)
        }
        frame 326 {
          # "Espera Status Detector entrar em ACTIVE"
          n492 = call "Read id.vi"("error in (no error)"=w1280, "Server in"=w1283) -> ("error out"=w1281:errorcluster, "id"=w1279:u32, "Server out"=w1282:refnum<class "Acquisition.lvclass">)  [unwired: 7 in]
          n493 = call-dynamic "Read Channel.vi"("error in (no error)"=w1281, "Acquisition in"=w1282) -> ("error out"=w1285:errorcluster, "Channel.lvclass"=w1288:refnum<class "Channel.lvclass">, "Acquisition out"=w1310:refnum<class "Acquisition.lvclass">)  [unwired: 7 in]
          n494 = call-dynamic "Read Status.vi"("error in (no error)"=w1285, "Channel in"=w1288) -> ("error out"=w1284:errorcluster, "Status"=w1286:T2, "Channel out"=w1287:refnum<class "Channel.lvclass">)  [unwired: 7 in]
          n495 = Unbundle By Name(w1286) -> ("Error"=w1278:bool)
          n496 = call-dynamic "Read State Machine.vi"("error in (no error)"=w1284, "Device in"=w1287) -> ("error out"=w1304:errorcluster, "State Machine.lvclass"=w1306:refnum<class "State Machine.lvclass">, "Device out"=w1308:refnum<class "Channel.lvclass">)  [unwired: 7 in]
          n497 = call-dynamic "Read State.vi"("error in (no error)"=w1304, "State Machine in"=w1306) -> ("error out"=w1303:errorcluster, "State"=w1297:i32, "State Machine out"=w1305:refnum<class "State Machine.lvclass">)  [unwired: 7 in]
          n498 = disable-structure shown="Enabled" {
            disable-tunnel: w1295 -> [w1312 w1313]
            disable-tunnel: [w1311 w1313] -> w1294
            frame Disabled {
              n499 = Increment(x=w1312) -> (x+1=w1311:u32)
            }
            frame Enabled {
              # "OV20241108:\nNão espera mais \nCyclesDone>0 em 327"
            }
          }
          n500 = Greater?(x=w1297, y=53) -> (0:w1302:bool)
          n501 = call-dynamic "Write State Machine.vi"("error in (no error)"=w1303, "State Machine.lvclass"=w1305, "Device in"=w1308) -> ("error out"=w1307:errorcluster, "Device out"=w1309:refnum<class "Channel.lvclass">)  [unwired: 7 in]
          n502 = call-dynamic "Write Channel.vi"("error in (no error)"=w1307, "Channel.lvclass"=w1309, "Acquisition in"=w1310) -> ("error out"=w1298:errorcluster, "Acquisition out"=w1299:refnum<class "Acquisition.lvclass">)  [unwired: 7 in]
          n503 = Select(t=u32 328, s=w1302, f=w1294) -> (s? t:f=w1292:u32)
          n504 = case shown="False" w1278 {
            tunnel: [w1316 u32 1 ("Acq_state")] -> w1291
            tunnel: w1292 -> [w1316 _]
            tunnel: w1290 -> [w1315 w1320]
            tunnel: [w1315 w1319] -> w1289
            tunnel: w1279 -> [_ w1318]
            frame False {
              n505 = Tick Count (ms)() -> (millisecond timer value=w1314:u32)
              n506 = local write "time307"(w1314) -> ()
            }
            frame True {
              n507 = Increment(x=w1318) -> (x+1=w1317:u32)
              n508 = Number To Decimal String(number=w1317) -> (decimal integer string=w1323:string)  [unwired: 1 in]
              n509 = Concatenate Strings("CHANNEL ", w1323, ": Error flag TRUE - see ACS panel.  HandleObservationAsync.vi - state 326.") -> (w1325:string)
              n510 = Bundle By Name(cluster=w1320, "Error Msg"=w1325) -> (w1319:refnum<class "S4GUI.lvclass">)
            }
          }
          n511 = call-dynamic "Write Acq_state.vi"("error in (no error)"=w1298, "Acq_state"=w1291, "Acquisition in"=w1299) -> ("error out"=w1300:errorcluster, "Acquisition out"=w1301:refnum<class "Acquisition.lvclass">)  [unwired: 7 in]
        }
        frame 327 {
          # "Verifica se CyclesDone lido do STATUS igualou ao PrevCycles+1"
          n512 = call "Read id.vi"("error in (no error)"=w1331, "Server in"=w1332) -> ("error out"=w1329:errorcluster, "id"=w1328:u32, "Server out"=w1330:refnum<class "Acquisition.lvclass">)  [unwired: 7 in]
          n513 = call-dynamic "Read Channel.vi"("error in (no error)"=w1329, "Acquisition in"=w1330) -> ("error out"=w1341:errorcluster, "Channel.lvclass"=w1342:refnum<class "Channel.lvclass">, "Acquisition out"=w1352:refnum<class "Acquisition.lvclass">)  [unwired: 7 in]
          n514 = Increment(x=w1328) -> (x+1=w1327:u32)
          n515 = call-dynamic "Read PrevCyclesDone.vi"("error in (no error)"=w1341, "Channel in"=w1342) -> ("error out"=w1344:errorcluster, "PrevCyclesDone"=w1343:u32, "Channel out"=w1345:refnum<class "Channel.lvclass">)  [unwired: 7 in]
          n516 = call-dynamic "Read CyclesDone.vi"("error in (no error)"=w1344, "Channel in"=w1345) -> ("error out"=w1338:errorcluster, "CyclesDone"=w1333:u32, "Channel out"=w1340:refnum<class "Channel.lvclass">)  [unwired: 7 in]
          n517 = Increment(x=w1343) -> (x+1=w1326:u32)
          n518 = call-dynamic "Read stopping.vi"("error in (no error)"=w1338, "Channel in"=w1340) -> ("error out"=w1337:errorcluster, "stopping"=w1335:bool, "Channel out"=w1339:refnum<class "Channel.lvclass">)  [unwired: 7 in]
          n519 = Equal?(x=w1333, y=w1326) -> (x = y?=w1336:bool)
          n520 = call-dynamic "Write Channel.vi"("error in (no error)"=w1337, "Channel.lvclass"=w1339, "Acquisition in"=w1352) -> ("error out"=w1348:errorcluster, "Acquisition out"=w1349:refnum<class "Acquisition.lvclass">)  [unwired: 7 in]
          n521 = case shown="True" w1336 {
            tunnel: [w1361 w1405] -> w1350
            tunnel: w1349 -> [w1357 w1393]
            tunnel: w1351 -> [w1355 w1404]
            tunnel: w1348 -> [w1358 w1392]
            tunnel: [w1363 w1402] -> w1347
            tunnel: w1346 -> [w1364 w1400]
            tunnel: w1335 -> [_ w1398]
            tunnel: [w1362 w1403] -> w1334
            tunnel: w1333 -> [_ w1397]
            tunnel: w1327 -> [w1360 _]
            frame False {
              # "Aguardando iniciar exposição por 5s"
              n522 = local read "time 2"() -> (w1354:u32)
              n523 = Tick Count (ms)() -> (millisecond timer value=w1367:u32)
              n524 = Subtract(x=w1367, y=w1354) -> (x-y=w1366:u32)
              n525 = To Double Precision Float(number=w1366) -> (double precision float=w1365:dbl)
              n526 = Number To Decimal String(number=w1360) -> (decimal integer string=w1359:string)  [unwired: 1 in]
              n527 = Less?(x=5000.0, y=w1365) -> (x < y?=w1353:bool)
              n528 = case shown="False" w1353 {
                tunnel: w1364 -> [w1374 w1387]
                tunnel: [w1374 w1386] -> w1363
                tunnel: [w1369 w1383] -> w1362
                tunnel: w1358 -> [w1370 w1382]
                tunnel: w1357 -> [w1373 w1385]
                tunnel: [w1371 w1384] -> w1361
                tunnel: w1359 -> [_ w1379]
                tunnel: w1355 -> [w1372 _]
                frame False {
                  n529 = disable-structure shown="Enabled" {
                    disable-tunnel: w1372 -> [w1376 w1377]
                    disable-tunnel: [w1375 w1377] -> w1368
                    frame Disabled {
                      # "Volta para \nesperar ACTIVE."
                      n530 = Decrement(x=w1376) -> (x-1=w1375:u32)
                    }
                    frame Enabled {
                      # "OV20241108:\nNão volta mais pra 326.\nSó verifica CyclesDone."
                    }
                  }
                  n531 = call-dynamic "Write Acq_state.vi"("error in (no error)"=w1370, "Acq_state"=w1368, "Acquisition in"=w1373) -> ("error out"=w1369:errorcluster, "Acquisition out"=w1371:refnum<class "Acquisition.lvclass">)  [unwired: 7 in]
                }
                frame True {
                  n532 = Concatenate Strings("ERROR: Init Acquisition Timeout. HandleObservationAsync.vi - state 327. Channel: ", w1379) -> (w1378:string)
                  n533 = call-dynamic "Write Acq_state.vi"("error in (no error)"=w1382, "Acq_state"=u32 1, "Acquisition in"=w1385) -> ("error out"=w1383:errorcluster, "Acquisition out"=w1384:refnum<class "Acquisition.lvclass">)  [unwired: 7 in]
                  n534 = Bundle By Name(cluster=w1387, "Error Msg"=w1378) -> (w1386:refnum<class "S4GUI.lvclass">)
                }
              }
            }
            frame True {
              # "STOP?"
              # "Avançou o ciclo."
              n535 = call-dynamic "Read Channel.vi"("error in (no error)"=w1392, "Acquisition in"=w1393) -> ("error out"=w1391:errorcluster, "Channel.lvclass"=w1396:refnum<class "Channel.lvclass">, "Acquisition out"=w1394:refnum<class "Acquisition.lvclass">)  [unwired: 7 in]
              n536 = call-dynamic "Write PrevCyclesDone.vi"("error in (no error)"=w1391, "PrevCyclesDone"=w1397, "Channel in"=w1396) -> ("error out"=w1390:errorcluster, "Channel out"=w1395:refnum<class "Channel.lvclass">)  [unwired: 7 in]
              n537 = call-dynamic "Write Channel.vi"("error in (no error)"=w1390, "Channel.lvclass"=w1395, "Acquisition in"=w1394) -> ("error out"=w1388:errorcluster, "Acquisition out"=w1389:refnum<class "Acquisition.lvclass">)  [unwired: 7 in]
              n538 = case shown="False" w1398 {
                tunnel: w1404 -> [w1408 _]
                tunnel: [w1406 u32 0] -> w1399
                frame False {
                  n539 = Increment(x=w1408) -> (x+1=w1407:u32)
                  n540 = Increment(x=w1407) -> (x+1=w1406:u32)
                }
                frame True {
                }
              }
              n541 = call-dynamic "Write Acq_state.vi"("error in (no error)"=w1388, "Acq_state"=w1399, "Acquisition in"=w1389) -> ("error out"=w1403:errorcluster, "Acquisition out"=w1405:refnum<class "Acquisition.lvclass">)  [unwired: 7 in]
              n542 = Bundle By Name(cluster=w1400, "Error Msg"="") -> (w1402:refnum<class "S4GUI.lvclass">)
            }
          }
        }
        frame 328 {
          # "Dispara o comando para o dispositivo corrente."
          n543 = call "Read id.vi"("error in (no error)"=w1415, "Server in"=w1416) -> ("error out"=w1413:errorcluster, "id"=w1412:u32, "Server out"=w1414:refnum<class "Acquisition.lvclass">)  [unwired: 7 in]
          n544 = call-dynamic "Read Channel.vi"("error in (no error)"=w1413, "Acquisition in"=w1414) -> ("error out"=w1425:errorcluster, "Channel.lvclass"=w1426:refnum<class "Channel.lvclass">, "Acquisition out"=w1436:refnum<class "Acquisition.lvclass">)  [unwired: 7 in]
          n545 = Increment(x=w1412) -> (x+1=w1411:u32)
          n546 = call-dynamic "Read PrevCyclesDone.vi"("error in (no error)"=w1425, "Channel in"=w1426) -> ("error out"=w1428:errorcluster, "PrevCyclesDone"=w1427:u32, "Channel out"=w1429:refnum<class "Channel.lvclass">)  [unwired: 7 in]
          n547 = call-dynamic "Read CyclesDone.vi"("error in (no error)"=w1428, "Channel in"=w1429) -> ("error out"=w1422:errorcluster, "CyclesDone"=w1417:u32, "Channel out"=w1424:refnum<class "Channel.lvclass">)  [unwired: 7 in]
          n548 = Increment(x=w1427) -> (x+1=w1410:u32)
          n549 = call-dynamic "Read stopping.vi"("error in (no error)"=w1422, "Channel in"=w1424) -> ("error out"=w1421:errorcluster, "stopping"=w1419:bool, "Channel out"=w1423:refnum<class "Channel.lvclass">)  [unwired: 7 in]
          n550 = Equal?(x=w1417, y=w1410) -> (x = y?=w1420:bool)
          n551 = call-dynamic "Write Channel.vi"("error in (no error)"=w1421, "Channel.lvclass"=w1423, "Acquisition in"=w1436) -> ("error out"=w1432:errorcluster, "Acquisition out"=w1433:refnum<class "Acquisition.lvclass">)  [unwired: 7 in]
          n552 = case shown="False" w1420 {
            tunnel: [w1442 w1487] -> w1434
            tunnel: w1433 -> [w1454 w1475]
            tunnel: w1435 -> [_ w1486]
            tunnel: w1432 -> [w1453 w1474]
            tunnel: [w1446 w1484] -> w1431
            tunnel: w1430 -> [w1447 w1482]
            tunnel: w1419 -> [_ w1480]
            tunnel: [w1444 w1485] -> w1418
            tunnel: w1417 -> [_ w1479]
            tunnel: w1411 -> [w1441 _]
            frame False {
              n553 = Tick Count (ms)() -> (millisecond timer value=w1456:u32)
              n554 = local read "time307"() -> (w1455:u32)
              n555 = call-dynamic "GetCubeDuration.vi"("error in (no error)"=w1453, "Acquisition in"=w1454) -> ("error out"=w1445:errorcluster, "Acquisition out"=w1443:refnum<class "Acquisition.lvclass">, "CubeDuration"=w1439:dbl)  [unwired: 7 in]
              n556 = Subtract(x=w1456, y=w1455) -> (x-y=w1450:u32)
              n557 = Multiply(x=w1439, y=1000.0) -> (x*y=w1437:dbl)
              n558 = To Double Precision Float(number=w1450) -> (double precision float=w1448:dbl)
              n559 = Add(x=1000.0, y=w1437) -> (x+y=w1451:dbl)
              n560 = Number To Decimal String(number=w1441) -> (decimal integer string=w1440:string)  [unwired: 1 in]
              n561 = Less?(x=w1451, y=w1448) -> (x < y?=w1449:bool)
              n562 = case shown="True" w1449 {
                tunnel: w1447 -> [w1459 w1469]
                tunnel: [w1459 w1468] -> w1446
                tunnel: [w1458 w1465] -> w1444
                tunnel: w1445 -> [w1458 w1464]
                tunnel: w1443 -> [w1457 w1467]
                tunnel: [w1457 w1466] -> w1442
                tunnel: w1440 -> [_ w1461]
                frame False {
                }
                frame True {
                  n563 = Concatenate Strings("ERROR: Acquisition Timeout. HandleObservationAsync.vi - state 328. Channel: ", w1461) -> (w1460:string)
                  n564 = call-dynamic "Write Acq_state.vi"("error in (no error)"=w1464, "Acq_state"=u32 1, "Acquisition in"=w1467) -> ("error out"=w1465:errorcluster, "Acquisition out"=w1466:refnum<class "Acquisition.lvclass">)  [unwired: 7 in]
                  n565 = Bundle By Name(cluster=w1469, "Error Msg"=w1460) -> (w1468:refnum<class "S4GUI.lvclass">)
                }
              }
            }
            frame True {
              n566 = call-dynamic "Read Channel.vi"("error in (no error)"=w1474, "Acquisition in"=w1475) -> ("error out"=w1473:errorcluster, "Channel.lvclass"=w1478:refnum<class "Channel.lvclass">, "Acquisition out"=w1476:refnum<class "Acquisition.lvclass">)  [unwired: 7 in]
              n567 = call-dynamic "Write PrevCyclesDone.vi"("error in (no error)"=w1473, "PrevCyclesDone"=w1479, "Channel in"=w1478) -> ("error out"=w1472:errorcluster, "Channel out"=w1477:refnum<class "Channel.lvclass">)  [unwired: 7 in]
              n568 = call-dynamic "Write Channel.vi"("error in (no error)"=w1472, "Channel.lvclass"=w1477, "Acquisition in"=w1476) -> ("error out"=w1470:errorcluster, "Acquisition out"=w1471:refnum<class "Acquisition.lvclass">)  [unwired: 7 in]
              n569 = case shown="False" w1480 {
                tunnel: w1486 -> [w1489 _]
                tunnel: [w1488 u32 0] -> w1481
                frame False {
                  n570 = Increment(x=w1489) -> (x+1=w1488:u32)
                }
                frame True {
                }
              }
              n571 = call-dynamic "Write Acq_state.vi"("error in (no error)"=w1470, "Acq_state"=w1481, "Acquisition in"=w1471) -> ("error out"=w1485:errorcluster, "Acquisition out"=w1487:refnum<class "Acquisition.lvclass">)  [unwired: 7 in]
              n572 = Bundle By Name(cluster=w1482, "Error Msg"="") -> (w1484:refnum<class "S4GUI.lvclass">)
            }
          }
        }
        frame 329 {
          n573 = call-dynamic "Read Channel.vi"("error in (no error)"=w1508, "Acquisition in"=w1509) -> ("error out"=w1502:errorcluster, "Channel.lvclass"=w1507:refnum<class "Channel.lvclass">, "Acquisition out"=w1494:refnum<class "Acquisition.lvclass">)  [unwired: 7 in]
          n574 = call-dynamic "Read CyclesDone.vi"("error in (no error)"=w1502, "Channel in"=w1507) -> ("error out"=w1510:errorcluster, "CyclesDone"=w1505:u32, "Channel out"=w1511:refnum<class "Channel.lvclass">)  [unwired: 7 in]
          n575 = call-dynamic "Read ciclos.vi"("error in (no error)"=w1510, "Channel in"=w1511) -> ("error out"=w1501:errorcluster, "ciclos"=w1506:u32, "Channel out"=w1500:refnum<class "Channel.lvclass">)  [unwired: 7 in]
          n576 = Subtract(x=w1506, y=w1505) -> (x-y=w1512:u32)
          n577 = Greater Than 0?(x=w1512) -> (x > 0?=w1492:bool)
          n578 = call-dynamic "Read wait_expose.vi"("error in (no error)"=w1501, "Channel in"=w1500) -> ("error out"=w1496:errorcluster, "wait_expose"=w1499:bool)  [unwired: 7 in, 1 out]
          n579 = Select(t=u32 323, s=w1499, f=u32 325 ("t")) -> (s? t:f=w1491:u32)
          n580 = case shown="False" w1492 {
            tunnel: [u32 0 ("f") w1535] -> w1498
            tunnel: w1497 -> [w1529 w1533]
            tunnel: w1496 -> [w1523 w1534]
            tunnel: [w1519 w1534] -> w1495
            tunnel: [w1518 w1533] -> w1493
            tunnel: w1491 -> [_ w1535]
            frame False {
              # "20241108:\nPassa aqui também quando é polarimetria com 1 posicao. \nNeste caso, deve recarregar SEQ antes de encerrar; então recarrega sempre aqui."
              n581 = call "Read Instrument.lvclass.vi"("error in (no error)"=w1523, "S4ACS_GUI in"=w1529) -> ("error out"=w1530:errorcluster, "Instrument.lvclass"=w1531:refnum<class "Instrument.lvclass">, "S4ACS_GUI out"=w1528:refnum<class "S4GUI.lvclass">)  [unwired: 7 in]
              n582 = call "Read WPROT.vi"("error in (no error)"=w1530, "Instrument in"=w1531) -> ("error out"=w1521:errorcluster, "Opt_Selector.lvclass"=w1525:refnum<class "Opt_Selector.lvclass">, "Instrument out"=w1527:refnum<class "Instrument.lvclass">)  [unwired: 7 in]
              n583 = call-dynamic "Read sequencia_ant.vi"("error in (no error)"=w1521, "Opt_Selector in"=w1525) -> ("error out"=w1516:errorcluster, "sequencia_ant"=w1515:u16, "Opt_Selector out"=w1517:refnum<class "Opt_Selector.lvclass">)  [unwired: 7 in]
              n584 = call-dynamic "Write sequencia.vi"("error in (no error)"=w1516, "sequencia"=w1515, "Opt_Selector in"=w1517) -> ("error out"=w1520:errorcluster, "Opt_Selector out"=w1524:refnum<class "Opt_Selector.lvclass">)  [unwired: 7 in]
              n585 = call "Write WPROT.vi"("error in (no error)"=w1520, "Opt_Selector.lvclass"=w1524, "Instrument in"=w1527) -> ("error out"=w1522:errorcluster, "Instrument out"=w1526:refnum<class "Instrument.lvclass">)  [unwired: 7 in]
              n586 = call "Write Instrument.lvclass.vi"("error in (no error)"=w1522, "Instrument.lvclass"=w1526, "S4ACS_GUI in"=w1528) -> ("error out"=w1519:errorcluster, "S4ACS_GUI out"=w1518:refnum<class "S4GUI.lvclass">)  [unwired: 7 in]
            }
            frame True {
            }
          }
          n587 = call-dynamic "Write Acq_state.vi"("error in (no error)"=w1495, "Acq_state"=w1498, "Acquisition in"=w1494) -> ("error out"=w1513:errorcluster, "Acquisition out"=w1514:refnum<class "Acquisition.lvclass">)  [unwired: 7 in]
        }
        frame 1325 {
          n588 = disable-structure shown="Enabled" {
            disable-tunnel: w1541 -> [w1557 w1585]
            disable-tunnel: w1540 -> [w1556 w1584]
            disable-tunnel: [w1549 w1580] -> w1539
            disable-tunnel: [w1543 w1581] -> w1538
            disable-tunnel: w1536 -> [_ _]
            disable-tunnel: w1537 -> [_ w1579]
            frame Disabled {
              n589 = call-dynamic "Read Channel.vi"("error in (no error)"=w1556, "Acquisition in"=w1557) -> ("error out"=w1554:errorcluster, "Channel.lvclass"=w1555:refnum<class "Channel.lvclass">, "Acquisition out"=w1551:refnum<class "Acquisition.lvclass">)  [unwired: 7 in]
              n590 = call-dynamic "Read ciclos.vi"("error in (no error)"=w1554, "Channel in"=w1555) -> ("error out"=w1546:errorcluster, "ciclos"=w1553:u32, "Channel out"=w1547:refnum<class "Channel.lvclass">)  [unwired: 7 in]
              n591 = Decrement(x=w1553) -> (x-1=w1558:u32)
              n592 = Greater Than 0?(x=w1558) -> (x > 0?=w1562:bool)
              n593 = case shown="True" w1562 {
                selector: w1562 -> [w1564 w1566]
                tunnel: w1558 -> [_ w1565]
                tunnel: [w1564 w1566] -> w1561
                tunnel: [u32 0 w1565] -> w1552
                frame False {
                }
                frame True {
                }
              }
              n594 = call-dynamic "Write ciclos.vi"("error in (no error)"=w1546, "ciclos"=w1552, "Channel in"=w1547) -> ("error out"=w1545:errorcluster, "Channel out"=w1548:refnum<class "Channel.lvclass">)  [unwired: 7 in]
              n595 = call-dynamic "Write Channel.vi"("error in (no error)"=w1545, "Channel.lvclass"=w1548, "Acquisition in"=w1551) -> ("error out"=w1544:errorcluster, "Acquisition out"=w1550:refnum<class "Acquisition.lvclass">)  [unwired: 7 in]
              n596 = Select(t=u32 323, s=w1561, f=u32 0) -> (s? t:f=w1542:u32)
              n597 = call-dynamic "Write Acq_state.vi"("error in (no error)"=w1544, "Acq_state"=w1542, "Acquisition in"=w1550) -> ("error out"=w1543:errorcluster, "Acquisition out"=w1549:refnum<class "Acquisition.lvclass">)  [unwired: 7 in]
            }
            frame Enabled {
              n598 = call-dynamic "Read Channel.vi"("error in (no error)"=w1584, "Acquisition in"=w1585) -> ("error out"=w1575:errorcluster, "Channel.lvclass"=w1577:refnum<class "Channel.lvclass">, "Acquisition out"=w1586:refnum<class "Acquisition.lvclass">)  [unwired: 7 in]
              n599 = call-dynamic "Read PrevCyclesDone.vi"("error in (no error)"=w1575, "Channel in"=w1577) -> ("error out"=w1574:errorcluster, "PrevCyclesDone"=w1573:u32, "Channel out"=w1576:refnum<class "Channel.lvclass">)  [unwired: 7 in]
              n600 = call-dynamic "Read CyclesDone.vi"("error in (no error)"=w1574, "Channel in"=w1576) -> ("error out"=w1570:errorcluster, "CyclesDone"=w1582:u32, "Channel out"=w1572:refnum<class "Channel.lvclass">)  [unwired: 7 in]
              n601 = Greater?(x=w1582, y=w1573) -> (0:w1583:bool)
              n602 = case shown="True" w1583 {
                tunnel: w1582 -> [_ w1590]
                tunnel: w1579 -> [w1589 w1596]
                tunnel: [w1589 w1595] -> w1578
                tunnel: [w1588 w1593] -> w1571
                tunnel: w1572 -> [w1588 w1594]
                tunnel: w1570 -> [w1587 w1592]
                tunnel: [w1587 w1591] -> w1569
                frame False {
                }
                frame True {
                  n603 = call-dynamic "Write PrevCyclesDone.vi"("error in (no error)"=w1592, "PrevCyclesDone"=w1590, "Channel in"=w1594) -> ("error out"=w1591:errorcluster, "Channel out"=w1593:refnum<class "Channel.lvclass">)  [unwired: 7 in]
                  n604 = Increment(x=w1596) -> (x+1=w1595:u32)
                }
              }
              n605 = call-dynamic "Write Channel.vi"("error in (no error)"=w1569, "Channel.lvclass"=w1571, "Acquisition in"=w1586) -> ("error out"=w1568:errorcluster, "Acquisition out"=w1567:refnum<class "Acquisition.lvclass">)  [unwired: 7 in]
              n606 = call-dynamic "Write Acq_state.vi"("error in (no error)"=w1568, "Acq_state"=w1578, "Acquisition in"=w1567) -> ("error out"=w1581:errorcluster, "Acquisition out"=w1580:refnum<class "Acquisition.lvclass">)  [unwired: 7 in]
            }
          }
        }
        frame 1326 {
          n607 = call-dynamic "Read Channel.vi"("error in (no error)"=w1604, "Acquisition in"=w1605) -> ("error out"=w1600:errorcluster, "Channel.lvclass"=w1603:refnum<class "Channel.lvclass">, "Acquisition out"=w1601:refnum<class "Acquisition.lvclass">)  [unwired: 7 in]
          n608 = call-dynamic "Read CyclesDone.vi"("Channel in"=w1603) -> ("error out"=w1597:errorcluster, "CyclesDone"=w1598:u32, "Channel out"=w1602:refnum<class "Channel.lvclass">)  [unwired: 8 in]
          n609 = call-dynamic "Read ciclos.vi"("error in (no error)"=w1597, "Channel in"=w1602) -> ("ciclos"=w1599:u32)  [unwired: 7 in, 2 out]
          n610 = Unbundle By Name(w1610) -> ("mode EXPOSE"=w1609:bool)
          n611 = Subtract(x=w1599, y=w1598) -> (x-y=w1616:u32)
          n612 = Select(t=u32 323, s=w1609, f=u32 325 ("t")) -> (s? t:f=w1606:u32)
          n613 = Greater Than 0?(x=w1616) -> (x > 0?=w1615:bool)
          n614 = Select(t=w1606, s=w1615, f=u32 0) -> (s? t:f=w1613:u32)
          n615 = call-dynamic "Write Acq_state.vi"("error in (no error)"=w1600, "Acq_state"=w1613, "Acquisition in"=w1601) -> ("error out"=w1611:errorcluster, "Acquisition out"=w1612:refnum<class "Acquisition.lvclass">)  [unwired: 7 in]
        }
        frame 360 {
          w1622 = u32 0 ("cyclesDone")
          # "Inicia o Ticks com\nvalor do relogio atual"
          # "Espera até 40 x 0.25s (= 10s) para\nmecanismo entrar em READY"
          # "Busca próximo valor de foco..."
          n616 = flat-sequence {
            tunnel: w1625 -> [w1652]
            tunnel: [w1652] -> w1642
            frame #0 {
              n617 = Tick Count (ms)() -> (millisecond timer value=→"time7":u32)
            }
          }
          n618 = call-dynamic "Read TelFocus.lvclass.vi"("error in (no error)"=w1642, "S4GUI in"=w1626) -> ("error out"=w1650:errorcluster, "TelFocus.lvclass"=w1651:refnum<class "TelFocus.lvclass">, "S4GUI out"=w1649:refnum<class "S4GUI.lvclass">)  [unwired: 7 in]
          n619 = call-dynamic "GetNextFocus.vi"("error in (no error)"=w1650, "TelFocus in"=w1651) -> ("error out"=w1640:errorcluster, "TelFocus out"=w1641:refnum<class "TelFocus.lvclass">)  [unwired: 8 in]
          n620 = call-dynamic "Read SecMirror.lvclass.vi"("error in (no error)"=w1640, "TelFocus in"=w1641) -> ("error out"=w1627:errorcluster, "SecMirror.lvclass"=w1628:refnum<class "SecMirror.lvclass">, "TelFocus out"=w1644:refnum<class "TelFocus.lvclass">)  [unwired: 7 in]
          n621 = call-dynamic "Read State Machine.vi"("error in (no error)"=w1627, "Device in"=w1628) -> ("error out"=w1637:errorcluster, "State Machine.lvclass"=w1639:refnum<class "State Machine.lvclass">, "Device out"=w1636:refnum<class "SecMirror.lvclass">)  [unwired: 7 in]
          n622 = call "Next State.vi"("error in (no error)"=w1637, "New_State"=1, "State Machine in"=w1639) -> ("error out"=w1634:errorcluster, "State Machine out"=w1635:refnum<class "State Machine.lvclass">)  [unwired: 7 in]
          n623 = call-dynamic "Write Timer.vi"("error in (no error)"=w1634, "Timer"=u32 40, "State Machine in"=w1635) -> ("error out"=w1631:errorcluster, "State Machine out"=w1632:refnum<class "State Machine.lvclass">)  [unwired: 7 in]
          n624 = call-dynamic "Init Ticks2.vi"("error in (no error)"=w1631, "State Machine in"=w1632) -> ("error out"=w1630:errorcluster, "State Machine out"=w1629:refnum<class "State Machine.lvclass">)  [unwired: 8 in]
          n625 = call-dynamic "Write State Machine.vi"("error in (no error)"=w1630, "State Machine.lvclass"=w1629, "Device in"=w1636) -> ("error out"=w1643:errorcluster, "Device out"=w1645:refnum<class "SecMirror.lvclass">)  [unwired: 7 in]
          n626 = call-dynamic "Write SecMirror.lvclass.vi"("error in (no error)"=w1643, "SecMirror.lvclass"=w1645, "TelFocus in"=w1644) -> ("error out"=w1647:errorcluster, "TelFocus out"=w1646:refnum<class "TelFocus.lvclass">)  [unwired: 7 in]
          n627 = call-dynamic "Write TelFocus.lvclass.vi"("error in (no error)"=w1647, "TelFocus.lvclass"=w1646, "S4GUI in"=w1649) -> ("error out"=w1619:errorcluster, "S4GUI out"=w1648:refnum<class "S4GUI.lvclass">)  [unwired: 7 in]
          n628 = Bundle By Name(cluster=w1648, "cyclesDone"=w1622, "sequesDone"=w1622) -> (w1623:refnum<class "S4GUI.lvclass">)
          n629 = Increment(x=w1624) -> (x+1=w1618:u32)
          n630 = call-dynamic "Write Acq_state.vi"("error in (no error)"=w1619, "Acq_state"=w1618, "Acquisition in"=w1621) -> ("error out"=w1617:errorcluster, "Acquisition out"=w1620:refnum<class "Acquisition.lvclass">)  [unwired: 7 in]
        }
        frame 361 {
          # "Timeout= 25s + distancia do target (cada 1000um=1s)"
          # "Espera terminar o movimento do foco do 2ndario para disparar\n a aquisição do canal."
          n631 = flat-sequence {
            tunnel: w1674 -> [w1710]
            tunnel: [w1710] -> w1690
            frame #0 {
              n632 = Tick Count (ms)() -> (millisecond timer value=w1709:u32)
              "time 8" <- w1709
              n633 = local read "time7"() -> (w1708:u32)
              n634 = Subtract(x=w1709, y=w1708) -> (x-y=→"delay 78":u32)
            }
          }
          n635 = call-dynamic "Read TelFocus.lvclass.vi"("error in (no error)"=w1690, "S4GUI in"=w1675) -> ("error out"=w1699:errorcluster, "TelFocus.lvclass"=w1700:refnum<class "TelFocus.lvclass">, "S4GUI out"=w1696:refnum<class "S4GUI.lvclass">)  [unwired: 7 in]
          n636 = call-dynamic "Read SecMirror.lvclass.vi"("error in (no error)"=w1699, "TelFocus in"=w1700) -> ("error out"=w1663:errorcluster, "SecMirror.lvclass"=w1666:refnum<class "SecMirror.lvclass">, "TelFocus out"=w1698:refnum<class "TelFocus.lvclass">)  [unwired: 7 in]
          n637 = call-dynamic "Read position.vi"("error in (no error)"=w1663, "SecMirror in"=w1666) -> ("error out"=w1672:errorcluster, "position"=w1660:i32, "SecMirror out"=w1665:refnum<class "SecMirror.lvclass">)  [unwired: 7 in]
          n638 = call-dynamic "Read target.vi"("error in (no error)"=w1672, "SecMirror in"=w1665) -> ("error out"=w1662:errorcluster, "target"=w1671:i32, "SecMirror out"=w1664:refnum<class "SecMirror.lvclass">)  [unwired: 7 in]
          n639 = Subtract(x=w1671, y=w1660) -> (x-y=w1670:i32)
          n640 = Absolute Value(x=w1670) -> (abs(x)=w1668:i32)
          n641 = call-dynamic "Read State Machine.vi"("error in (no error)"=w1662, "Device in"=w1664) -> ("error out"=w1682:errorcluster, "State Machine.lvclass"=w1685:refnum<class "State Machine.lvclass">, "Device out"=w1693:refnum<class "SecMirror.lvclass">)  [unwired: 7 in]
          n642 = To Unsigned Long Integer(number=w1668) -> (unsigned 32bit integer=w1669:u32)
          n643 = Add(x=w1669, y=u32 25000 ("period")) -> (x+y=w1661:u32)
          n644 = call-dynamic "Verif Clock 2.vi"("error in (no error)"=w1682, "period (ms)"=w1661, "State Machine in"=w1685) -> ("error out"=w1681:errorcluster, "time elapsed"=→"time elapsed 2":u32, "State Machine out"=w1684:refnum<class "State Machine.lvclass">)  [unwired: 6 in]
          n645 = call-dynamic "Read Timeout 2.vi"("error in (no error)"=w1681, "State Machine in"=w1684) -> ("error out"=w1680:errorcluster, "Timeout 2"=w1686:bool, "State Machine out"=w1683:refnum<class "State Machine.lvclass">)  [unwired: 7 in]
          n646 = call-dynamic "Read State.vi"("error in (no error)"=w1680, "State Machine in"=w1683) -> ("error out"=w1688:errorcluster, "State"=w1691:i32, "State Machine out"=w1689:refnum<class "State Machine.lvclass">)  [unwired: 7 in]
          n647 = call-dynamic "Write State Machine.vi"("error in (no error)"=w1688, "State Machine.lvclass"=w1689, "Device in"=w1693) -> ("error out"=w1692:errorcluster, "Device out"=w1694:refnum<class "SecMirror.lvclass">)  [unwired: 7 in]
          n648 = call-dynamic "Write SecMirror.lvclass.vi"("error in (no error)"=w1692, "SecMirror.lvclass"=w1694, "TelFocus in"=w1698) -> ("error out"=w1695:errorcluster, "TelFocus out"=w1697:refnum<class "TelFocus.lvclass">)  [unwired: 7 in]
          n649 = call-dynamic "Write TelFocus.lvclass.vi"("error in (no error)"=w1695, "TelFocus.lvclass"=w1697, "S4GUI in"=w1696) -> ("error out"=w1657:errorcluster, "S4GUI out"=w1679:refnum<class "S4GUI.lvclass">)  [unwired: 7 in]
          n650 = Equal To 0?(x=w1691) -> (x = 0?=w1687:bool)
          n651 = case shown="True" w1686 {
            tunnel: w1673 -> [w1702 _]
            tunnel: [w1702 u32 0 ("Obs_state")] -> w1677
            tunnel: w1679 -> [w1701 w1706]
            tunnel: [w1701 w1705] -> w1659
            frame False {
            }
            frame True {
              n652 = Bundle By Name(cluster=w1706, "Error Msg"="ERROR: moving telescope focus timeout  (S4GUI:HandleObservationAsync.vi - state 361)") -> (w1705:refnum<class "S4GUI.lvclass">)
            }
          }
          n653 = Increment(x=w1677) -> (x+1=w1676:u32)
          n654 = Select(t=w1676, s=w1687, f=w1677) -> (s? t:f=w1654:u32)
          n655 = call-dynamic "Write Acq_state.vi"("error in (no error)"=w1657, "Acq_state"=w1654, "Acquisition in"=w1658) -> ("error out"=w1655:errorcluster, "Acquisition out"=w1656:refnum<class "Acquisition.lvclass">)  [unwired: 7 in]
        }
        frame 362 {
          # "Dispara o comando para o dispositivo corrente."
          n656 = call-dynamic "Read Channel.vi"("error in (no error)"=w1720, "Acquisition in"=w1721) -> ("error out"=w1727:errorcluster, "Channel.lvclass"=w1726:refnum<class "Channel.lvclass">, "Acquisition out"=w1731:refnum<class "Acquisition.lvclass">)  [unwired: 7 in]
          n657 = call-dynamic "Read State Machine.vi"("error in (no error)"=w1727, "Device in"=w1726) -> ("error out"=w1728:errorcluster, "State Machine.lvclass"=w1730:refnum<class "State Machine.lvclass">, "Device out"=w1724:refnum<class "Channel.lvclass">)  [unwired: 7 in]
          n658 = call "Next State.vi"("error in (no error)"=w1728, "New_State"=58, "State Machine in"=w1730) -> ("error out"=w1713:errorcluster, "State Machine out"=w1714:refnum<class "State Machine.lvclass">)  [unwired: 7 in]
          n659 = call-dynamic "Write State Machine.vi"("error in (no error)"=w1713, "State Machine.lvclass"=w1714, "Device in"=w1724) -> ("error out"=w1723:errorcluster, "Device out"=w1725:refnum<class "Channel.lvclass">)  [unwired: 7 in]
          n660 = Increment(x=w1722) -> (x+1=w1719:u32)
          n661 = call-dynamic "Write Channel.vi"("error in (no error)"=w1723, "Channel.lvclass"=w1725, "Acquisition in"=w1731) -> ("error out"=w1717:errorcluster, "Acquisition out"=w1716:refnum<class "Acquisition.lvclass">)  [unwired: 7 in]
          n662 = call-dynamic "Write Acq_state.vi"("error in (no error)"=w1717, "Acq_state"=w1719, "Acquisition in"=w1716) -> ("error out"=w1712:errorcluster, "Acquisition out"=w1715:refnum<class "Acquisition.lvclass">)  [unwired: 7 in]
          n663 = flat-sequence {
            tunnel: w1712 -> [w1732]
            tunnel: [w1732] -> w1711
            frame #0 {
              n664 = Tick Count (ms)() -> (millisecond timer value=→"time9":u32)
            }
          }
        }
        frame 363 {
          # "Espera terminar a execução do comando atual \nantes de ir ao proximo passo da Observação."
          n665 = call-dynamic "Read Channel.vi"("error in (no error)"=w1750, "Acquisition in"=w1751) -> ("error out"=w1743:errorcluster, "Channel.lvclass"=w1744:refnum<class "Channel.lvclass">, "Acquisition out"=w1759:refnum<class "Acquisition.lvclass">)  [unwired: 7 in]
          n666 = call-dynamic "Read wait_expose.vi"("error in (no error)"=w1743, "Channel in"=w1744) -> ("error out"=w1741:errorcluster, "wait_expose"=w1739:bool, "Channel out"=w1742:refnum<class "Channel.lvclass">)  [unwired: 7 in]
          n667 = call-dynamic "Read State Machine.vi"("error in (no error)"=w1741, "Device in"=w1742) -> ("error out"=w1753:errorcluster, "State Machine.lvclass"=w1755:refnum<class "State Machine.lvclass">, "Device out"=w1757:refnum<class "Channel.lvclass">)  [unwired: 7 in]
          n668 = call-dynamic "Read State.vi"("error in (no error)"=w1753, "State Machine in"=w1755) -> ("error out"=w1752:errorcluster, "State"=w1735:i32, "State Machine out"=w1754:refnum<class "State Machine.lvclass">)  [unwired: 7 in]
          n669 = call-dynamic "Write State Machine.vi"("error in (no error)"=w1752, "State Machine.lvclass"=w1754, "Device in"=w1757) -> ("error out"=w1756:errorcluster, "Device out"=w1758:refnum<class "Channel.lvclass">)  [unwired: 7 in]
          n670 = Equal To 0?(x=w1735) -> (x = 0?=w1734:bool)
          n671 = call-dynamic "Write Channel.vi"("error in (no error)"=w1756, "Channel.lvclass"=w1758, "Acquisition in"=w1759) -> ("error out"=w1737:errorcluster, "Acquisition out"=w1749:refnum<class "Acquisition.lvclass">)  [unwired: 7 in]
          n672 = Increment(x=w1745) -> (x+1=w1738:u32)
          n673 = Select(t=w1738, s=w1734, f=w1745) -> (s? t:f=w1748:u32)
          n674 = call-dynamic "Write Acq_state.vi"("error in (no error)"=w1737, "Acq_state"=w1748, "Acquisition in"=w1749) -> ("error out"=w1746:errorcluster, "Acquisition out"=w1747:refnum<class "Acquisition.lvclass">)  [unwired: 7 in]
          n675 = Bundle By Name(cluster=w1736, "mode EXPOSE"=w1739) -> (w1740:refnum<class "S4GUI.lvclass">)
        }
        frame 364 {
          n676 = flat-sequence {
            tunnel: [w1775] -> w1763
            tunnel: w1764 -> [w1775]
            tunnel: [w1770] -> w1760
            frame #0 {
              n677 = local read "time9"() -> (w1771:u32)
              n678 = Tick Count (ms)() -> (millisecond timer value=w1774:u32)
              "time 10" <- w1774
              n679 = Subtract(x=w1774, y=w1771) -> (x-y=w1773:u32)
              "delay 89" <- w1773
              n680 = Greater?(x=w1773, y=u32 2000) -> (0:w1770:bool)
            }
          }
          n681 = Increment(x=w1761) -> (x+1=w1768:u32)
          n682 = Select(t=w1768, s=w1760, f=w1761) -> (s? t:f=w1769:u32)
          n683 = call-dynamic "Write Acq_state.vi"("error in (no error)"=w1763, "Acq_state"=w1769, "Acquisition in"=w1762) -> ("error out"=w1765:errorcluster, "Acquisition out"=w1766:refnum<class "Acquisition.lvclass">)  [unwired: 7 in]
        }
        frame 365 {
          # "Dispara o comando para o dispositivo corrente."
          n684 = call-dynamic "Read Channel.vi"("error in (no error)"=w1784, "Acquisition in"=w1785) -> ("error out"=w1791:errorcluster, "Channel.lvclass"=w1790:refnum<class "Channel.lvclass">, "Acquisition out"=w1795:refnum<class "Acquisition.lvclass">)  [unwired: 7 in]
          n685 = call-dynamic "Read State Machine.vi"("error in (no error)"=w1791, "Device in"=w1790) -> ("error out"=w1792:errorcluster, "State Machine.lvclass"=w1794:refnum<class "State Machine.lvclass">, "Device out"=w1788:refnum<class "Channel.lvclass">)  [unwired: 7 in]
          n686 = call "Next State.vi"("error in (no error)"=w1792, "New_State"=50, "State Machine in"=w1794) -> ("error out"=w1776:errorcluster, "State Machine out"=w1777:refnum<class "State Machine.lvclass">)  [unwired: 7 in]
          n687 = call-dynamic "Write State Machine.vi"("error in (no error)"=w1776, "State Machine.lvclass"=w1777, "Device in"=w1788) -> ("error out"=w1787:errorcluster, "Device out"=w1789:refnum<class "Channel.lvclass">)  [unwired: 7 in]
          n688 = Increment(x=w1786) -> (x+1=w1783:u32)
          n689 = call-dynamic "Write Channel.vi"("error in (no error)"=w1787, "Channel.lvclass"=w1789, "Acquisition in"=w1795) -> ("error out"=w1781:errorcluster, "Acquisition out"=w1780:refnum<class "Acquisition.lvclass">)  [unwired: 7 in]
          n690 = call-dynamic "Write Acq_state.vi"("error in (no error)"=w1781, "Acq_state"=w1783, "Acquisition in"=w1780) -> ("error out"=w1778:errorcluster, "Acquisition out"=w1779:refnum<class "Acquisition.lvclass">)  [unwired: 7 in]
        }
        frame 366 {
          # "Espera terminar a execução do comando atual \nantes de ir ao proximo passo da Observação."
          n691 = call-dynamic "Read Channel.vi"("error in (no error)"=w1813, "Acquisition in"=w1814) -> ("error out"=w1803:errorcluster, "Channel.lvclass"=w1804:refnum<class "Channel.lvclass">, "Acquisition out"=w1822:refnum<class "Acquisition.lvclass">)  [unwired: 7 in]
          n692 = call-dynamic "Read wait_expose.vi"("error in (no error)"=w1803, "Channel in"=w1804) -> ("error out"=w1801:errorcluster, "wait_expose"=w1799:bool, "Channel out"=w1802:refnum<class "Channel.lvclass">)  [unwired: 7 in]
          n693 = call-dynamic "Read State Machine.vi"("error in (no error)"=w1801, "Device in"=w1802) -> ("error out"=w1816:errorcluster, "State Machine.lvclass"=w1818:refnum<class "State Machine.lvclass">, "Device out"=w1820:refnum<class "Channel.lvclass">)  [unwired: 7 in]
          n694 = call-dynamic "Read State.vi"("error in (no error)"=w1816, "State Machine in"=w1818) -> ("error out"=w1815:errorcluster, "State"=w1807:i32, "State Machine out"=w1817:refnum<class "State Machine.lvclass">)  [unwired: 7 in]
          n695 = call-dynamic "Write State Machine.vi"("error in (no error)"=w1815, "State Machine.lvclass"=w1817, "Device in"=w1820) -> ("error out"=w1819:errorcluster, "Device out"=w1821:refnum<class "Channel.lvclass">)  [unwired: 7 in]
          n696 = Greater?(x=w1807, y=53) -> (0:w1806:bool)
          n697 = call-dynamic "Write Channel.vi"("error in (no error)"=w1819, "Channel.lvclass"=w1821, "Acquisition in"=w1822) -> ("error out"=w1797:errorcluster, "Acquisition out"=w1812:refnum<class "Acquisition.lvclass">)  [unwired: 7 in]
          n698 = Increment(x=w1805) -> (x+1=w1798:u32)
          n699 = Select(t=w1798, s=w1806, f=w1805) -> (s? t:f=w1811:u32)
          n700 = call-dynamic "Write Acq_state.vi"("error in (no error)"=w1797, "Acq_state"=w1811, "Acquisition in"=w1812) -> ("error out"=w1809:errorcluster, "Acquisition out"=w1810:refnum<class "Acquisition.lvclass">)  [unwired: 7 in]
          n701 = Bundle By Name(cluster=w1796, "mode EXPOSE"=w1799) -> (w1800:refnum<class "S4GUI.lvclass">)
        }
        frame 367 {
          # "SEQS_DONE = 0,1,2,...,n,0,1,..."
          n702 = Unbundle By Name(w1823) -> ("sequesDone"=w1832:u32, "cyclesDone"=w1827:u32)
          n703 = call-dynamic "Read Channel.vi"("error in (no error)"=w1843, "Acquisition in"=w1844) -> ("error out"=w1835:errorcluster, "Channel.lvclass"=w1836:refnum<class "Channel.lvclass">, "Acquisition out"=w1845:refnum<class "Acquisition.lvclass">)  [unwired: 7 in]
          n704 = call-dynamic "Read CyclesDone.vi"("error in (no error)"=w1835, "Channel in"=w1836) -> ("error out"=w1837:errorcluster, "CyclesDone"=w1828:u32, "Channel out"=w1838:refnum<class "Channel.lvclass">)  [unwired: 7 in]
          n705 = call-dynamic "Read SequesDone.vi"("error in (no error)"=w1837, "Channel in"=w1838) -> ("error out"=w1833:errorcluster, "SequesDone"=w1829:u32, "Channel out"=w1834:refnum<class "Channel.lvclass">)  [unwired: 6 in, 1 out]
          n706 = Not Equal?(x=w1828, y=w1827) -> (x != y?=w1825:bool)
          n707 = Not Equal?(x=w1829, y=w1832) -> (x != y?=w1826:bool)
          n708 = call-dynamic "Write Channel.vi"("error in (no error)"=w1833, "Channel.lvclass"=w1834, "Acquisition in"=w1845) -> ("error out"=w1841:errorcluster, "Acquisition out"=w1842:refnum<class "Acquisition.lvclass">)  [unwired: 7 in]
          n709 = Or(x=w1826, y=w1825) -> (x .or. y?=w1824:bool)
          n710 = case shown="True" w1824 {
            tunnel: [w1846 w1847] -> w1831
            tunnel: w1830 -> [w1846 w1848]
            tunnel: w1829 -> [_ _]
            tunnel: w1828 -> [_ _]
            frame False {
            }
            frame True {
              n711 = Increment(x=w1848) -> (x+1=w1847:u32)
            }
          }
          n712 = call-dynamic "Write Acq_state.vi"("error in (no error)"=w1841, "Acq_state"=w1831, "Acquisition in"=w1842) -> ("error out"=w1839:errorcluster, "Acquisition out"=w1840:refnum<class "Acquisition.lvclass">)  [unwired: 7 in]
        }
        frame 368 {
          n713 = Unbundle By Name(w1856) -> ("TelFocus.lvclass"=w1858:refnum<class "TelFocus.lvclass">)
          n714 = call-dynamic "VerifSteps.vi"("error in (no error)"=w1855, "TelFocus in"=w1858) -> ("error out"=w1852:errorcluster, "continua?"=w1859:bool, "TelFocus out"=w1857:refnum<class "TelFocus.lvclass">)  [unwired: 7 in]
          n715 = Bundle By Name(cluster=w1856, "TelFocus.lvclass"=w1857) -> (w1851:refnum<class "S4GUI.lvclass">)
          n716 = Select(t=u32 360, s=w1859, f=u32 0) -> (s? t:f=w1853:u32)
          n717 = call-dynamic "Write Acq_state.vi"("error in (no error)"=w1852, "Acq_state"=w1853, "Acquisition in"=w1854) -> ("error out"=w1849:errorcluster, "Acquisition out"=w1850:refnum<class "Acquisition.lvclass">)  [unwired: 7 in]
        }
        frame 400 {
          # "Estado de \"Pause\": fica parado aqui até o botão START seja pressionado."
        }
        frame 500 {
          # "Espera terminar o envio de RESUME para todos os ACS."
          # "Estado de \"Pause\": fica parado aqui até o botão RESUME seja pressionado."
          n718 = call-dynamic "VerifyAcqIdle.vi"("error in (no error)"=w1866, "S4GUI in"=w1867) -> ("error out"=w1870:errorcluster, "idle"=w1872:bool, "S4GUI out"=w1871:refnum<class "S4GUI.lvclass">)  [unwired: 6 in, 1 out]
          n719 = case shown="True" w1872 {
            tunnel: w1871 -> [w1874 w1884]
            tunnel: [w1874 w1876] -> w1869
            tunnel: w1870 -> [w1873 w1883]
            tunnel: [w1873 w1877] -> w1868
            frame False {
            }
            frame True {
              n720 = call-dynamic "LoadPrevAcqRunState.vi"("error in (no error)"=w1883, "S4GUI in"=w1884) -> ("error out"=w1878:errorcluster, "S4GUI out"=w1879:refnum<class "S4GUI.lvclass">)  [unwired: 8 in]
              n721 = Tick Count (ms)() -> (millisecond timer value=w1875:u32)
              n722 = call-dynamic "Read Obs_prevstate.vi"("error in (no error)"=w1878, "S4ACS_GUI in"=w1879) -> ("error out"=w1882:errorcluster, "Obs_prevstate"=w1880:u32, "S4ACS_GUI out"=w1881:refnum<class "S4GUI.lvclass">)  [unwired: 7 in]
              n723 = local write "time307"(w1875) -> ()
              n724 = local write "time1"(w1875) -> ()
              n725 = call-dynamic "Write Obs_state.vi"("error in (no error)"=w1882, "Obs_state"=w1880, "S4ACS_GUI in"=w1881) -> ("error out"=w1877:errorcluster, "S4ACS_GUI out"=w1876:refnum<class "S4GUI.lvclass">)  [unwired: 7 in]
            }
          }
        }
      }
    }
    frame Error {
    }
  }
  "error out" <- w5
  "S4ACS_GUI out" <- w3
  "Acquisition.lvclass Out" <- w1
